vi "电池状态显示.vi"(0 "can卡类型":u8, 1 "设备索引号":u8, 2 "CAN端口":u8, 3 "VIC_Receive":refnum<vi>, 5 "主界面选项 3":enum32{"单选选项1", "单选选项2 2", "单选选项2 3", "单选选项2 4"}(ring)) -> ()   [LabVIEW 2013]
panel:
  out "辅助继电器B(heat)":u16(ring) items=["未闭合", "闭合", "故障", "保留"]
  out "辅助继电器A(fan)":u16(ring) items=["未闭合", "闭合", "故障", "保留"]
  out "标准CAN总线状态":u16(ring) caption="标定CAN模块状态"
  out "Life:":dbl
  out "从板个数":u8
  out "功率":dbl
  out "负绝缘":dbl
  out "正绝缘":dbl
  out "DO":string[](array[string])
  out "DI":string[](array[string])
  out "AI2":dbl
  out "AI1":dbl
  out "放电总安时":dbl
  out "充电总安时":dbl
  out "实际容量":dbl
  out "最大放电电流":dbl
  out "最大充电电流":dbl
  out "平均电流":dbl
  in  "板号":u8
  out "其它故障":string[](array[string])
  out "硬件故障":string[](array[string])
  out "电池系统故障":string[](array[string])
  out "电池故障":string[](array[string])
  out "电池信息":T1
  out "电池应用车型":string
  out "电池包产权标识 3":string
  out "电池包组号 3":string
  out "电池类型 3":string
  out "电池厂商":string
  out "电池生产日期":string
  out "电池充电次数":dbl
  out "电池放空次数 3":dbl
  out "电池充满次数":dbl
  out "电池包累计充电总安时 3":dbl
  out "电池包额定总电压":dbl
  out "电池包额定能量":dbl
  out "电池包额定容量":dbl
  out "电池包累计放电总安时 3":dbl
  out "电池并联 3":dbl
  out "电池串联 3":dbl
  in  "电池信息读取":bool
  out "时间":string
  out "07":dbl
  out "10":string[](array[string])
  out "F":dbl[](array[numeric])
  in  "充电均衡":u32(colorbox)=6618880
  in  "放电均衡":u32(colorbox)=16711680
  out "均衡信息":string[][](table)=[["第1串", "1", "单体检测其它故障", "第25串", "1", "单体检测其它故障", "第49串", "1", "单体检测其它故障", "第73串", "1", "单体检测其它故障", "第97串", "1", "单体检测其它故障", "第121串", "1", "单体检测其它故障", "第145串", "1", "单体检测其它故障", "第169串", "1", "单体检测其它故障", "第193串", "1", "单体检测其它故障", "第217串", "1", "单体检测其它故障", "第241串", "1", "单体检测其它故障", "第265串", "1", "单体检测其它故障", "第289串", "1", "单体检测其它故障", ""], ["第2串", "", "", "第26串", "", "", "第50串", "", "", "第74串", "", "", "第98串", "", "", "第122串", "", "", "第146串", "", "", "第170串", "", "", "第194串", "", "", "第218串", "", "", "第242串", "", "", "第266串", "", "", "第290串", "", "", ""], ["第3串", "", "", "第27串", "", "", "第51串", "", "", "第75串", "", "", "第99串", "", "", "第123串", "", "", "第147串", "", "", "第171串", "", "", "第195串", "", "", "第219串", "", "", "第243串", "", "", "第267串", "", "", "第291串", "", "", ""], ["第4串", "", "", "第28串", "", "", "第52串", "", "", "第76串", "", "", "第100串", "", "", "第124串", "", "", "第148串", "", "", "第172串", "", "", "第196串", "", "", "第220串", "", "", "第244串", "", "", "第268串", "", "", "第292串", "", "", ""], ["第5串", "", "", "第29串", "", "", "第53串", "", "", "第77串", "", "", "第101串", "", "", "第125串", "", "", "第149串", "", "", "第173串", "", "", "第197串", "", "", "第221串", "", "", "第245串", "", "", "第269串", "", "", "第293串", "", "", ""], ["第6串", "", "", "第30串", "", "", "第54串", "", "", "第78串", "", "", "第102串", "", "", "第126串", "", "", "第150串", "", "", "第174串", "", "", "第198串", "", "", "第222串", "", "", "第246串", "", "", "第270串", "", "", "第294串", "", "", ""], ["第7串", "", "", "第31串", "", "", "第55串", "", "", "第79串", "", "", "第103串", "", "", "第127串", "", "", "第151串", "", "", "第175串", "", "", "第199串", "", "", "第223串", "", "", "第247串", "", "", "第271串", "", "", "第295串", "", "", ""], ["第8串", "", "", "第32串", "", "", "第56串", "", "", "第80串", "", "", "第104串", "", "", "第128串", "", "", "第152串", "", "", "第176串", "", "", "第200串", "", "", "第224串", "", "", "第248串", "", "", "第272串", "", "", "第296串", "", "", ""], ["第9串", "", "", "第33串", "", "", "第57串", "", "", "第81串", "", "", "第105串", "", "", "第129串", "", "", "第153串", "", "", "第177串", "", "", "第201串", "", "", "第225串", "", "", "第249串", "", "", "第273串", "", "", "第297串", "", "", ""], ["第10串", "", "", "第34串", "", "", "第58串", "", "", "第82串", "", "", "第106串", "", "", "第130串", "", "", "第154串", "", "", "第178串", "", "", "第202串", "", "", "第226串", "", "", "第250串", "", "", "第274串", "", "", "第298串", "", "", ""], ["第11串", "", "", "第35串", "", "", "第59串", "", "", "第83串", "", "", "第107串", "", "", "第131串", "", "", "第155串", "", "", "第179串", "", "", "第203串", "", "", "第227串", "", "", "第251串", "", "", "第275串", "", "", "第299串", "", "", ""], ["第12串", "", "", "第36串", "", "", "第60串", "", "", "第84串", "", "", "第108串", "", "", "第132串", "", "", "第156串", "", "", "第180串", "", "", "第204串", "", "", "第228串", "", "", "第252串", "", "", "第276串", "", "", "第300串", "", "", ""], ["第13串", "", "", "第37串", "", "", "第61串", "", "", "第85串", "", "", "第109串", "", "", "第133串", "", "", "第157串", "", "", "第181串", "", "", "第205串", "", "", "第229串", "", "", "第253串", "", "", "第277串", "", "", "", "", "", ""], ["第14串", "", "", "第38串", "", "", "第62串", "", "", "第86串", "", "", "第110串", "", "", "第134串", "", "", "第158串", "", "", "第182串", "", "", "第206串", "", "", "第230串", "", "", "第254串", "", "", "第278串", "", "", "", "", "", ""], ["第15串", "", "", "第39串", "", "", "第63串", "", "", "第87串", "", "", "第111串", "", "", "第135串", "", "", "第159串", "", "", "第183串", "", "", "第207串", "", "", "第231串", "", "", "第255串", "", "", "第279串", "", "", "", "", "", ""], ["第16串", "", "", "第40串", "", "", "第64串", "", "", "第88串", "", "", "第112串", "", "", "第136串", "", "", "第160串", "", "", "第184串", "", "", "第208串", "", "", "第232串", "", "", "第256串", "", "", "第280串", "", "", "", "", "", ""], ["第17串", "", "", "第41串", "", "", "第65串", "", "", "第89串", "", "", "第113串", "", "", "第137串", "", "", "第161串", "", "", "第185串", "", "", "第209串", "", "", "第233串", "", "", "第257串", "", "", "第281串", "", "", "", "", "", ""], ["第18串", "", "", "第42串", "", "", "第66串", "", "", "第90串", "", "", "第114串", "", "", "第138串", "", "", "第162串", "", "", "第186串", "", "", "第210串", "", "", "第234串", "", "", "第258串", "", "", "第282串", "", "", "", "", "", ""], ["第19串", "", "", "第43串", "", "", "第67串", "", "", "第91串", "", "", "第115串", "", "", "第139串", "", "", "第163串", "", "", "第187串", "", "", "第211串", "", "", "第235串", "", "", "第259串", "", "", "第283串", "", "", "", "", "", ""], ["第20串", "", "", "第44串", "", "", "第68串", "", "", "第92串", "", "", "第116串", "", "", "第140串", "", "", "第164串", "", "", "第188串", "", "", "第212串", "", "", "第236串", "", "", "第260串", "", "", "第284串", "", "", "", "", "", ""], ["第21串", "", "", "第45串", "", "", "第69串", "", "", "第93串", "", "", "第117串", "", "", "第141串", "", "", "第165串", "", "", "第189串", "", "", "第213串", "", "", "第237串", "", "", "第261串", "", "", "第285串", "", "", "", "", "", ""], ["第22串", "", "", "第46串", "", "", "第70串", "", "", "第94串", "", "", "第118串", "", "", "第142串", "", "", "第166串", "", "", "第190串", "", "", "第214串", "", "", "第238串", "", "", "第262串", "", "", "第286串", "", "", "", "", "", ""], ["第23串", "", "", "第47串", "", "", "第71串", "", "", "第95串", "", "", "第119串", "", "", "第143串", "", "", "第167串", "", "", "第191串", "", "", "第215串", "", "", "第239串", "", "", "第263串", "", "", "第287串", "", "", "", "", "", ""], ["第24串", "", "", "第48串", "", "", "第72串", "", "", "第96串", "", "", "第120串", "", "", "第144串", "", "", "第168串", "", "", "第192串", "", "", "第216串", "", "", "第240串", "", "", "第264串", "", "", "第288串", "", "", "", "", "", ""]]
  out "SOC":string[][](table)=[["第1串", "", "", "第25串", "", "", "第49串", "", "", "第73串", "", "", "第97串", "", "", "第121串", "", "", "第145串", "", "", "第169串", "", "", "第193串", "", "", "第217串", "", "", "第241串", "", "", "第265串", "", "", "第289串", "", "", ""], ["第2串", "", "", "第26串", "", "", "第50串", "", "", "第74串", "", "", "第98串", "", "", "第122串", "", "", "第146串", "", "", "第170串", "", "", "第194串", "", "", "第218串", "", "", "第242串", "", "", "第266串", "", "", "第290串", "", "", ""], ["第3串", "", "", "第27串", "", "", "第51串", "", "", "第75串", "", "", "第99串", "", "", "第123串", "", "", "第147串", "", "", "第171串", "", "", "第195串", "", "", "第219串", "", "", "第243串", "", "", "第267串", "", "", "第291串", "", "", ""], ["第4串", "", "", "第28串", "", "", "第52串", "", "", "第76串", "", "", "第100串", "", "", "第124串", "", "", "第148串", "", "", "第172串", "", "", "第196串", "", "", "第220串", "", "", "第244串", "", "", "第268串", "", "", "第292串", "", "", ""], ["第5串", "", "", "第29串", "", "", "第53串", "", "", "第77串", "", "", "第101串", "", "", "第125串", "", "", "第149串", "", "", "第173串", "", "", "第197串", "", "", "第221串", "", "", "第245串", "", "", "第269串", "", "", "第293串", "", "", ""], ["第6串", "", "", "第30串", "", "", "第54串", "", "", "第78串", "", "", "第102串", "", "", "第126串", "", "", "第150串", "", "", "第174串", "", "", "第198串", "", "", "第222串", "", "", "第246串", "", "", "第270串", "", "", "第294串", "", "", ""], ["第7串", "", "", "第31串", "", "", "第55串", "", "", "第79串", "", "", "第103串", "", "", "第127串", "", "", "第151串", "", "", "第175串", "", "", "第199串", "", "", "第223串", "", "", "第247串", "", "", "第271串", "", "", "第295串", "", "", ""], ["第8串", "", "", "第32串", "", "", "第56串", "", "", "第80串", "", "", "第104串", "", "", "第128串", "", "", "第152串", "", "", "第176串", "", "", "第200串", "", "", "第224串", "", "", "第248串", "", "", "第272串", "", "", "第296串", "", "", ""], ["第9串", "", "", "第33串", "", "", "第57串", "", "", "第81串", "", "", "第105串", "", "", "第129串", "", "", "第153串", "", "", "第177串", "", "", "第201串", "", "", "第225串", "", "", "第249串", "", "", "第273串", "", "", "第297串", "", "", ""], ["第10串", "", "", "第34串", "", "", "第58串", "", "", "第82串", "", "", "第106串", "", "", "第130串", "", "", "第154串", "", "", "第178串", "", "", "第202串", "", "", "第226串", "", "", "第250串", "", "", "第274串", "", "", "第298串", "", "", ""], ["第11串", "", "", "第35串", "", "", "第59串", "", "", "第83串", "", "", "第107串", "", "", "第131串", "", "", "第155串", "", "", "第179串", "", "", "第203串", "", "", "第227串", "", "", "第251串", "", "", "第275串", "", "", "第299串", "", "", ""], ["第12串", "", "", "第36串", "", "", "第60串", "", "", "第84串", "", "", "第108串", "", "", "第132串", "", "", "第156串", "", "", "第180串", "", "", "第204串", "", "", "第228串", "", "", "第252串", "", "", "第276串", "", "", "第300串", "", "", ""], ["第13串", "", "", "第37串", "", "", "第61串", "", "", "第85串", "", "", "第109串", "", "", "第133串", "", "", "第157串", "", "", "第181串", "", "", "第205串", "", "", "第229串", "", "", "第253串", "", "", "第277串", "", "", "", "", "", ""], ["第14串", "", "", "第38串", "", "", "第62串", "", "", "第86串", "", "", "第110串", "", "", "第134串", "", "", "第158串", "", "", "第182串", "", "", "第206串", "", "", "第230串", "", "", "第254串", "", "", "第278串", "", "", "", "", "", ""], ["第15串", "", "", "第39串", "", "", "第63串", "", "", "第87串", "", "", "第111串", "", "", "第135串", "", "", "第159串", "", "", "第183串", "", "", "第207串", "", "", "第231串", "", "", "第255串", "", "", "第279串", "", "", "", "", "", ""], ["第16串", "", "", "第40串", "", "", "第64串", "", "", "第88串", "", "", "第112串", "", "", "第136串", "", "", "第160串", "", "", "第184串", "", "", "第208串", "", "", "第232串", "", "", "第256串", "", "", "第280串", "", "", "", "", "", ""], ["第17串", "", "", "第41串", "", "", "第65串", "", "", "第89串", "", "", "第113串", "", "", "第137串", "", "", "第161串", "", "", "第185串", "", "", "第209串", "", "", "第233串", "", "", "第257串", "", "", "第281串", "", "", "", "", "", ""], ["第18串", "", "", "第42串", "", "", "第66串", "", "", "第90串", "", "", "第114串", "", "", "第138串", "", "", "第162串", "", "", "第186串", "", "", "第210串", "", "", "第234串", "", "", "第258串", "", "", "第282串", "", "", "", "", "", ""], ["第19串", "", "", "第43串", "", "", "第67串", "", "", "第91串", "", "", "第115串", "", "", "第139串", "", "", "第163串", "", "", "第187串", "", "", "第211串", "", "", "第235串", "", "", "第259串", "", "", "第283串", "", "", "", "", "", ""], ["第20串", "", "", "第44串", "", "", "第68串", "", "", "第92串", "", "", "第116串", "", "", "第140串", "", "", "第164串", "", "", "第188串", "", "", "第212串", "", "", "第236串", "", "", "第260串", "", "", "第284串", "", "", "", "", "", ""], ["第21串", "", "", "第45串", "", "", "第69串", "", "", "第93串", "", "", "第117串", "", "", "第141串", "", "", "第165串", "", "", "第189串", "", "", "第213串", "", "", "第237串", "", "", "第261串", "", "", "第285串", "", "", "", "", "", ""], ["第22串", "", "", "第46串", "", "", "第70串", "", "", "第94串", "", "", "第118串", "", "", "第142串", "", "", "第166串", "", "", "第190串", "", "", "第214串", "", "", "第238串", "", "", "第262串", "", "", "第286串", "", "", "", "", "", ""], ["第23串", "", "", "第47串", "", "", "第71串", "", "", "第95串", "", "", "第119串", "", "", "第143串", "", "", "第167串", "", "", "第191串", "", "", "第215串", "", "", "第239串", "", "", "第263串", "", "", "第287串", "", "", "", "", "", ""], ["第24串", "", "", "第48串", "", "", "第72串", "", "", "第96串", "", "", "第120串", "", "", "第144串", "", "", "第168串", "", "", "第192串", "", "", "第216串", "", "", "第240串", "", "", "第264串", "", "", "第288串", "", "", "", "", "", ""]]
  out "内阻":string[][](table)=[["第1串", "", "", "第25串", "", "", "第49串", "", "", "第73串", "", "", "第97串", "", "", "第121串", "", "", "第145串", "", "", "第169串", "", "", "第193串", "", "", "第217串", "", "", "第241串", "", "", "第265串", "", "", "第289串", "", "", ""], ["第2串", "", "", "第26串", "", "", "第50串", "", "", "第74串", "", "", "第98串", "", "", "第122串", "", "", "第146串", "", "", "第170串", "", "", "第194串", "", "", "第218串", "", "", "第242串", "", "", "第266串", "", "", "第290串", "", "", ""], ["第3串", "", "", "第27串", "", "", "第51串", "", "", "第75串", "", "", "第99串", "", "", "第123串", "", "", "第147串", "", "", "第171串", "", "", "第195串", "", "", "第219串", "", "", "第243串", "", "", "第267串", "", "", "第291串", "", "", ""], ["第4串", "", "", "第28串", "", "", "第52串", "", "", "第76串", "", "", "第100串", "", "", "第124串", "", "", "第148串", "", "", "第172串", "", "", "第196串", "", "", "第220串", "", "", "第244串", "", "", "第268串", "", "", "第292串", "", "", ""], ["第5串", "", "", "第29串", "", "", "第53串", "", "", "第77串", "", "", "第101串", "", "", "第125串", "", "", "第149串", "", "", "第173串", "", "", "第197串", "", "", "第221串", "", "", "第245串", "", "", "第269串", "", "", "第293串", "", "", ""], ["第6串", "", "", "第30串", "", "", "第54串", "", "", "第78串", "", "", "第102串", "", "", "第126串", "", "", "第150串", "", "", "第174串", "", "", "第198串", "", "", "第222串", "", "", "第246串", "", "", "第270串", "", "", "第294串", "", "", ""], ["第7串", "", "", "第31串", "", "", "第55串", "", "", "第79串", "", "", "第103串", "", "", "第127串", "", "", "第151串", "", "", "第175串", "", "", "第199串", "", "", "第223串", "", "", "第247串", "", "", "第271串", "", "", "第295串", "", "", ""], ["第8串", "", "", "第32串", "", "", "第56串", "", "", "第80串", "", "", "第104串", "", "", "第128串", "", "", "第152串", "", "", "第176串", "", "", "第200串", "", "", "第224串", "", "", "第248串", "", "", "第272串", "", "", "第296串", "", "", ""], ["第9串", "", "", "第33串", "", "", "第57串", "", "", "第81串", "", "", "第105串", "", "", "第129串", "", "", "第153串", "", "", "第177串", "", "", "第201串", "", "", "第225串", "", "", "第249串", "", "", "第273串", "", "", "第297串", "", "", ""], ["第10串", "", "", "第34串", "", "", "第58串", "", "", "第82串", "", "", "第106串", "", "", "第130串", "", "", "第154串", "", "", "第178串", "", "", "第202串", "", "", "第226串", "", "", "第250串", "", "", "第274串", "", "", "第298串", "", "", ""], ["第11串", "", "", "第35串", "", "", "第59串", "", "", "第83串", "", "", "第107串", "", "", "第131串", "", "", "第155串", "", "", "第179串", "", "", "第203串", "", "", "第227串", "", "", "第251串", "", "", "第275串", "", "", "第299串", "", "", ""], ["第12串", "", "", "第36串", "", "", "第60串", "", "", "第84串", "", "", "第108串", "", "", "第132串", "", "", "第156串", "", "", "第180串", "", "", "第204串", "", "", "第228串", "", "", "第252串", "", "", "第276串", "", "", "第300串", "", "", ""], ["第13串", "", "", "第37串", "", "", "第61串", "", "", "第85串", "", "", "第109串", "", "", "第133串", "", "", "第157串", "", "", "第181串", "", "", "第205串", "", "", "第229串", "", "", "第253串", "", "", "第277串", "", "", "", "", "", ""], ["第14串", "", "", "第38串", "", "", "第62串", "", "", "第86串", "", "", "第110串", "", "", "第134串", "", "", "第158串", "", "", "第182串", "", "", "第206串", "", "", "第230串", "", "", "第254串", "", "", "第278串", "", "", "", "", "", ""], ["第15串", "", "", "第39串", "", "", "第63串", "", "", "第87串", "", "", "第111串", "", "", "第135串", "", "", "第159串", "", "", "第183串", "", "", "第207串", "", "", "第231串", "", "", "第255串", "", "", "第279串", "", "", "", "", "", ""], ["第16串", "", "", "第40串", "", "", "第64串", "", "", "第88串", "", "", "第112串", "", "", "第136串", "", "", "第160串", "", "", "第184串", "", "", "第208串", "", "", "第232串", "", "", "第256串", "", "", "第280串", "", "", "", "", "", ""], ["第17串", "", "", "第41串", "", "", "第65串", "", "", "第89串", "", "", "第113串", "", "", "第137串", "", "", "第161串", "", "", "第185串", "", "", "第209串", "", "", "第233串", "", "", "第257串", "", "", "第281串", "", "", "", "", "", ""], ["第18串", "", "", "第42串", "", "", "第66串", "", "", "第90串", "", "", "第114串", "", "", "第138串", "", "", "第162串", "", "", "第186串", "", "", "第210串", "", "", "第234串", "", "", "第258串", "", "", "第282串", "", "", "", "", "", ""], ["第19串", "", "", "第43串", "", "", "第67串", "", "", "第91串", "", "", "第115串", "", "", "第139串", "", "", "第163串", "", "", "第187串", "", "", "第211串", "", "", "第235串", "", "", "第259串", "", "", "第283串", "", "", "", "", "", ""], ["第20串", "", "", "第44串", "", "", "第68串", "", "", "第92串", "", "", "第116串", "", "", "第140串", "", "", "第164串", "", "", "第188串", "", "", "第212串", "", "", "第236串", "", "", "第260串", "", "", "第284串", "", "", "", "", "", ""], ["第21串", "", "", "第45串", "", "", "第69串", "", "", "第93串", "", "", "第117串", "", "", "第141串", "", "", "第165串", "", "", "第189串", "", "", "第213串", "", "", "第237串", "", "", "第261串", "", "", "第285串", "", "", "", "", "", ""], ["第22串", "", "", "第46串", "", "", "第70串", "", "", "第94串", "", "", "第118串", "", "", "第142串", "", "", "第166串", "", "", "第190串", "", "", "第214串", "", "", "第238串", "", "", "第262串", "", "", "第286串", "", "", "", "", "", ""], ["第23串", "", "", "第47串", "", "", "第71串", "", "", "第95串", "", "", "第119串", "", "", "第143串", "", "", "第167串", "", "", "第191串", "", "", "第215串", "", "", "第239串", "", "", "第263串", "", "", "第287串", "", "", "", "", "", ""], ["第24串", "", "", "第48串", "", "", "第72串", "", "", "第96串", "", "", "第120串", "", "", "第144串", "", "", "第168串", "", "", "第192串", "", "", "第216串", "", "", "第240串", "", "", "第264串", "", "", "第288串", "", "", "", "", "", ""]]
  out "温度表格":string[][](table)=[["第1串", "", "", "第25串", "", "", "第49串", "", "", "第73串", "", "", "第97串", "", "", "第121串", "", "", "第145串", "", "", "第169串", "", "", "第193串", "", "", "第217串", "", "", "第241串", "", "", "第265串", "", "", "第289串", "", "", ""], ["第2串", "", "", "第26串", "", "", "第50串", "", "", "第74串", "", "", "第98串", "", "", "第122串", "", "", "第146串", "", "", "第170串", "", "", "第194串", "", "", "第218串", "", "", "第242串", "", "", "第266串", "", "", "第290串", "", "", ""], ["第3串", "", "", "第27串", "", "", "第51串", "", "", "第75串", "", "", "第99串", "", "", "第123串", "", "", "第147串", "", "", "第171串", "", "", "第195串", "", "", "第219串", "", "", "第243串", "", "", "第267串", "", "", "第291串", "", "", ""], ["第4串", "", "", "第28串", "", "", "第52串", "", "", "第76串", "", "", "第100串", "", "", "第124串", "", "", "第148串", "", "", "第172串", "", "", "第196串", "", "", "第220串", "", "", "第244串", "", "", "第268串", "", "", "第292串", "", "", ""], ["第5串", "", "", "第29串", "", "", "第53串", "", "", "第77串", "", "", "第101串", "", "", "第125串", "", "", "第149串", "", "", "第173串", "", "", "第197串", "", "", "第221串", "", "", "第245串", "", "", "第269串", "", "", "第293串", "", "", ""], ["第6串", "", "", "第30串", "", "", "第54串", "", "", "第78串", "", "", "第102串", "", "", "第126串", "", "", "第150串", "", "", "第174串", "", "", "第198串", "", "", "第222串", "", "", "第246串", "", "", "第270串", "", "", "第294串", "", "", ""], ["第7串", "", "", "第31串", "", "", "第55串", "", "", "第79串", "", "", "第103串", "", "", "第127串", "", "", "第151串", "", "", "第175串", "", "", "第199串", "", "", "第223串", "", "", "第247串", "", "", "第271串", "", "", "第295串", "", "", ""], ["第8串", "", "", "第32串", "", "", "第56串", "", "", "第80串", "", "", "第104串", "", "", "第128串", "", "", "第152串", "", "", "第176串", "", "", "第200串", "", "", "第224串", "", "", "第248串", "", "", "第272串", "", "", "第296串", "", "", ""], ["第9串", "", "", "第33串", "", "", "第57串", "", "", "第81串", "", "", "第105串", "", "", "第129串", "", "", "第153串", "", "", "第177串", "", "", "第201串", "", "", "第225串", "", "", "第249串", "", "", "第273串", "", "", "第297串", "", "", ""], ["第10串", "", "", "第34串", "", "", "第58串", "", "", "第82串", "", "", "第106串", "", "", "第130串", "", "", "第154串", "", "", "第178串", "", "", "第202串", "", "", "第226串", "", "", "第250串", "", "", "第274串", "", "", "第298串", "", "", ""], ["第11串", "", "", "第35串", "", "", "第59串", "", "", "第83串", "", "", "第107串", "", "", "第131串", "", "", "第155串", "", "", "第179串", "", "", "第203串", "", "", "第227串", "", "", "第251串", "", "", "第275串", "", "", "第299串", "", "", ""], ["第12串", "", "", "第36串", "", "", "第60串", "", "", "第84串", "", "", "第108串", "", "", "第132串", "", "", "第156串", "", "", "第180串", "", "", "第204串", "", "", "第228串", "", "", "第252串", "", "", "第276串", "", "", "第300串", "", "", ""], ["第13串", "", "", "第37串", "", "", "第61串", "", "", "第85串", "", "", "第109串", "", "", "第133串", "", "", "第157串", "", "", "第181串", "", "", "第205串", "", "", "第229串", "", "", "第253串", "", "", "第277串", "", "", "", "", "", ""], ["第14串", "", "", "第38串", "", "", "第62串", "", "", "第86串", "", "", "第110串", "", "", "第134串", "", "", "第158串", "", "", "第182串", "", "", "第206串", "", "", "第230串", "", "", "第254串", "", "", "第278串", "", "", "", "", "", ""], ["第15串", "", "", "第39串", "", "", "第63串", "", "", "第87串", "", "", "第111串", "", "", "第135串", "", "", "第159串", "", "", "第183串", "", "", "第207串", "", "", "第231串", "", "", "第255串", "", "", "第279串", "", "", "", "", "", ""], ["第16串", "", "", "第40串", "", "", "第64串", "", "", "第88串", "", "", "第112串", "", "", "第136串", "", "", "第160串", "", "", "第184串", "", "", "第208串", "", "", "第232串", "", "", "第256串", "", "", "第280串", "", "", "", "", "", ""], ["第17串", "", "", "第41串", "", "", "第65串", "", "", "第89串", "", "", "第113串", "", "", "第137串", "", "", "第161串", "", "", "第185串", "", "", "第209串", "", "", "第233串", "", "", "第257串", "", "", "第281串", "", "", "", "", "", ""], ["第18串", "", "", "第42串", "", "", "第66串", "", "", "第90串", "", "", "第114串", "", "", "第138串", "", "", "第162串", "", "", "第186串", "", "", "第210串", "", "", "第234串", "", "", "第258串", "", "", "第282串", "", "", "", "", "", ""], ["第19串", "", "", "第43串", "", "", "第67串", "", "", "第91串", "", "", "第115串", "", "", "第139串", "", "", "第163串", "", "", "第187串", "", "", "第211串", "", "", "第235串", "", "", "第259串", "", "", "第283串", "", "", "", "", "", ""], ["第20串", "", "", "第44串", "", "", "第68串", "", "", "第92串", "", "", "第116串", "", "", "第140串", "", "", "第164串", "", "", "第188串", "", "", "第212串", "", "", "第236串", "", "", "第260串", "", "", "第284串", "", "", "", "", "", ""], ["第21串", "", "", "第45串", "", "", "第69串", "", "", "第93串", "", "", "第117串", "", "", "第141串", "", "", "第165串", "", "", "第189串", "", "", "第213串", "", "", "第237串", "", "", "第261串", "", "", "第285串", "", "", "", "", "", ""], ["第22串", "", "", "第46串", "", "", "第70串", "", "", "第94串", "", "", "第118串", "", "", "第142串", "", "", "第166串", "", "", "第190串", "", "", "第214串", "", "", "第238串", "", "", "第262串", "", "", "第286串", "", "", "", "", "", ""], ["第23串", "", "", "第47串", "", "", "第71串", "", "", "第95串", "", "", "第119串", "", "", "第143串", "", "", "第167串", "", "", "第191串", "", "", "第215串", "", "", "第239串", "", "", "第263串", "", "", "第287串", "", "", "", "", "", ""], ["第24串", "", "", "第48串", "", "", "第72串", "", "", "第96串", "", "", "第120串", "", "", "第144串", "", "", "第168串", "", "", "第192串", "", "", "第216串", "", "", "第240串", "", "", "第264串", "", "", "第288串", "", "", "", "", "", ""]]
  out "电压表格控件":string[][](table)=[["第1串", "", "", "第25串", "", "", "第49串", "", "", "第73串", "", "", "第97串", "", "", "第121串", "", "", "第145串", "", "", "第169串", "", "", "第193串", "", "", "第217串", "", "", "第241串", "", "", "第265串", "", "", "第289串", "", "", ""], ["第2串", "", "", "第26串", "", "", "第50串", "", "", "第74串", "", "", "第98串", "", "", "第122串", "", "", "第146串", "", "", "第170串", "", "", "第194串", "", "", "第218串", "", "", "第242串", "", "", "第266串", "", "", "第290串", "", "", ""], ["第3串", "", "", "第27串", "", "", "第51串", "", "", "第75串", "", "", "第99串", "", "", "第123串", "", "", "第147串", "", "", "第171串", "", "", "第195串", "", "", "第219串", "", "", "第243串", "", "", "第267串", "", "", "第291串", "", "", ""], ["第4串", "", "", "第28串", "", "", "第52串", "", "", "第76串", "", "", "第100串", "", "", "第124串", "", "", "第148串", "", "", "第172串", "", "", "第196串", "", "", "第220串", "", "", "第244串", "", "", "第268串", "", "", "第292串", "", "", ""], ["第5串", "", "", "第29串", "", "", "第53串", "", "", "第77串", "", "", "第101串", "", "", "第125串", "", "", "第149串", "", "", "第173串", "", "", "第197串", "", "", "第221串", "", "", "第245串", "", "", "第269串", "", "", "第293串", "", "", ""], ["第6串", "", "", "第30串", "", "", "第54串", "", "", "第78串", "", "", "第102串", "", "", "第126串", "", "", "第150串", "", "", "第174串", "", "", "第198串", "", "", "第222串", "", "", "第246串", "", "", "第270串", "", "", "第294串", "", "", ""], ["第7串", "", "", "第31串", "", "", "第55串", "", "", "第79串", "", "", "第103串", "", "", "第127串", "", "", "第151串", "", "", "第175串", "", "", "第199串", "", "", "第223串", "", "", "第247串", "", "", "第271串", "", "", "第295串", "", "", ""], ["第8串", "", "", "第32串", "", "", "第56串", "", "", "第80串", "", "", "第104串", "", "", "第128串", "", "", "第152串", "", "", "第176串", "", "", "第200串", "", "", "第224串", "", "", "第248串", "", "", "第272串", "", "", "第296串", "", "", ""], ["第9串", "", "", "第33串", "", "", "第57串", "", "", "第81串", "", "", "第105串", "", "", "第129串", "", "", "第153串", "", "", "第177串", "", "", "第201串", "", "", "第225串", "", "", "第249串", "", "", "第273串", "", "", "第297串", "", "", ""], ["第10串", "", "", "第34串", "", "", "第58串", "", "", "第82串", "", "", "第106串", "", "", "第130串", "", "", "第154串", "", "", "第178串", "", "", "第202串", "", "", "第226串", "", "", "第250串", "", "", "第274串", "", "", "第298串", "", "", ""], ["第11串", "", "", "第35串", "", "", "第59串", "", "", "第83串", "", "", "第107串", "", "", "第131串", "", "", "第155串", "", "", "第179串", "", "", "第203串", "", "", "第227串", "", "", "第251串", "", "", "第275串", "", "", "第299串", "", "", ""], ["第12串", "", "", "第36串", "", "", "第60串", "", "", "第84串", "", "", "第108串", "", "", "第132串", "", "", "第156串", "", "", "第180串", "", "", "第204串", "", "", "第228串", "", "", "第252串", "", "", "第276串", "", "", "第300串", "", "", ""], ["第13串", "", "", "第37串", "", "", "第61串", "", "", "第85串", "", "", "第109串", "", "", "第133串", "", "", "第157串", "", "", "第181串", "", "", "第205串", "", "", "第229串", "", "", "第253串", "", "", "第277串", "", "", "", "", "", ""], ["第14串", "", "", "第38串", "", "", "第62串", "", "", "第86串", "", "", "第110串", "", "", "第134串", "", "", "第158串", "", "", "第182串", "", "", "第206串", "", "", "第230串", "", "", "第254串", "", "", "第278串", "", "", "", "", "", ""], ["第15串", "", "", "第39串", "", "", "第63串", "", "", "第87串", "", "", "第111串", "", "", "第135串", "", "", "第159串", "", "", "第183串", "", "", "第207串", "", "", "第231串", "", "", "第255串", "", "", "第279串", "", "", "", "", "", ""], ["第16串", "", "", "第40串", "", "", "第64串", "", "", "第88串", "", "", "第112串", "", "", "第136串", "", "", "第160串", "", "", "第184串", "", "", "第208串", "", "", "第232串", "", "", "第256串", "", "", "第280串", "", "", "", "", "", ""], ["第17串", "", "", "第41串", "", "", "第65串", "", "", "第89串", "", "", "第113串", "", "", "第137串", "", "", "第161串", "", "", "第185串", "", "", "第209串", "", "", "第233串", "", "", "第257串", "", "", "第281串", "", "", "", "", "", ""], ["第18串", "", "", "第42串", "", "", "第66串", "", "", "第90串", "", "", "第114串", "", "", "第138串", "", "", "第162串", "", "", "第186串", "", "", "第210串", "", "", "第234串", "", "", "第258串", "", "", "第282串", "", "", "", "", "", ""], ["第19串", "", "", "第43串", "", "", "第67串", "", "", "第91串", "", "", "第115串", "", "", "第139串", "", "", "第163串", "", "", "第187串", "", "", "第211串", "", "", "第235串", "", "", "第259串", "", "", "第283串", "", "", "", "", "", ""], ["第20串", "", "", "第44串", "", "", "第68串", "", "", "第92串", "", "", "第116串", "", "", "第140串", "", "", "第164串", "", "", "第188串", "", "", "第212串", "", "", "第236串", "", "", "第260串", "", "", "第284串", "", "", "", "", "", ""], ["第21串", "", "", "第45串", "", "", "第69串", "", "", "第93串", "", "", "第117串", "", "", "第141串", "", "", "第165串", "", "", "第189串", "", "", "第213串", "", "", "第237串", "", "", "第261串", "", "", "第285串", "", "", "", "", "", ""], ["第22串", "", "", "第46串", "", "", "第70串", "", "", "第94串", "", "", "第118串", "", "", "第142串", "", "", "第166串", "", "", "第190串", "", "", "第214串", "", "", "第238串", "", "", "第262串", "", "", "第286串", "", "", "", "", "", ""], ["第23串", "", "", "第47串", "", "", "第71串", "", "", "第95串", "", "", "第119串", "", "", "第143串", "", "", "第167串", "", "", "第191串", "", "", "第215串", "", "", "第239串", "", "", "第263串", "", "", "第287串", "", "", "", "", "", ""], ["第24串", "", "", "第48串", "", "", "第72串", "", "", "第96串", "", "", "第120串", "", "", "第144串", "", "", "第168串", "", "", "第192串", "", "", "第216串", "", "", "第240串", "", "", "第264串", "", "", "第288串", "", "", "", "", "", ""]]
  out "故障定义":string[][](table)=[["电池故障定义", "状态", "BMS故障定义", "状态", "电池系统故障定义", "状态", "其他故障定义", "状态"], ["总电压过压", "失效", "电压检测模块故障", "保留", "正接触器粘连", "保留", "下电故障", "二级故障"], ["总电压欠压", "失效", "温度检测模块故障", "保留", "正接触器不能吸合", "保留", "供电电源过压", "二级故障"], ["单体电压过压", "失效", "电池检测模块故障", "保留", "带电流切断总正继电器故障", "保留", "供电电源欠压", "二级故障"], ["单体电压欠压", "失效", "绝缘检测模块故障", "正常", "带电流切断总负继电器故障", "保留", "风机继电器粘连", "二级故障"], ["单箱压差过大", "失效", "内总电压检测模块故障", "保留", "负接触器粘连", "保留", "风机继电器不能吸合", "失效"], ["整组压差过大", "失效", "外总电压检测模块故障", "保留", "负接触器不能吸合", "保留", "液位传感器", "失效"], ["单箱温差过大", "失效", "系统外扩时钟模块故障", "正常", "预充电接触器粘连", "保留", "压力传感器报警", "失效"], ["整组温差过大", "失效", "CPU内部EE故障", "保留", "预充电接触器不能吸合", "保留", "碰撞传感器报警", "失效"], ["温度过高", "失效", "EE存储器故障", "保留", "DC/DC继电器粘连", "保留", "湿度传感器报警", ""], ["温度过低", "失效", "45db041存储器故障", "保留", "DC/DC继电器不能吸合", "保留", "烟雾报警器故障", ""], ["充电电流过高", "失效", "CPU内部flash存储器故障", "保留", "高压互锁失效", "保留", "保险丝温度高于上限值", ""], ["放电电流过高", "失效", "CPU故障", "保留", "高压互锁异常", "保留", "保险丝损坏", ""], ["回馈过电流", "失效", "CAN4通信模块故障", "保留", "充电接触器粘连", "保留", "绝缘故障偏正极", "失效"], ["SOC过高", "正常", "CAN0通信模块故障", "保留", "充电接触器不能吸合", "保留", "绝缘故障偏负极", "失效"], ["SOC过低", "失效", "CAN1通信模块故障", "正常", "带电流切断充电继电器故障", "保留", "绝缘故障中间侧", "失效"], ["单体SOC过高", "失效", "CAN2通信模块故障", "正常", "极注温度高于上限值", "保留", "绝缘故障(未分位置", "失效"], ["单体SOC过低", "失效", "CAN3通信模块故障", "保留", "预充电故障", "保留", "", ""], ["单体SOC不一致", "失效", "以太网通信模块故障", "保留", "风机堵路", "正常", "", ""], ["箱间平均电压不一致", "失效", "RS232通信模块故障", "保留", "风机开路", "正常", "", ""], ["电池组号不一致", "失效", "RS485通信模块故障", "保留", "加热不能开启", "正常", "", ""], ["单体电池内阻大", "失效", "充电均衡模块故障", "正常", "加热不能关闭", "保留", "", ""], ["单体电池内阻不一致", "失效", "放电均衡模块故障", "正常", "加热器温度高于上限值", "保留", "", ""], ["电池组内阻大", "失效", "WH计量模块故障", "正常", "进风口温度过高", "保留", "", ""], ["箱间SOC不一致", "失效", "软件故障", "正常", "进风口,出风口温差故障", "保留", "", ""], ["电池厂家不一致", "失效", "AI自检异常", "正常", "出风口温度过高", "保留", "", ""], ["电池类型不一致", "失效", "AO自检异常", "正常", "出风口过低", "保留", "", ""], ["电池内短路", "失效", "DI模块故障", "正常", "", "", "", ""], ["整体电池容量低", "失效", "DO模块故障", "正常", "", "", "", ""], ["单体电池容量低", "失效", "", "", "", "", "", ""], ["单体电池容量不一致", "", "", "", "", "", "", ""], ["", "", "", "", "", "", "", ""], ["", "", "", "", "", "", "", ""]] caption="故障信息"
  out "BMS信息":string[][](table)=[["参数名称", "周期刷新", "参数名称", "周期刷新", "参数名称", "单次刷新"], ["温度检测模块状态", "", "BMS唤醒模式", "", "软件版本号", ""], ["电池充电均衡模块状态", "", "Key_on", "", "平台版本号", ""], ["电池放电均衡模块状态", "", "慢充", "", "各功能模块版本号", ""], ["电压检测模式状态", "", "快充", "", "内部CAN通讯协议版本", ""], ["绝缘检测模块状态", "", "自唤醒", "", "硬件版本号", ""], ["电池检测模块状态", "", "CAN唤醒", "", "温度传感器类型", ""], ["内部总电压检测模块状态", "", "自保持输出状态", "", "电流传感器类型", ""], ["外部总电压检测模块状态", "", "内部CAN总线状态", "", "历史记录起始页", ""], ["系统时钟状态", "", "充电CAN总线状态", "", "历史记录终止页", ""], ["Flash存储器状态", "", "整车CAN总线状态", "", "故障记录起始页", ""], ["外部EE存储器状态", "", "BMS上次停机时间", "", "故障记录终止页", ""], ["内部EE存储器状态", "", "BMS当前系统时间", "", "", ""], ["BMS供电电源状态", "", "", "", "", ""], ["BMS钥匙信号状态", "", "", "", "", ""], ["BMS供电电源电压", "", "", "", "", ""], ["内网总线负载率", "", "", "", "", ""], ["", "", "", "", "", ""], ["", "", "", "", "", ""], ["", "", "", "", "", ""], ["", "", "", "", "", ""], ["", "", "", "", "", ""]] caption="BMS信息界面"
  in  "主界面选项":enum32{"单选选项1", "单选选项2 2", "单选选项2 3", "单选选项2 4"}(radio)
  out "充电信息":string[][](table)=[["参数名称", "周期刷新", "参数名称", "周期刷新", "参数名称", ""], ["充电允许控制状态", "禁止充电", "BMS停止充电原因", "2345", "累计充电时间", ""], ["快/慢充电信号状态", "消失", "达到所需单体电压设定值", "0", "剩余充电时间", ""], ["交流充电接口容量", "32A", "达到总电压设定值", "300", "最大允许充电总电压", ""], ["充电接口连接状态", "不连接", "达到所需SOC目标值", "3.7", "最大允许充电单体电压", ""], ["充电状态", "空闲", "BMS有硬件故障", "670", "最大允许充电电流", ""], ["充电阶段", "", "系统存在绝缘故障", "3500", "最小允许充电电流", ""], ["充电机状态", "", "单体电压超过上限", "0", "充电电流步长", ""], ["充电机停止充电原因", "", "单体电压过低", "23000", "最大允许充电温度", ""], ["达到充电机设定条件中止", "", "总电压超过上限", "300", "充电机输出电压", ""], ["人工中止", "", "总电压过低", "30000", "充电机输出电流", ""], ["故障中止", "", "电池温度过高", "4560", "充电机累计输出能量", ""], ["充电机故障代码", "", "电池温度过低", "", "", ""], ["充电机过温", "", "充电电流超限", "", "", ""], ["充电连接器故障", "", "电池不匹配", "", "", ""], ["充电机内部过温", "", "电池己充满", "", "", ""], ["所需电量不能传送", "", "充电继电器故障", "", "", ""], ["充电机急停故障", "", "输出连接器故障", "", "", ""], ["电压异常", "", "充电连接器故障", "", "", ""], ["电流不匹配", "", "充电通信超时", "", "", ""], ["其他故障", "", "辅助电源故障", "", "", ""], ["", "", "烟雾报警", "", "", ""], ["", "", "其他故障", "", "", ""], ["", "", "", "", "", ""]] caption="BMS信息界面"
  in  "电池信息选项":enum16{"电池信息", "历史信息"}(ring)
  out "电池系统信息":string[][](table)=[["参数名称", "周期刷新", "参数名称", "单次刷新", "参数名称", "单次刷新", "参数名称", "单次刷新"], ["严重故障干接点", "", "电池串联数", "", "历史最高电压", "", "历史最大充电功率", ""], ["加热器状态", "", "电池并联数", "", "历史最低电压", "", "历史最大放电功率", ""], ["风机状态", "", "电池生产厂商", "", "历史电池电压极差", "", "历史最大充电电流", ""], ["液位传感器状态", "", "电池类型", "", "历史最高平均电压", "", "历史最大放电电流", ""], ["电池箱锁止机构状态", "", "电池包生产日期", "", "历史最低平均电压", "", "电池组工作电流分布", ""], ["烟雾报警器状态", "", "电池包额定能量", "", "历史最高端电压", "", "电池组SOC分布", ""], ["维护开关状态", "", "电池包额定容量", "", "历史最低端电压", "", "电池总充电安时", ""], ["高压互锁状态", "", "电池包额定总电压", "", "历史最高温度", "", "电池总放电安时", ""], ["碰撞开关状态", "", "电池包产权标识", "", "历史最低温度", "", "电池剩余容量", ""], ["手动维护状态", "", "", "", "历史电池温度极差", "", "", ""], ["温度传感器状态", "", "电池包应用车型", "", "历史最高平均温度", "", "", ""], ["压力传感器状态", "", "正极接触器寿命", "", "历史最低平均温度", "", "", ""], ["风机转速", "", "负极接触器寿命", "", "平均温度分布", "", "", ""], ["预充电时间", "", "预充电接触器寿命", "", "最低温度分布", "", "", ""], ["", "", "充电接触器寿命", "", "最高温度分布", "", "", ""], ["", "", "车辆VIN号", "", "最大极差温度分布", "", "", ""], ["", "", "电池放空次数", "", "", "", "", ""], ["", "", "充满次数", "", "", "", "", ""], ["", "", "充电次数", "", "", "", "", ""], ["", "", "", "", "", "", "", ""], ["", "", "", "", "", "", "", ""], ["", "", "", "", "", "", "", ""], ["", "", "", "", "", "", "", ""]] caption="BMS信息界面"
  out "主界面详细信息":string[][](table)=[["平均电流", "", "辅助继电器A"], ["最大充电电流", "", "辅助继电器B"], ["最大放电电流", "", "DO1"], ["实际容量", "", "DO2"], ["充电总安时", "", "DI1"], ["放电总安时", "", "DI2"], ["正绝缘电阻", "", "DI3"], ["负绝缘电阻", "", "DI4"], ["功率", "", "协议版本号"], ["从板个数", "", "应用类型"], ["AI1", "", "波特率"], ["AI2", "", "协议是否公开"], ["", "", ""], ["", "", ""]]
  out "位置":dbl[](array[numeric])
  out "输出数据":dbl[](array[numeric])
  out "详细信息":T2
  out "继电器颜色":u32[](array[colorbox])
  out "命令序号":u8
  in  "命令":u32=133
  out "列1颜色 2":u32[](array[colorbox])
  out "电池信息解析":dbl[](array[numeric])
  out "列1":dbl[](array[numeric])
  out "列3":T3
  out "结束信号":bool
  out "输出数组":u8[](array[numeric])
  out "错误代码":i32
  in  "VCI_Receive":T4 {"Rsv3" max=0 format="%x"; "Rsv2" min=101 format="%x"; "Rsv1" format="%x"; "Data8" format="%x"; "Data7" format="%x"; "Data6" format="%x"; "Data5" format="%x"; "Data4" format="%x"; "Data3" format="%x"; "Data2" format="%x"; "Data1" format="%x"; "DataLen" format="%x"; "ExternFlag" format="%x"; "RemoteFlag" format="%x"; "SendType" format="%x"; "TimeFlag" format="%x"; "TimeStamp" format="%x"; "ID" format="%x"}
  out "状态":bool=TRUE
  in  "停止":bool=TRUE
  in  "选项卡控件":enum32{"电池系统信息", "BMS信息", "充电信息", "故障信息"}(tab)
  out "外总压(V)":dbl(knob) scale=0.0..800.0
  out "风机转速":dbl
  out "预充电时间":dbl
  out "碰撞开关状态":u16(ring) items=["正常", "异常", "保留", "无效"]
  out "手动维护开关":u16(ring) items=["正常", "异常", "保留", "无效"]
  out "湿度传感器状态":u16(ring) items=["正常", "异常", "保留", "无效"]
  out "压力传感器状态":u16(ring) items=["正常", "异常", "保留", "无效"]
  out "电池箱锁止机构状态":u16(ring) items=["正常", "异常", "保留", "无效"]
  out "烟雾报警器状态":u16(ring) items=["正常", "异常", "保留", "无效"]
  out "维护开关状态":u16(ring) items=["正常", "异常", "保留", "无效"]
  out "高压互锁状态":u16(ring) items=["正常", "异常", "保留", "无效"]
  out "液位传感器状态":u16(ring) items=["正常", "异常", "保留", "无效"]
  out "风机状态":u16(ring) items=["闭合", "断开", "故障", "无效"]
  out "加热器状态":u16(ring) items=["闭合", "断开", "故障", "无效"]
  out "严重故障干接点":u16(ring) items=["闭合", "断开", "故障", "无效"]
  out "主界面其他信息":T5 {"放电总安时(Ah)" format="%#_12f"; "负绝缘电阻(kΩ)" format="%#_12f"; "实际容量(Ah)" format="%#.3f"; "充电总安时(Ah)" format="%#_12f"; "正绝缘电阻(kΩ)" format="%#_12f"}
  out "慢充":string="未唤醒"
  out "快充":string="未唤醒"
  out "自唤醒":string="未唤醒"
  out "CAN唤醒":string="未唤醒"
  out "Key_on":string="未唤醒"
  out "当前系统时间":string
  out "BMS当前系统时间2":string
  out "BMS当前系统时间2 2":string
  out "上次停机时间":string
  out "供电电源电压(V)":string="0"
  in  "保留":u16(ring)
  in  "故障":u16(ring)
  in  "闭合":u16(ring)
  in  "未闭合":u16(ring)
  in  "欠压":u16(ring)
  in  "过压":u16(ring)
  in  "无效":u16(ring)
  in  "故障":u16(ring)
  in  "正常":u16(ring)
  out "内网总线负载率":string="0"
  out "供电电源状态":u16(ring)
  out "充电CAN总线状态":u16(ring) caption="充电CAN模块状态"
  out "整车CAN总线状态":u16(ring) caption="整车CAN模块状态"
  out "内部CAN总线状态":u16(ring) caption="内部CAN模块状态"
  out "Flash存储器状态":u16(ring)
  out "外部EE存储器状态":u16(ring)
  out "内部EE存储器状态":u16(ring)
  out "系统时钟状态":u16(ring)
  out "内部总电压检测模块状态":u16(ring)
  out "外部总电压检测模块状态":u16(ring)
  out "绝缘检测模块状态":u16(ring)
  out "电流模块模块状态":u16(ring) caption="电流检测模块状态"
  out "电池充电均衡模块状态":u16(ring)
  out "电池放电均衡模块状态":u16(ring)
  out "温度模块检测状态":u16(ring) caption="温度检测模块状态"
  out "电压模块检测状态":u16(ring) caption="电压检测模块状态"
  out "下拉列表":u16(ring) caption="充电状态2"
  out "充电状态":u16(ring) items=["空闲", "充电", "充满", "故障"]
  out "检测点2 CC2(V)":dbl
  out "检测点4 CC(V)":dbl
  out "PWM检测点3 CP(%)":dbl caption="PWM3 CP(%)"
  out "充电电流步长":dbl
  out "最小允许充电电流(A)":dbl
  out "最大允许充电电流(A)":dbl
  out "最高允许充电单体电压(A)":dbl
  out "最高允许充电总电压(A)":dbl
  out "最高允许充电温度(℃)":dbl
  out "剩余充电时间(min)":dbl
  out "BMS中止\n充电原因":string
  out "累计充电时间(min)":dbl
  out "充电机累计输出能量(kW)":string="0"
  out "充电机输出电流(A)":T6="0"
  out "充电机输出电压(V)":string="0"
  out "充电机中止充电原因":string
  out "充电机 故障代码":string="充电机 故障代码"
  out "慢充电信号状态":string="消失"
  out "交流充电接口容量":string="无效"
  out "充电允许控制状态":string="禁止充电"
  out "充电接口连接状态":string="不连接"
  out "充电阶段":string="无效"
  out "充电机状态":string="正常"
  out "三级故障":bool=TRUE
  out "二级故障":bool
  out "一级故障":bool=TRUE
  in  "故障信息选择按键":T7(radio)
  out "二级故障 4":bool
  out "二级故障 3":bool
  out "二级故障 2":bool
  in  "故障信息":T8(tab)=enum."BMS故障"
  out "电池故障":string[][](array[string])
  out "硬件故障 2":string[][](array[string])
  out "硬件故障 2":string[][](array[string])
  out "其他故障":string[][](array[string])
  in  "其他故障":string[][](array[string])
  in  "状态选择":T9(ring)
  in  "读取其它状态":bool
  out "电池故障显示":bool
  out "电池系统故障显示":bool
  out "BMS故障显示":bool
  out "二级故障 5":bool
  out "其他故障显示":bool
  out "单选选项2":bool
  # "主板详细信息"
  # "主板详细信息"
  # "监控上位机"
  # "图例"
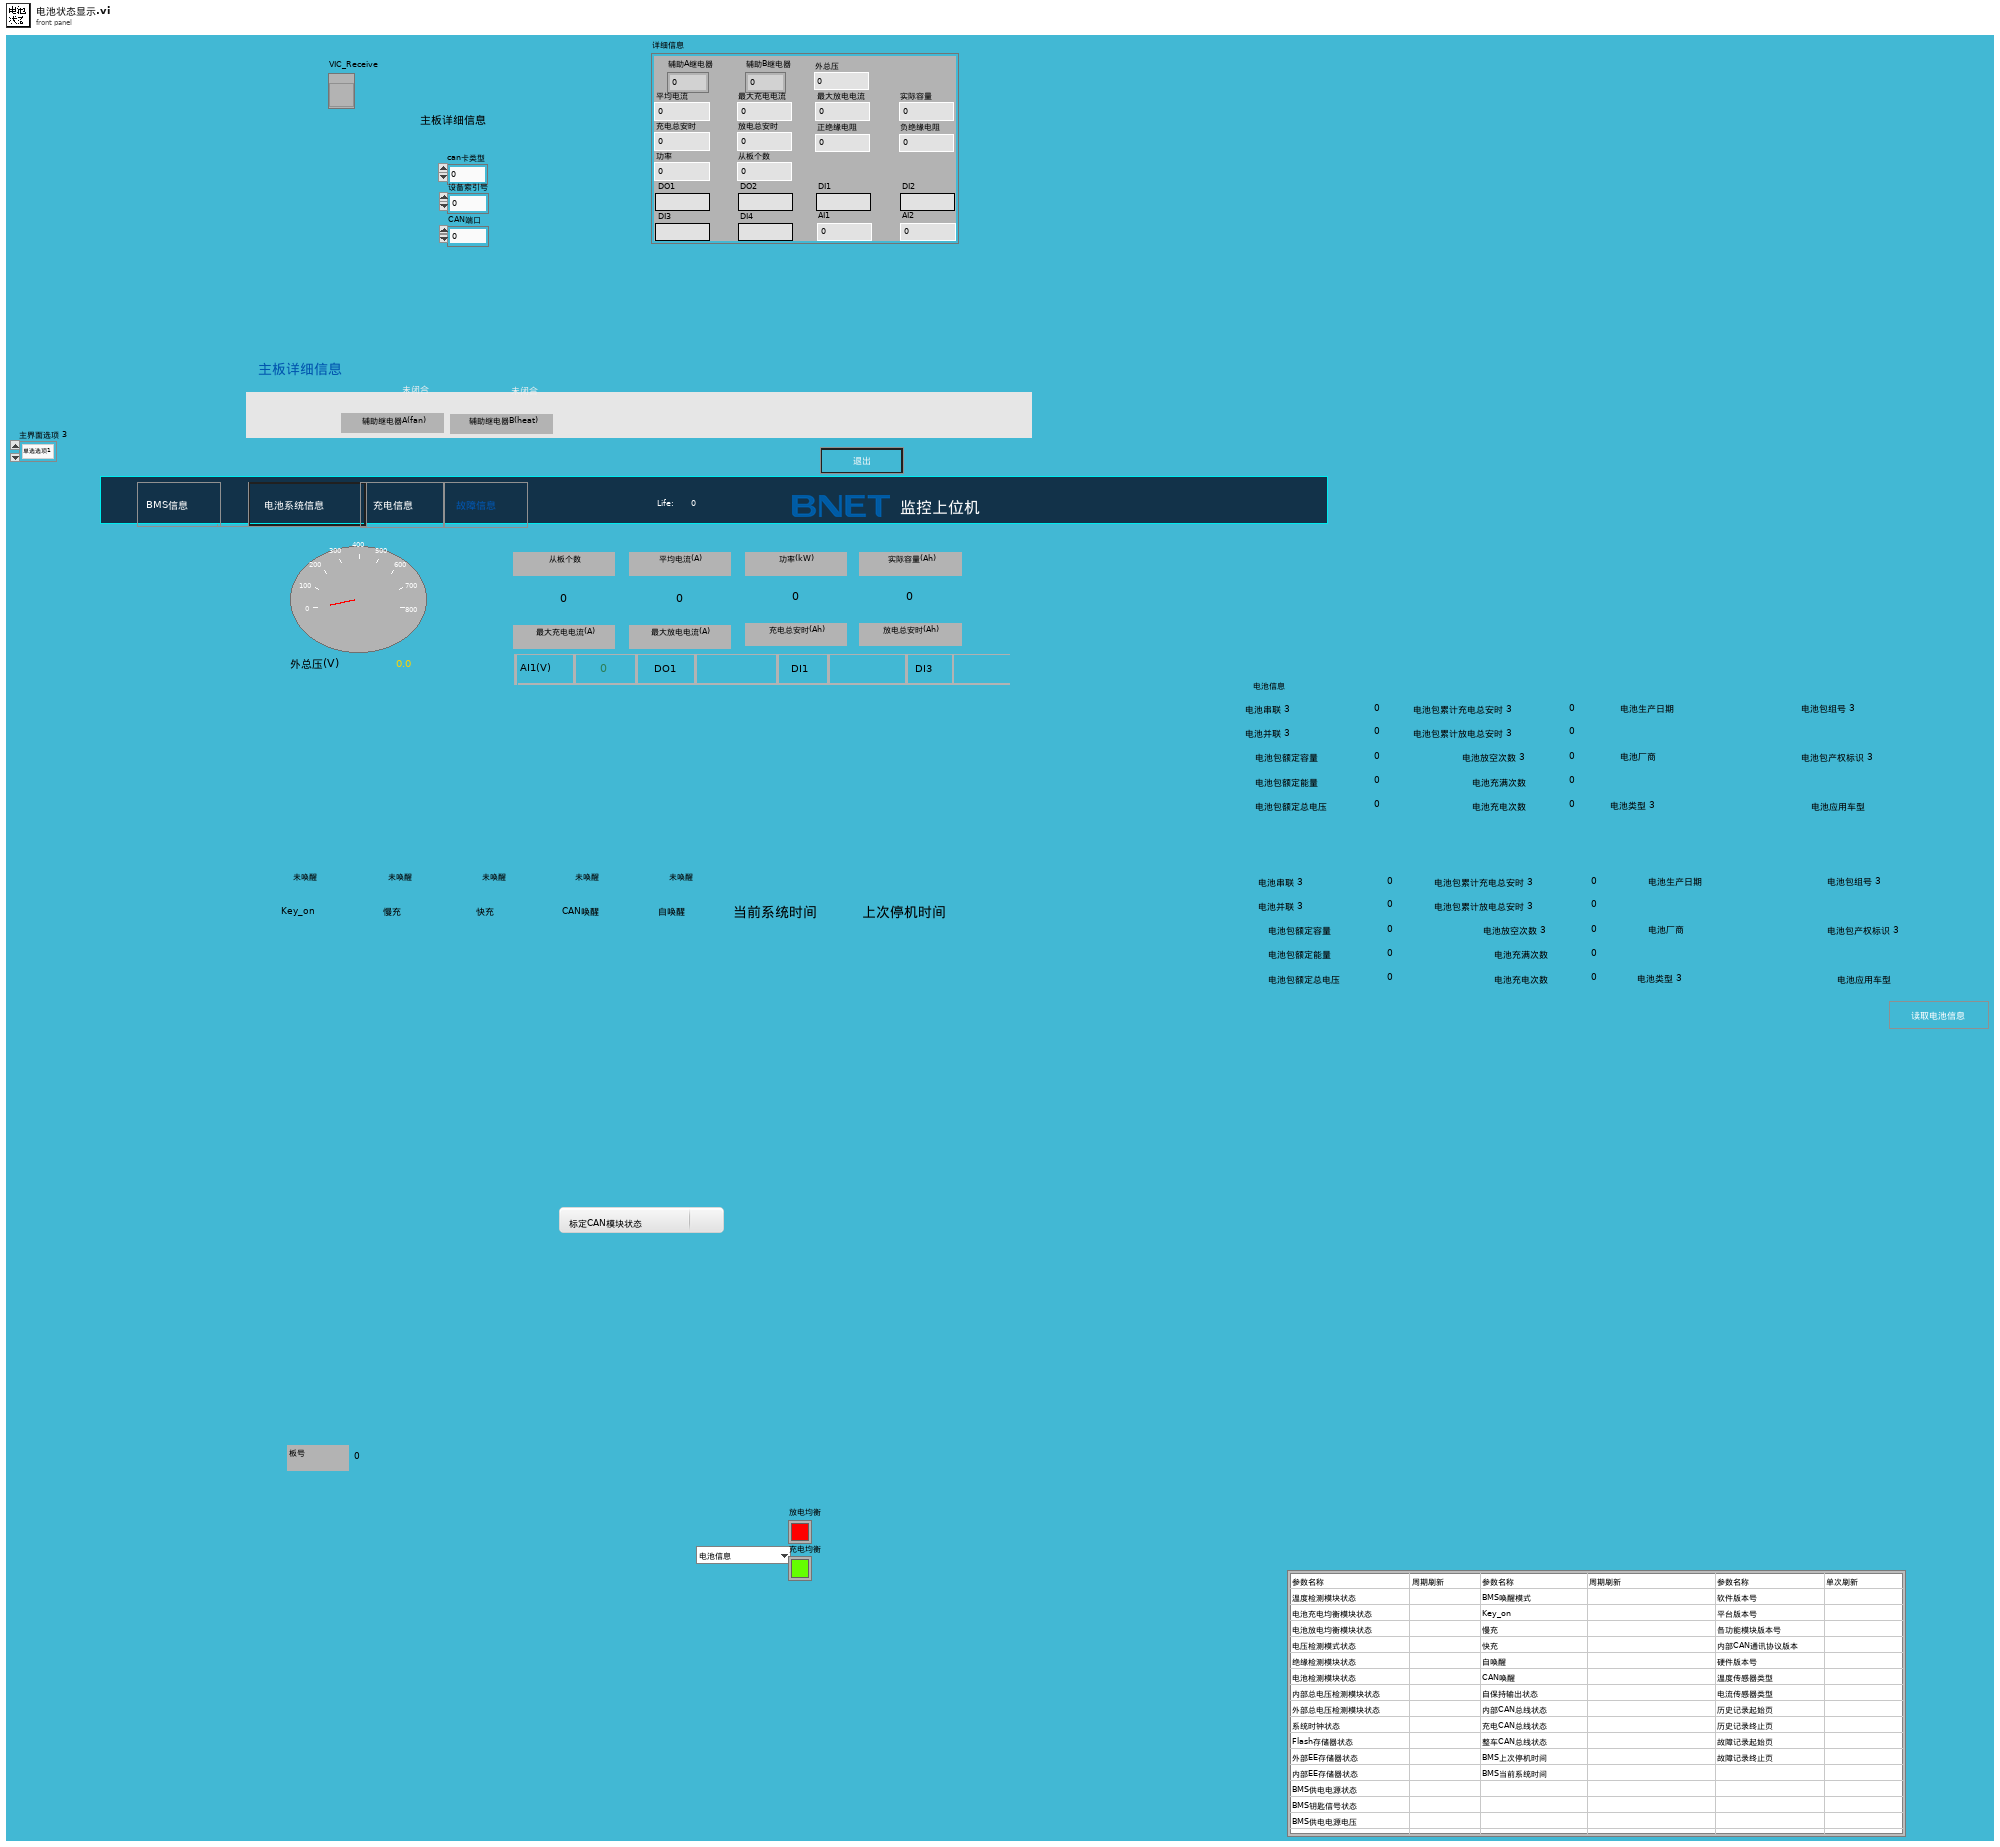
[diagram p1: front panel]
types:
  T1 = cluster{"电池串联 3":dbl, "电池并联 3":dbl, "电池包累计放电总安时 3":dbl, "电池包额定容量":dbl, "电池包额定能量":dbl, "电池包额定总电压":dbl, "电池包累计充电总安时 3":dbl, "电池充满次数":dbl, "电池放空次数 3":dbl, "电池充电次数":dbl, "电池生产日期":string, "电池厂商":string, "电池类型 3":string, "电池包组号 3":string, "电池包产权标识 3":string, "电池应用车型":string}
  T2 = cluster{"平均电流":dbl, "最大充电电流":dbl, "最大放电电流":dbl, "实际容量":dbl, "充电总安时":dbl, "放电总安时":dbl, "正绝缘电阻":dbl, "负绝缘电阻":dbl, "功率":dbl, "从板个数":dbl, "辅助A继电器":dbl, "辅助B继电器":dbl, "DO1":string, "DO2":string, "DI1":string, "DI2":string, "DI3":string, "DI4":string, "AI1":dbl, "AI2":dbl, "外总压":dbl}
  T3 = cluster{"累计充电时间":dbl, "剩余充电时间":dbl, "最大允许充电总电压":dbl, "最大允许充电单体电压":dbl, "最大允许充电电流":dbl, "最小允许充电电流":dbl, "充电电流步长":dbl, "最大允许充电温度":dbl, "充电机输出电压":dbl, "充电机输出电流":dbl, "充电机累计输出能量":dbl}
  T4 = cluster{"ID":u32, "TimeStamp":u32, "TimeFlag":u8, "SendType":u8, "RemoteFlag":u8, "ExternFlag":u8, "DataLen":u8, "Data1":u8, "Data2":u8, "Data3":u8, "Data4":u8, "Data5":u8, "Data6":u8, "Data7":u8, "Data8":u8, "Rsv1":u8, "Rsv2":u8, "Rsv3":u8}
  T5 = cluster{"平均电流(A)":dbl, "最大充电电流(A)":dbl, "最大放电电流(A)":dbl, "实际容量(Ah)":dbl, "充电总安时(Ah)":dbl, "放电总安时(Ah)":dbl, "正绝缘电阻(kΩ)":dbl, "负绝缘电阻(kΩ)":dbl, "功率(kW)":dbl, "从板个数":dbl, "DO1":string, "DO2":string, "DI1":string, "DI2":string, "DI3":string, "DI4":string, "AI1(V)":dbl, "AI2(V)":dbl}
  T6 = typedef "控件 1.ctl" = string
  T7 = enum32{"单选选项2", "单选选项2 2", "单选选项2 3", "单选选项1", "单选选项2 4"}
  T8 = enum32{"电池故障", "BMS故障", "电池系统故障", "其他故障", "其他状态"}
  T9 = enum16{"电压检测,内总电压检测,外总电压检测,温度检测,电流检测,绝缘检测", "内部EE存储器,外部EE存储器,外部FLASH存储器", "CAN检测", "CPU,软件", "RS485,RS232检测", "DI,DO,AI,AO检测", "预充电故障,电池不匹配,充电异常故障"}
  T10 = enum16{"电压检测", "外总电压检测", "内总电压检测", "温度检测", "电流检测", "绝缘检测", "CAN0检测", "CAN1检测", "CAN4检测", "CAN2检测", "CAN3检测", "RS485检测", "RS232检测", "内部EE存储器", "外部EE存储器", "外部Flash存储器", "CPU", "软件", "DI", "DO", "AI", "AO", "预充电故障", "电池不匹配", "充电异常"}
  T11 = enum32{"Invalid", "Standard", "Closed", "Hidden", "Minimized", "Maximized"}
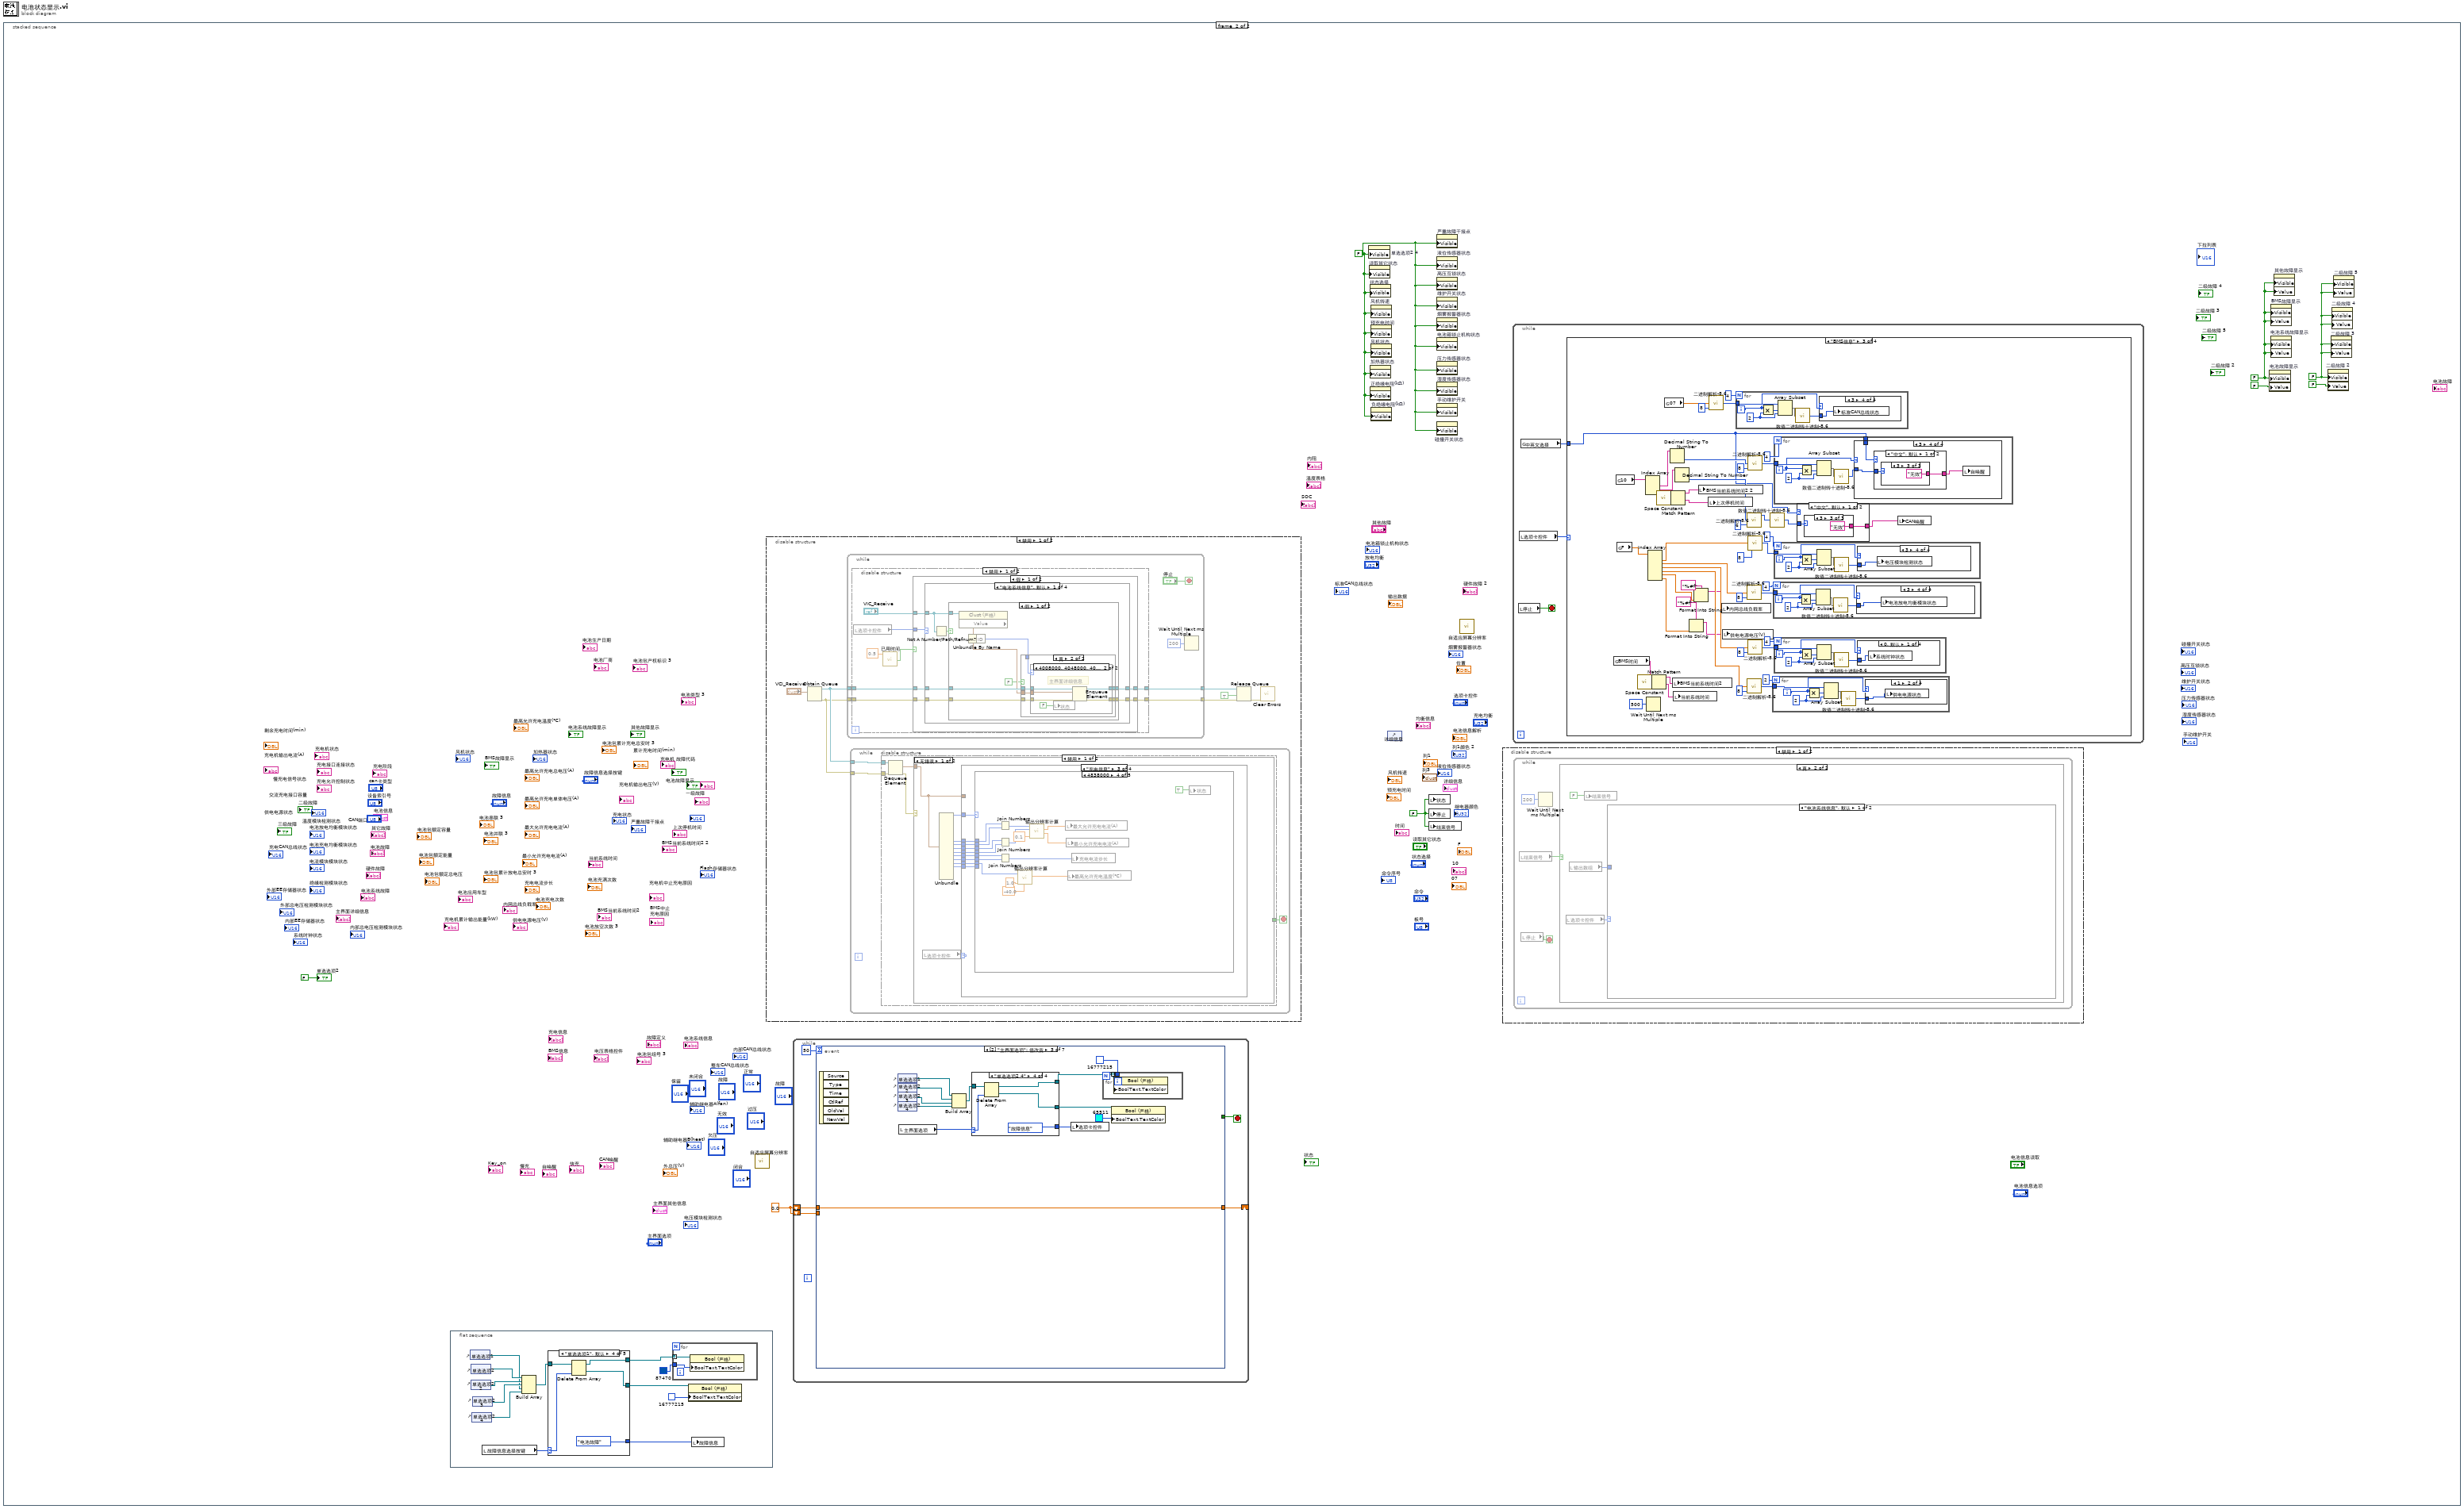
[diagram p0: block diagram]
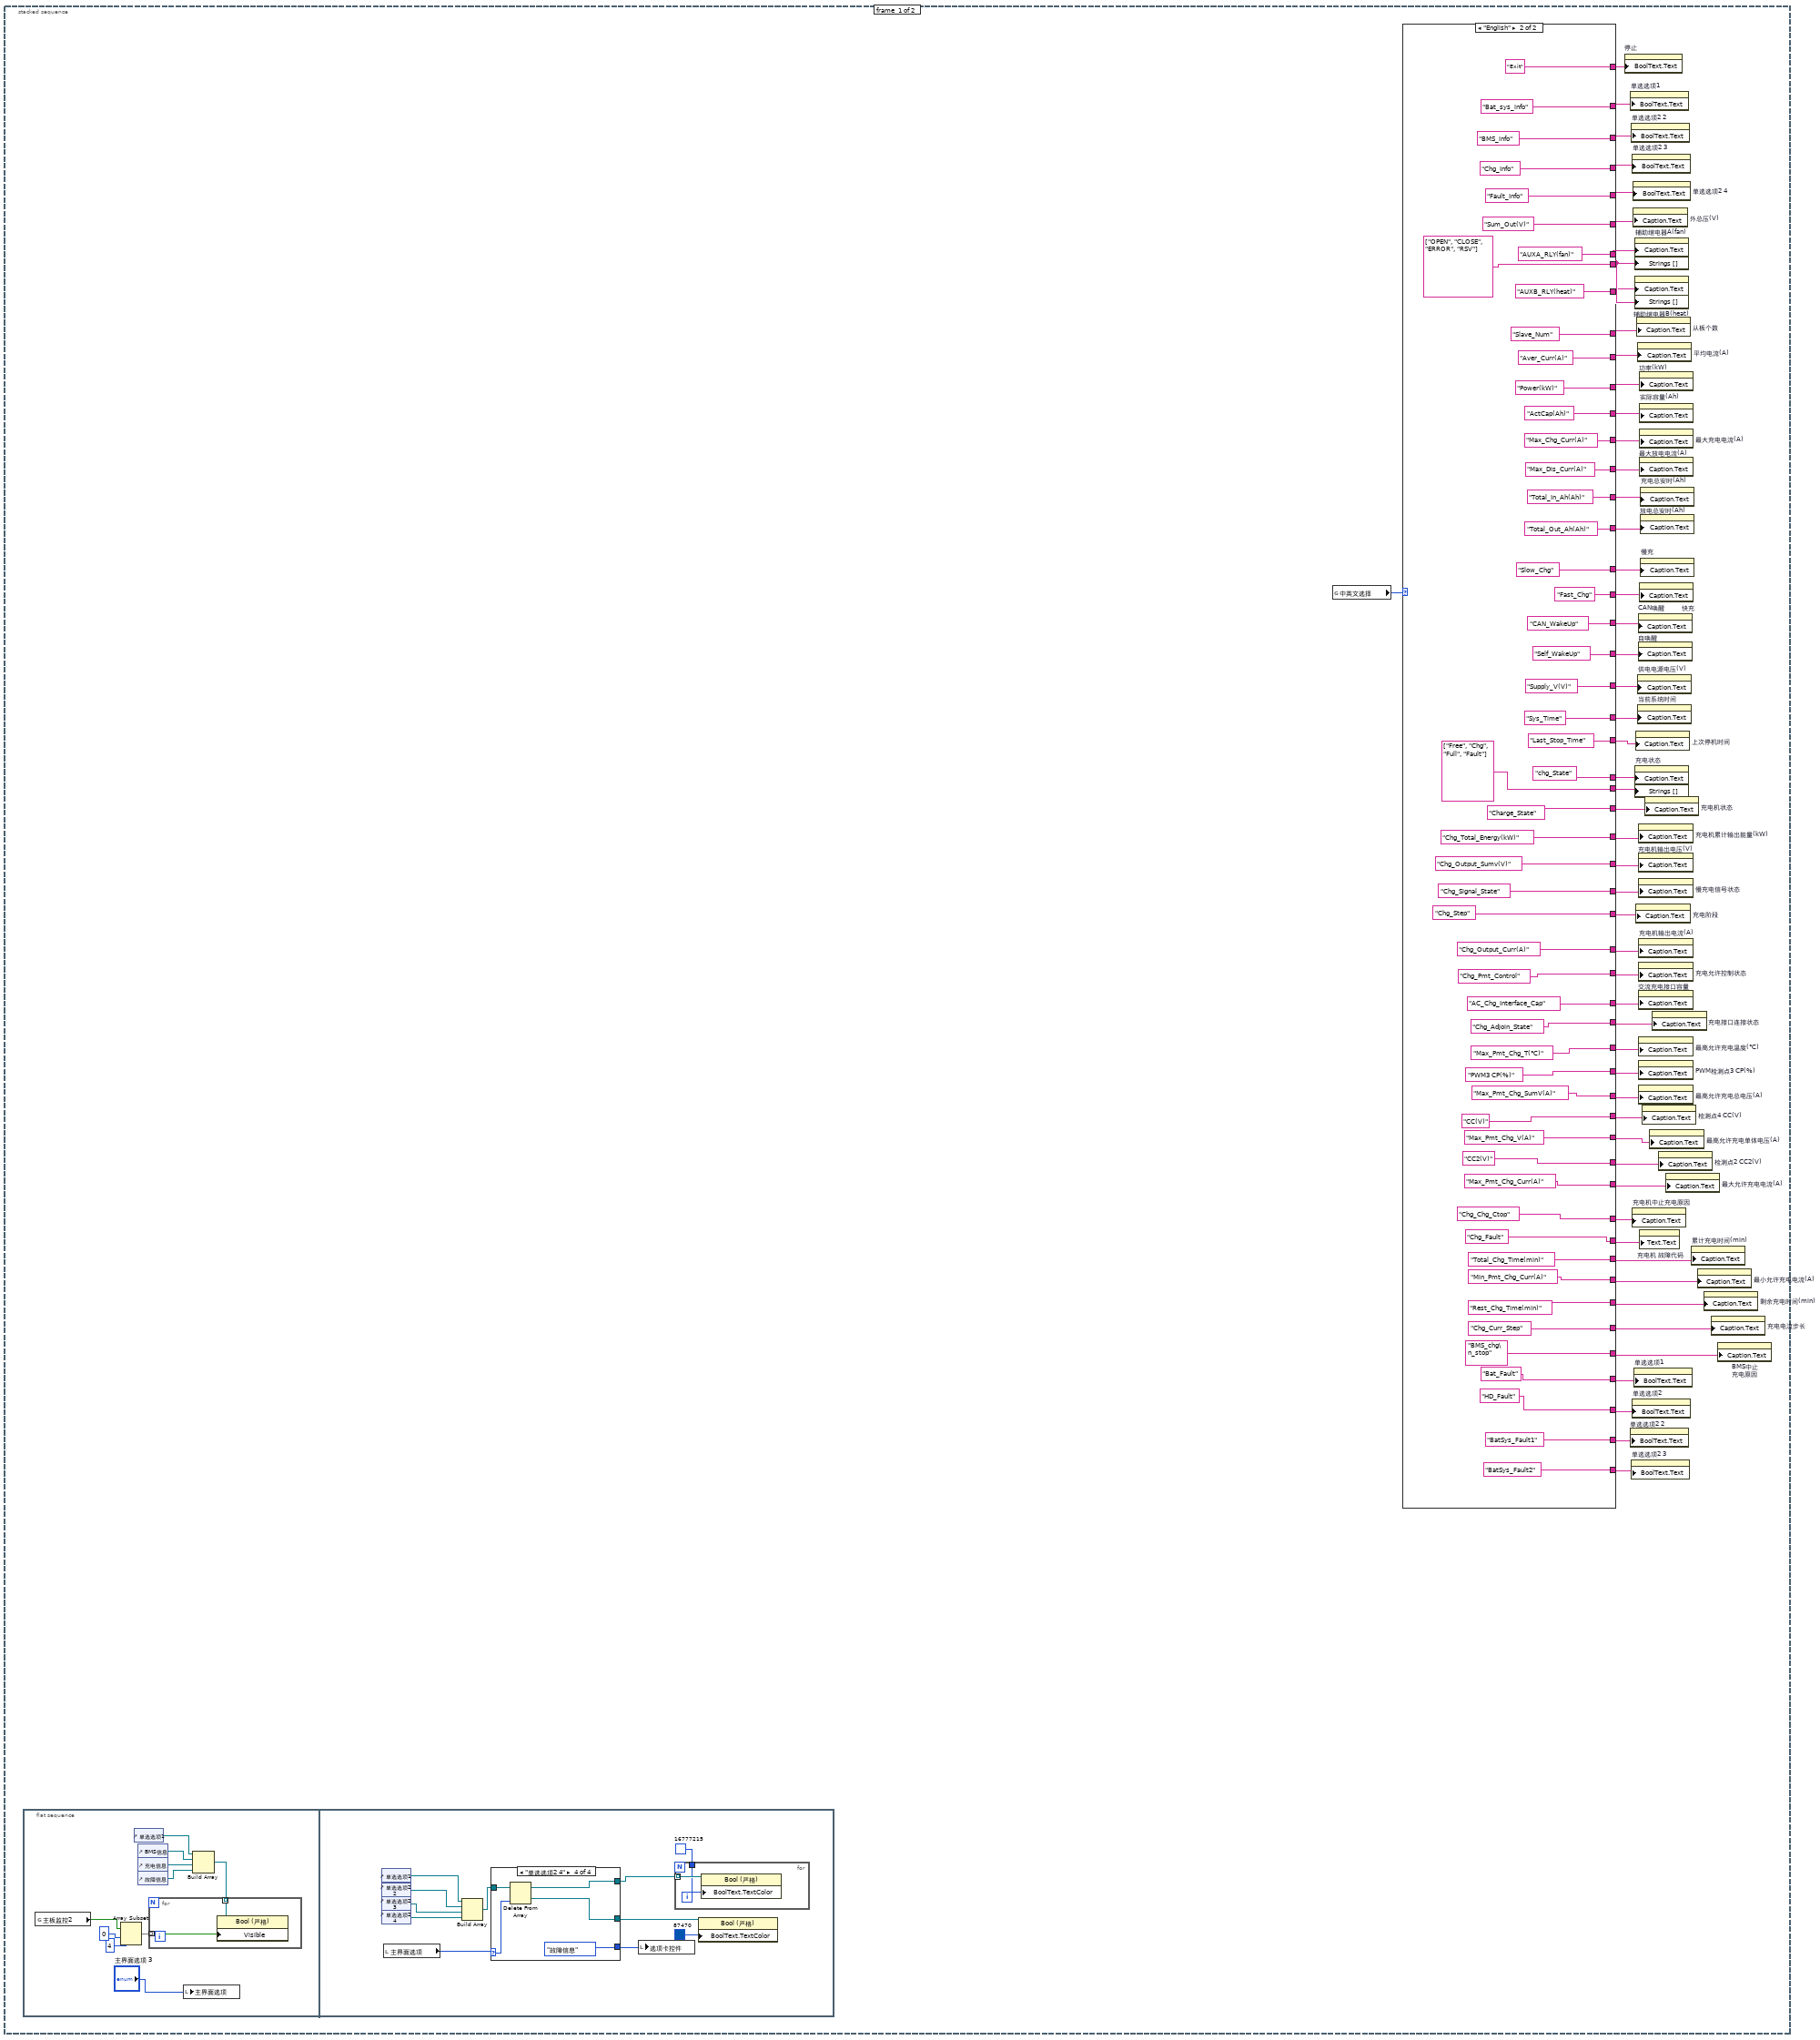
[diagram p2: hidden frame]
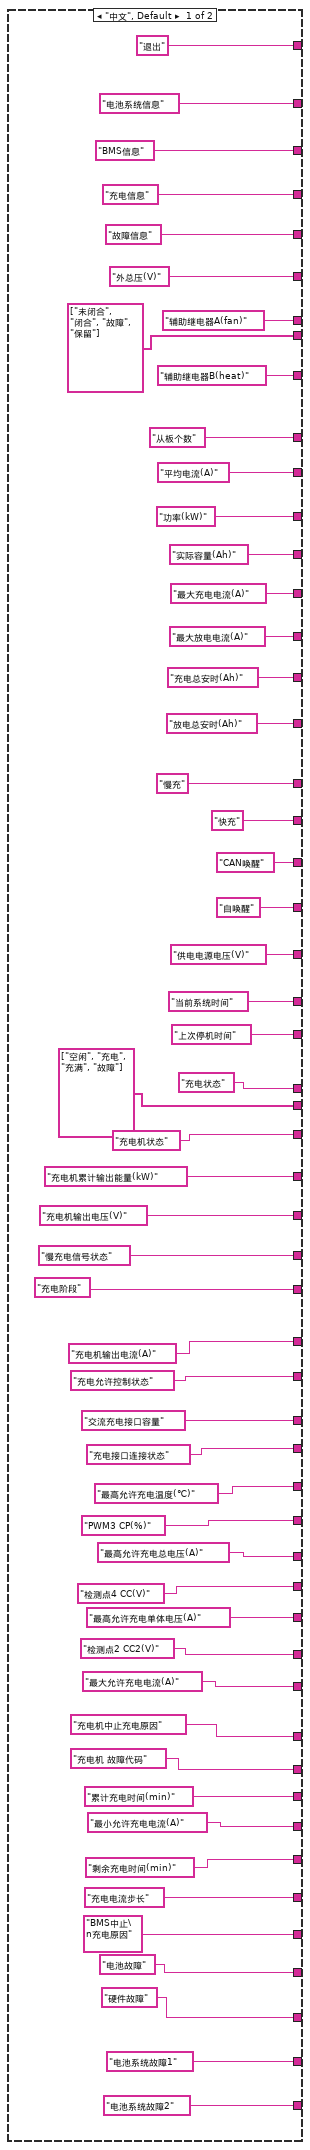
[diagram p3: hidden frame]
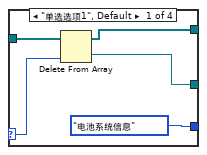
[diagram p4: hidden frame]
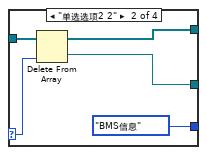
[diagram p5: hidden frame]
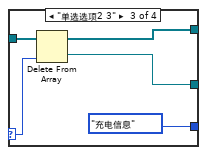
[diagram p6: hidden frame]
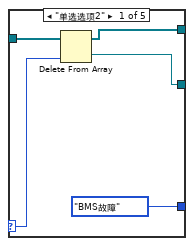
[diagram p7: hidden frame]
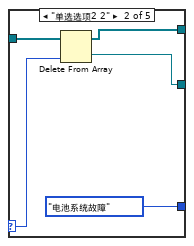
[diagram p8: hidden frame]
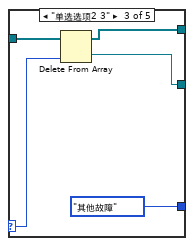
[diagram p9: hidden frame]
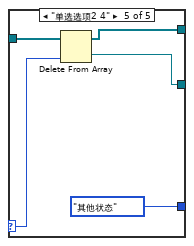
[diagram p10: hidden frame]
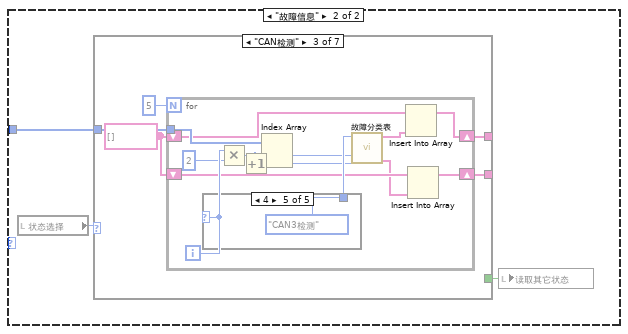
[diagram p12: hidden frame]
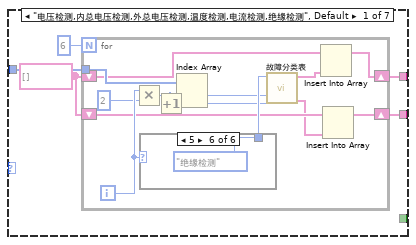
[diagram p13: hidden frame]
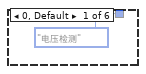
[diagram p14: hidden frame]
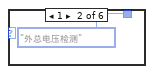
[diagram p15: hidden frame]
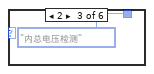
[diagram p16: hidden frame]
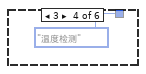
[diagram p17: hidden frame]
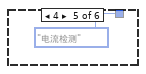
[diagram p18: hidden frame]
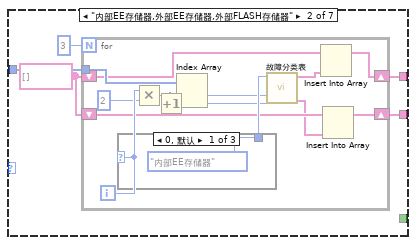
[diagram p19: hidden frame]
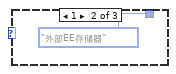
[diagram p20: hidden frame]
diagram:
  n1 = stacked-sequence {
    frame #0 {
      n2 = flat-sequence {
        frame #0 {
          n3 = global read "功能码全局.vi" "主板监控2"() -> (w170:bool[])
          n4 = Array Subset(array=w170, index=0 ("索引"), length=4 ("长度")) -> (w167:bool[])
          n5 = control-ref of="单选选项1"() -> (w162:refnum<vi>)
          n6 = control-ref of="BMS信息"() -> (w166:refnum<vi>)
          n7 = control-ref of="充电信息"() -> (w165:refnum<vi>)
          n8 = control-ref of="故障信息"() -> (w164:refnum<vi>)
          n9 = local write "主界面选项"("主界面选项 3") -> ()
          n10 = Build Array(w162, w166, w165, w164) -> (w163:refnum<vi>[])
          n11 = for {
            tunnel: w167 -> [w171] mode=indexing
            tunnel: w163 -> [w172] mode=indexing
            n12 = property class="Bool (严格)"(reference=w172, "Visible"=w171) -> ()  [unwired: 1 in, 2 out]
          }
        }
        frame #1 {
          n13 = control-ref of="单选选项1"() -> (w178:refnum<vi>)
          n14 = control-ref of="单选选项2 2"() -> (w180:refnum<vi>)
          n15 = control-ref of="单选选项2 3"() -> (w181:refnum<vi>)
          n16 = control-ref of="单选选项2 4"() -> (w182:refnum<vi>)
          n17 = local read "主界面选项"() -> (w175:enum32{"单选选项1", "单选选项2 2", "单选选项2 3", "单选选项2 4"})
          n18 = Build Array(w178, w180, w181, w182) -> (w179:refnum<vi>[])
          n19 = case shown="\"单选选项2 4\"" w175 {
            selector: w175 -> [w189 w195 w200 w205]
            tunnel: [w188 w194 w199 w204] -> w174
            tunnel: [w187 w193 w198 w203] -> w177
            tunnel: w179 -> [w190 w192 w197 w202]
            tunnel: [enum32{"电池系统信息", "BMS信息", "充电信息", "故障信息"}."电池系统信息" ("值") enum32{"电池系统信息", "BMS信息", "充电信息", "故障信息"}."BMS信息" ("值") enum32{"电池系统信息", "BMS信息", "充电信息", "故障信息"}."充电信息" ("值") enum32{"电池系统信息", "BMS信息", "充电信息", "故障信息"}."故障信息" ("值")] -> w183
            frame "单选选项1", Default {
              n20 = Delete From Array(array=w190, index=w189) -> (deleted portion=w187:refnum<vi>, array with subset deleted=w188:refnum<vi>[])  [unwired: 1 in]
            }
            frame "单选选项2 2" {
              n21 = Delete From Array(array=w192, index=w195) -> (deleted portion=w193:refnum<vi>, array with subset deleted=w194:refnum<vi>[])  [unwired: 1 in]
            }
            frame "单选选项2 3" {
              n22 = Delete From Array(array=w197, index=w200) -> (deleted portion=w198:refnum<vi>, array with subset deleted=w199:refnum<vi>[])  [unwired: 1 in]
            }
            frame "单选选项2 4" {
              n23 = Delete From Array(array=w202, index=w205) -> (deleted portion=w203:refnum<vi>, array with subset deleted=w204:refnum<vi>[])  [unwired: 1 in]
            }
          }
          n24 = local write "选项卡控件"(w183) -> ()
          n25 = for {
            tunnel: w174 -> [w185] mode=indexing
            tunnel: u32 16777215 -> [w184]
            n26 = property class="Bool (严格)"(reference=w185, "BoolText.TextColor"=w184) -> ()  [unwired: 1 in, 2 out]
          }
          n27 = property class="Bool (严格)"(reference=w177, "BoolText.TextColor"=u32 87470) -> ()  [unwired: 1 in, 2 out]
        }
      }
      n28 = global read "中英文全局.vi" "中英文选择"() -> (w54:enum32{"中文", "English"})
      n29 = case shown="\"English\"" w54 {
        tunnel: ["电池系统信息" "Bat_sys_info"] -> w53
        tunnel: ["BMS信息" "BMS_info"] -> w52
        tunnel: ["充电信息" "Chg_Info"] -> w51
        tunnel: ["故障信息" "Fault_Info"] -> w50
        tunnel: ["外总压(V)" "Sum_Out(V)"] -> w49
        tunnel: [string[] ["未闭合", "闭合", "故障", "保留"] ("字符串[]") string[] ["OPEN", "CLOSE", "ERROR", "RSV"] ("字符串[]")] -> w48
        tunnel: ["辅助继电器A(fan)" "AUXA_RLY(fan)"] -> w47
        tunnel: ["辅助继电器B(heat)" "AUXB_RLY(heat)"] -> w46
        tunnel: ["从板个数" "Slave_Num"] -> w45
        tunnel: ["平均电流(A)" "Aver_Curr(A)"] -> w44
        tunnel: ["功率(kW)" "Power(kW)"] -> w43
        tunnel: ["实际容量(Ah)" "ActCap(Ah)"] -> w42
        tunnel: ["最大充电电流(A)" "Max_Chg_Curr(A)"] -> w41
        tunnel: ["最大放电电流(A)" "Max_Dis_Curr(A)"] -> w40
        tunnel: ["充电总安时(Ah)" "Total_In_Ah(Ah)"] -> w39
        tunnel: ["放电总安时(Ah)" "Total_Out_Ah(Ah)"] -> w38
        tunnel: ["慢充" "Slow_Chg"] -> w37
        tunnel: ["快充" "Fast_Chg"] -> w36
        tunnel: ["CAN唤醒" "CAN_WakeUp"] -> w35
        tunnel: ["自唤醒" "Self_WakeUp"] -> w34
        tunnel: ["供电电源电压(V)" "Supply_V(V)"] -> w33
        tunnel: ["当前系统时间" "Sys_Time"] -> w32
        tunnel: ["上次停机时间" "Last_Stop_Time"] -> w31
        tunnel: ["退出" "Exit"] -> w30
        tunnel: [string[] ["空闲", "充电", "充满", "故障"] ("字符串[]") string[] ["Free", "Chg", "Full", "Fault"] ("字符串[]")] -> w29
        tunnel: ["充电状态" "chg_State"] -> w28
        tunnel: ["充电机累计输出能量(kW)" "Chg_Total_Energy(kW)"] -> w27
        tunnel: ["充电机输出电压(V)" "Chg_Output_Sumv(V)"] -> w26
        tunnel: ["慢充电信号状态" "Chg_Signal_State"] -> w25
        tunnel: ["充电阶段" "Chg_Step"] -> w24
        tunnel: ["充电机状态" "Charge_State"] -> w23
        tunnel: ["充电机输出电流(A)" "Chg_Output_Curr(A)"] -> w22
        tunnel: ["充电允许控制状态" "Chg_Pmt_Control"] -> w21
        tunnel: ["交流充电接口容量" "AC_Chg_Interface_Cap"] -> w20
        tunnel: ["充电接口连接状态" "Chg_Adjoin_State"] -> w19
        tunnel: ["最高允许充电温度(℃)" "Max_Pmt_Chg_T(℃)"] -> w18
        tunnel: ["PWM3 CP(%)" "PWM3 CP(%)"] -> w17
        tunnel: ["最高允许充电总电压(A)" "Max_Pmt_Chg_SumV(A)"] -> w16
        tunnel: ["检测点4 CC(V)" "CC(V)"] -> w15
        tunnel: ["最高允许充电单体电压(A)" "Max_Pmt_Chg_V(A)"] -> w14
        tunnel: ["检测点2 CC2(V)" "CC2(V)"] -> w13
        tunnel: ["最大允许充电电流(A)" "Max_Pmt_Chg_Curr(A)"] -> w12
        tunnel: ["累计充电时间(min)" "Total_Chg_Time(min)"] -> w11
        tunnel: ["最小允许充电电流(A)" "Min_Pmt_Chg_Curr(A)"] -> w10
        tunnel: ["剩余充电时间(min)" "Rest_Chg_Time(min)"] -> w9
        tunnel: ["充电电流步长" "Chg_Curr_Step"] -> w8
        tunnel: ["BMS中止\n充电原因" "BMS_chg\n_stop"] -> w7
        tunnel: ["电池故障" "Bat_Fault"] -> w6
        tunnel: ["硬件故障" "HD_Fault"] -> w5
        tunnel: ["电池系统故障1" "BatSys_Fault1"] -> w4
        tunnel: ["电池系统故障2" "BatSys_Fault2"] -> w3
        tunnel: ["充电机中止充电原因" "Chg_Chg_Ctop"] -> w2
        tunnel: ["充电机 故障代码" "Chg_Fault"] -> w1
        frame "中文", Default {
        }
        frame "English" {
        }
      }
      n30 = property on="停止" class="Bool (严格)"("BoolText.Text"=w30) -> ()  [unwired: 2 in, 2 out]
      n31 = property on="单选选项1" class="Bool (严格)"("BoolText.Text"=w53) -> ()  [unwired: 2 in, 2 out]
      n32 = property on="单选选项2 2" class="Bool (严格)"("BoolText.Text"=w4) -> ()  [unwired: 2 in, 2 out]
      n33 = property on="单选选项2 2" class="Bool (严格)"("BoolText.Text"=w52) -> ()  [unwired: 2 in, 2 out]
      n34 = property on="单选选项2 3" class="Bool (严格)"("BoolText.Text"=w3) -> ()  [unwired: 2 in, 2 out]
      n35 = property on="单选选项2 3" class="Bool (严格)"("BoolText.Text"=w51) -> ()  [unwired: 2 in, 2 out]
      n36 = property on="充电机中止充电原因" class="Str"("Caption.Text"=w2) -> ()  [unwired: 2 in, 2 out]
      n37 = property on="单选选项2" class="Bool (严格)"("BoolText.Text"=w5) -> ()  [unwired: 2 in, 2 out]
      n38 = property on="单选选项2 4" class="Bool (严格)"("BoolText.Text"=w50) -> ()  [unwired: 2 in, 2 out]
      n39 = property on="外总压(V)" class="Knob (严格)"("Caption.Text"=w49) -> ()  [unwired: 2 in, 2 out]
      n40 = property on="单选选项1" class="Bool (严格)"("BoolText.Text"=w6) -> ()  [unwired: 2 in, 2 out]
      n41 = property on="辅助继电器A(fan)" class="Ring (严格)"("Caption.Text"=w47, "Strings []"=w48) -> ()  [unwired: 2 in, 2 out]
      n42 = property on="辅助继电器B(heat)" class="Ring (严格)"("Caption.Text"=w46, "Strings []"=w48) -> ()  [unwired: 2 in, 2 out]
      n43 = property on="充电状态" class="Ring (严格)"("Caption.Text"=w28, "Strings []"=w29) -> ()  [unwired: 2 in, 2 out]
      n44 = property on="上次停机时间" class="Str"("Caption.Text"=w31) -> ()  [unwired: 2 in, 2 out]
      n45 = property on="充电阶段" class="Str"("Caption.Text"=w24) -> ()  [unwired: 2 in, 2 out]
      n46 = property on="从板个数" class="DigNum (严格)"("Caption.Text"=w45) -> ()  [unwired: 2 in, 2 out]
      n47 = property on="平均电流(A)" class="DigNum (严格)"("Caption.Text"=w44) -> ()  [unwired: 2 in, 2 out]
      n48 = property on="供电电源电压(V)" class="Str"("Caption.Text"=w33) -> ()  [unwired: 2 in, 2 out]
      n49 = property on="当前系统时间" class="Str"("Caption.Text"=w32) -> ()  [unwired: 2 in, 2 out]
      n50 = property on="CAN唤醒" class="Str"("Caption.Text"=w35) -> ()  [unwired: 2 in, 2 out]
      n51 = property on="自唤醒" class="Str"("Caption.Text"=w34) -> ()  [unwired: 2 in, 2 out]
      n52 = property on="充电机累计输出能量(kW)" class="Str"("Caption.Text"=w27) -> ()  [unwired: 2 in, 2 out]
      n53 = property on="充电机输出电压(V)" class="Str"("Caption.Text"=w26) -> ()  [unwired: 2 in, 2 out]
      n54 = property on="慢充电信号状态" class="Str"("Caption.Text"=w25) -> ()  [unwired: 2 in, 2 out]
      n55 = property on="充电机输出电流(A)" class="Str (严格)"("Caption.Text"=w22) -> ()  [unwired: 2 in, 2 out]
      n56 = property on="充电允许控制状态" class="Str"("Caption.Text"=w21) -> ()  [unwired: 2 in, 2 out]
      n57 = property on="交流充电接口容量" class="Str"("Caption.Text"=w20) -> ()  [unwired: 2 in, 2 out]
      n58 = property on="最高允许充电温度(℃)" class="DigNum (严格)"("Caption.Text"=w18) -> ()  [unwired: 2 in, 2 out]
      n59 = property on="PWM检测点3 CP(%)" class="DigNum (严格)"("Caption.Text"=w17) -> ()  [unwired: 2 in, 2 out]
      n60 = property on="最高允许充电总电压(A)" class="DigNum (严格)"("Caption.Text"=w16) -> ()  [unwired: 2 in, 2 out]
      n61 = property on="功率(kW)" class="DigNum (严格)"("Caption.Text"=w43) -> ()  [unwired: 2 in, 2 out]
      n62 = property on="实际容量(Ah)" class="DigNum (严格)"("Caption.Text"=w42) -> ()  [unwired: 2 in, 2 out]
      n63 = property on="最大充电电流(A)" class="DigNum (严格)"("Caption.Text"=w41) -> ()  [unwired: 2 in, 2 out]
      n64 = property on="最大放电电流(A)" class="DigNum (严格)"("Caption.Text"=w40) -> ()  [unwired: 2 in, 2 out]
      n65 = property on="快充" class="Str"("Caption.Text"=w36) -> ()  [unwired: 2 in, 2 out]
      n66 = property on="充电机 故障代码" class="Str"("Text.Text"=w1) -> ()  [unwired: 2 in, 2 out]
      n67 = property on="充电总安时(Ah)" class="DigNum (严格)"("Caption.Text"=w39) -> ()  [unwired: 2 in, 2 out]
      n68 = property on="放电总安时(Ah)" class="DigNum (严格)"("Caption.Text"=w38) -> ()  [unwired: 2 in, 2 out]
      n69 = property on="慢充" class="Str"("Caption.Text"=w37) -> ()  [unwired: 2 in, 2 out]
      n70 = property on="检测点4 CC(V)" class="DigNum (严格)"("Caption.Text"=w15) -> ()  [unwired: 2 in, 2 out]
      n71 = property on="充电机状态" class="Str"("Caption.Text"=w23) -> ()  [unwired: 2 in, 2 out]
      n72 = property on="最高允许充电单体电压(A)" class="DigNum (严格)"("Caption.Text"=w14) -> ()  [unwired: 2 in, 2 out]
      n73 = property on="充电接口连接状态" class="Str"("Caption.Text"=w19) -> ()  [unwired: 2 in, 2 out]
      n74 = property on="检测点2 CC2(V)" class="DigNum (严格)"("Caption.Text"=w13) -> ()  [unwired: 2 in, 2 out]
      n75 = property on="最大允许充电电流(A)" class="DigNum (严格)"("Caption.Text"=w12) -> ()  [unwired: 2 in, 2 out]
      n76 = property on="累计充电时间(min)" class="DigNum (严格)"("Caption.Text"=w11) -> ()  [unwired: 2 in, 2 out]
      n77 = property on="最小允许充电电流(A)" class="DigNum (严格)"("Caption.Text"=w10) -> ()  [unwired: 2 in, 2 out]
      n78 = property on="剩余充电时间(min)" class="DigNum (严格)"("Caption.Text"=w9) -> ()  [unwired: 2 in, 2 out]
      n79 = property on="充电电流步长" class="DigNum (严格)"("Caption.Text"=w8) -> ()  [unwired: 2 in, 2 out]
      n80 = property on="BMS中止\n充电原因" class="Str"("Caption.Text"=w7) -> ()  [unwired: 2 in, 2 out]
    }
    frame #1 {
      w206 = FALSE ("可见")
      w207 = 0.0 ("life")
      w210 = FALSE ("可见")
      w209 = FALSE ("可见")
      w213 = FALSE ("停止")
      n81 = flat-sequence {
        frame #0 {
          n82 = control-ref of="单选选项1"() -> (w214:refnum<vi>)
          n83 = control-ref of="单选选项2"() -> (w221:refnum<vi>)
          n84 = control-ref of="单选选项2 2"() -> (w220:refnum<vi>)
          n85 = control-ref of="单选选项2 4"() -> (w218:refnum<vi>)
          n86 = control-ref of="单选选项2 3"() -> (w219:refnum<vi>)
          n87 = local read "故障信息选择按键"() -> (w215:T7)
          n88 = Build Array(w221, w220, w219, w214, w218) -> (w217:refnum<vi>[])
          n89 = case shown="\"单选选项1\", 默认" w215 {
            selector: w215 -> [w231 w236 w241 w246 w251]
            tunnel: [w230 w235 w240 w245 w250] -> w225
            tunnel: [w229 w234 w239 w244 w249] -> w223
            tunnel: w217 -> [w232 w237 w242 w247 w252]
            tunnel: [T8."BMS故障" ("故障信息") T8."电池系统故障" ("故障信息") T8."其他故障" ("故障信息") T8."电池故障" ("故障信息") T8."其他状态" ("故障信息")] -> w222
            frame "单选选项2" {
              n90 = Delete From Array(array=w232, index=w231) -> (deleted portion=w229:refnum<vi>, array with subset deleted=w230:refnum<vi>[])  [unwired: 1 in]
            }
            frame "单选选项2 2" {
              n91 = Delete From Array(array=w237, index=w236) -> (deleted portion=w234:refnum<vi>, array with subset deleted=w235:refnum<vi>[])  [unwired: 1 in]
            }
            frame "单选选项2 3" {
              n92 = Delete From Array(array=w242, index=w241) -> (deleted portion=w239:refnum<vi>, array with subset deleted=w240:refnum<vi>[])  [unwired: 1 in]
            }
            frame "单选选项1", Default {
              n93 = Delete From Array(array=w247, index=w246) -> (deleted portion=w244:refnum<vi>, array with subset deleted=w245:refnum<vi>[])  [unwired: 1 in]
            }
            frame "单选选项2 4" {
              n94 = Delete From Array(array=w252, index=w251) -> (deleted portion=w249:refnum<vi>, array with subset deleted=w250:refnum<vi>[])  [unwired: 1 in]
            }
          }
          n95 = for {
            tunnel: u32 87470 -> [w227]
            tunnel: w225 -> [w226] mode=indexing
            n96 = property class="Bool (严格)"(reference=w226, "BoolText.TextColor"=w227) -> ()  [unwired: 1 in, 2 out]
          }
          n97 = property class="Bool (严格)"(reference=w223, "BoolText.TextColor"=u32 16777215) -> ()  [unwired: 1 in, 2 out]
          n98 = local write "故障信息"(w222) -> ()
        }
      }
      n99 = call "自适应屏幕分辨率.vi"() -> ()  [unwired: 16 in]
      n100 = disable-structure shown="禁用" {
        frame Disabled {
          n101 = Obtain Queue(element data type="VCI_Receive") -> (queue out=w1590:refnum<queue>, error out=w1589:errorcluster)  [unwired: 4 in, 1 out]
          n102 = while {
            tunnel: w1590 -> [w1951]
            tunnel: w1589 -> [w1950]
            tunnel: [w1949] -> w1588
            tunnel: [w1948] -> w1587
            stop <- "停止" stop-if-true
            n103 = disable-structure shown="禁用" {
              disable-tunnel: w1951 -> [w1958 _]
              disable-tunnel: w1950 -> [w1957 _]
              disable-tunnel: [w1956 _] -> w1949
              disable-tunnel: [w1955 _] -> w1948
              frame Disabled {
                n104 = local read "选项卡控件"() -> (w1959:enum32{"电池系统信息", "BMS信息", "充电信息", "故障信息"})
                n105 = call "已用时间"("Time Target (s)"=0.5) -> ("Time has Elapsed"=w1953:bool)  [unwired: 4 in, 14 out]
                n106 = case shown="假" w1953 {
                  tunnel: "VIC_Receive" -> [w1966 _]
                  tunnel: w1959 -> [w1965 _]
                  tunnel: w1958 -> [w1964 w2072]
                  tunnel: w1957 -> [w1963 w2071]
                  tunnel: [w1962 w2070] -> w1956
                  tunnel: [w1961 w2068] -> w1955
                  frame False {
                    n107 = case shown="\"电池系统信息\", 默认" w1965 {
                      tunnel: w1966 -> [w1968 w2000 w2023 w2046]
                      tunnel: w1964 -> [w1972 w2004 w2027 w2050]
                      tunnel: w1963 -> [w1971 w2003 w2026 w2049]
                      tunnel: [w1970 w2002 w2025 w2048] -> w1962
                      tunnel: [w1969 w2001 w2024 w2047] -> w1961
                      frame "电池系统信息", Default {
                        n108 = Not A Number/Path/Refnum?(number/path/refnum=w1968) -> (NaN/Path/Refnum?=w1967:bool)
                        n109 = case shown="假" w1967 {
                          tunnel: w1972 -> [w1980 w1998]
                          tunnel: w1971 -> [w1979 w1997]
                          tunnel: [w1977 w1998] -> w1970
                          tunnel: [w1976 w1997] -> w1969
                          tunnel: w1968 -> [w1975 _]
                          frame False {
                            n110 = property class="Clust (严格)"(reference=w1975) -> ("Value"=w1978:T4)  [unwired: 1 in, 2 out]
                            n111 = Unbundle By Name(w1978) -> ("ID"=w1974:u32)
                            n112 = case shown="真" FALSE {
                              tunnel: w1980 -> [w1982 w1988]
                              tunnel: w1979 -> [w1981 w1987]
                              tunnel: w1978 -> [_ w1986]
                              tunnel: [w1982 w1985] -> w1977
                              tunnel: [w1981 w1984] -> w1976
                              tunnel: w1974 -> [_ w1983]
                              frame False {
                              }
                              frame True {
                                n113 = case shown="4008000, 4048000, 4058000, 4068000, 4088000, 40E8000, 4FF3F00" w1983 {
                                tunnel: w1988 -> [w1990 w1996]
                                tunnel: w1987 -> [w1989 w1995]
                                tunnel: w1986 -> [_ w1994]
                                tunnel: [w1990 w1993] -> w1985
                                tunnel: [w1989 w1992] -> w1984
                                frame 153, Default {
                                }
                                frame 67141632, 67403776, 67469312, 67534848, 67665920, 68059136, 83836672 {
                                # "主界面详细信息"
                                n114 = local write "状态"(FALSE ("状态")) -> ()
                                n115 = Enqueue Element(queue=w1996, element=w1994, error in (no error)=w1995) -> (queue out=w1993:refnum<queue>, error out=w1992:errorcluster)  [unwired: 2 out]
                                }
                                }
                              }
                            }
                          }
                          frame True {
                          }
                        }
                      }
                      frame "BMS信息" {
                        n116 = Not A Number/Path/Refnum?(number/path/refnum=w2000) -> (NaN/Path/Refnum?=w1999:bool)
                        n117 = case shown="假" w1999 {
                          tunnel: w2004 -> [w2011 w2021]
                          tunnel: w2003 -> [w2010 w2020]
                          tunnel: [w2008 w2021] -> w2002
                          tunnel: [w2007 w2020] -> w2001
                          tunnel: w2000 -> [w2006 _]
                          frame False {
                            n118 = property class="Clust (严格)"(reference=w2006) -> ("Value"=w2009:T4)  [unwired: 1 in, 2 out]
                            n119 = Unbundle By Name(w2009) -> ("ID"=w2005:u32)
                            n120 = case shown="4078000, 40F8000, 4108000, 18898000, 188A8000" w2005 {
                              tunnel: w2011 -> [w2013 w2019]
                              tunnel: w2010 -> [w2012 w2018]
                              tunnel: w2009 -> [_ w2017]
                              tunnel: [w2013 w2016] -> w2008
                              tunnel: [w2012 w2015] -> w2007
                              frame 0, Default {
                              }
                              frame 67600384, 68124672, 68190208, 411664384, 411729920 {
                                # "BMS信息"
                                n121 = Enqueue Element(queue=w2019, element=w2017, error in (no error)=w2018) -> (queue out=w2016:refnum<queue>, error out=w2015:errorcluster)  [unwired: 2 out]
                                n122 = local write "状态"(FALSE ("状态")) -> ()
                              }
                            }
                          }
                          frame True {
                          }
                        }
                      }
                      frame "充电信息" {
                        n123 = Not A Number/Path/Refnum?(number/path/refnum=w2023) -> (NaN/Path/Refnum?=w2022:bool)
                        n124 = case shown="假" w2022 {
                          tunnel: w2027 -> [w2034 w2044]
                          tunnel: w2026 -> [w2033 w2043]
                          tunnel: [w2031 w2044] -> w2025
                          tunnel: [w2030 w2043] -> w2024
                          tunnel: w2023 -> [w2029 _]
                          frame False {
                            n125 = property class="Clust (严格)"(reference=w2029) -> ("Value"=w2032:T4)  [unwired: 1 in, 2 out]
                            n126 = Unbundle By Name(w2032) -> ("ID"=w2028:u32)
                            n127 = case shown="4818000, 4828000, 4838000, 4848000" w2028 {
                              tunnel: w2034 -> [w2036 w2042]
                              tunnel: w2033 -> [w2035 w2041]
                              tunnel: w2032 -> [_ w2040]
                              tunnel: [w2036 w2039] -> w2031
                              tunnel: [w2035 w2038] -> w2030
                              frame 0, Default {
                              }
                              frame 75595776, 75661312, 75726848, 75792384 {
                                # "充电信息"
                                n128 = Enqueue Element(queue=w2042, element=w2040, error in (no error)=w2041) -> (queue out=w2039:refnum<queue>, error out=w2038:errorcluster)  [unwired: 2 out]
                                n129 = local write "状态"(FALSE ("状态")) -> ()
                              }
                            }
                          }
                          frame True {
                          }
                        }
                      }
                      frame "故障信息" {
                        n130 = Not A Number/Path/Refnum?(number/path/refnum=w2046) -> (NaN/Path/Refnum?=w2045:bool)
                        n131 = case shown="假" w2045 {
                          tunnel: w2050 -> [w2057 w2067]
                          tunnel: w2049 -> [w2056 w2066]
                          tunnel: [w2054 w2067] -> w2048
                          tunnel: [w2053 w2066] -> w2047
                          tunnel: w2046 -> [w2052 _]
                          frame False {
                            n132 = property class="Clust (严格)"(reference=w2052) -> ("Value"=w2055:T4)  [unwired: 1 in, 2 out]
                            n133 = Unbundle By Name(w2055) -> ("ID"=w2051:u32)
                            n134 = case shown="4098000, 40A8000, 40B8000, 40C8000, 18858000" w2051 {
                              tunnel: w2057 -> [w2059 w2065]
                              tunnel: w2056 -> [w2058 w2064]
                              tunnel: w2055 -> [_ w2063]
                              tunnel: [w2059 w2062] -> w2054
                              tunnel: [w2058 w2061] -> w2053
                              frame 0, Default {
                              }
                              frame 67731456, 67796992, 67862528, 67928064, 411402240 {
                                # "故障信息"
                                n135 = Enqueue Element(queue=w2065, element=w2063, error in (no error)=w2064) -> (queue out=w2062:refnum<queue>, error out=w2061:errorcluster)  [unwired: 2 out]
                                n136 = local write "状态"(FALSE ("状态")) -> ()
                              }
                            }
                          }
                          frame True {
                          }
                        }
                      }
                    }
                  }
                  frame True {
                    n137 = Flush Queue(queue=w2072, error in (no error)=w2071) -> (queue out=w2070:refnum<queue>, error out=w2069:errorcluster)  [unwired: 1 out]
                    n138 = call <vilib>:"Clear Errors.vi"("error in (no error)"=w2069) -> ("error out"=w2068:errorcluster)  [unwired: 6 out]
                  }
                }
              }
              frame Enabled {
              }
            }
            n139 = Wait Until Next ms Multiple(millisecond multiple=u32 200 ("毫秒倍数")) -> ()  [unwired: 1 out]
          }
          n140 = while {
            tunnel: w1590 -> [w1594]
            tunnel: w1589 -> [w1593]
            stop <- w1592 stop-if-true
            n141 = disable-structure shown="禁用" {
              disable-tunnel: [w1598 _] -> _
              disable-tunnel: w1594 -> [w1597 _]
              disable-tunnel: w1593 -> [w1596 _]
              disable-tunnel: [_ TRUE] -> w1592
              frame Disabled {
                n142 = Dequeue Element(queue=w1597, error in (no error)=w1596) -> (element=w1595:T4, error out=w1598:errorcluster)  [unwired: 3 out]
                n143 = case shown="无错误" w1598 {
                  tunnel: w1595 -> [w1608 _]
                  frame No Error {
                    n144 = local read "选项卡控件"() -> (w1609:enum32{"电池系统信息", "BMS信息", "充电信息", "故障信息"})
                    n145 = Unbundle(w1608) -> ("ID"=w1607:u32, "Data1"=w1606:u8, "Data2"=w1605:u8, "Data3"=w1604:u8, "Data4"=w1603:u8, "Data5"=w1602:u8, "Data6"=w1601:u8, "Data7"=w1600:u8, "Data8"=w1599:u8)  [unwired: 9 out]
                    n146 = case shown="\"充电信息\"" w1609 {
                      tunnel: w1608 -> [_ w1728 _ w1856]
                      tunnel: w1607 -> [w1618 w1727 w1787 w1846]
                      tunnel: w1606 -> [w1613 w1726 w1786 w1854]
                      tunnel: w1605 -> [w1612 w1725 w1785 w1853]
                      tunnel: w1604 -> [w1611 w1724 w1784 w1852]
                      tunnel: w1603 -> [w1610 w1723 w1783 w1851]
                      tunnel: w1602 -> [w1617 w1722 w1782 w1850]
                      tunnel: w1601 -> [w1616 w1721 w1781 w1849]
                      tunnel: w1600 -> [w1615 w1720 w1780 w1848]
                      tunnel: w1599 -> [w1614 w1719 w1779 w1847]
                      frame "电池系统信息", Default {
                        n147 = case shown="4068000" w1618 {
                          tunnel: w1617 -> [_ w1625 w1636 w1652 _ w1695 w1711 _]
                          tunnel: w1616 -> [_ w1624 w1635 w1651 w1674 w1694 w1710 _]
                          tunnel: w1615 -> [_ w1623 _ w1650 w1673 _ w1709 w1718]
                          tunnel: w1614 -> [_ w1622 _ w1649 _ _ w1708 _]
                          tunnel: w1613 -> [_ _ w1640 w1656 _ w1699 w1714 _]
                          tunnel: w1612 -> [_ _ w1639 w1655 w1676 w1698 w1713 _]
                          tunnel: w1611 -> [_ _ w1638 w1654 _ w1697 w1712 _]
                          tunnel: w1610 -> [_ _ w1637 w1653 w1675 w1696 _ _]
                          frame 0, Default {
                          }
                          frame 67141632 {
                            n148 = Join Numbers(hi=w1623, lo=w1622) -> ((hi.lo)=w1626:u16)
                            n149 = Join Numbers(hi=w1625, lo=w1624) -> ((hi.lo)=w1629:u16)
                            n150 = call "输出分辨率计算.vi"("偏移量"=sgl -3000.0, "分辨率"=0.1, "数值 2"=w1626) -> ("输出2"=→"平均电流":dbl)  [unwired: 3 in, 5 out]
                            n151 = call "输出分辨率计算.vi"("分辨率"=0.1, "数值 2"=w1629) -> ("输出2"=w1620:dbl)  [unwired: 4 in, 5 out]
                            n152 = local write "外总压(V)"(w1620) -> ()
                            n153 = local write "状态"(TRUE ("状态")) -> ()
                          }
                          frame 67403776 {
                            n154 = Join Numbers(hi=w1640, lo=w1639) -> ((hi.lo)=w1641:u16)
                            n155 = Join Numbers(hi=w1638, lo=w1637) -> ((hi.lo)=w1642:u16)
                            n156 = Join Numbers(hi=w1636, lo=w1635) -> ((hi.lo)=w1643:u16)
                            n157 = call "输出分辨率计算.vi"("分辨率"=0.1, "数值 2"=w1643) -> ("输出2"=→"实际容量":dbl)  [unwired: 4 in, 5 out]
                            n158 = call "输出分辨率计算.vi"("分辨率"=0.1, "数值 3"=w1642, "数值 2"=w1641) -> ("输出3"=→"最大放电电流":dbl, "输出2"=→"最大充电电流":dbl)  [unwired: 3 in, 4 out]
                            n159 = local write "状态"(TRUE ("状态")) -> ()
                          }
                          frame 67469312 {
                            n160 = Join Numbers(hi=w1652, lo=w1651) -> ((hi.lo)=w1661:u16)
                            n161 = Join Numbers(hi=w1650, lo=w1649) -> ((hi.lo)=w1662:u16)
                            n162 = Join Numbers(hi=w1656, lo=w1655) -> ((hi.lo)=w1659:u16)
                            n163 = Join Numbers(hi=w1654, lo=w1653) -> ((hi.lo)=w1658:u16)
                            n164 = Join Numbers(hi=w1661, lo=w1662) -> ((hi.lo)=w1663:u32)
                            n165 = Join Numbers(hi=w1659, lo=w1658) -> ((hi.lo)=w1660:u32)
                            n166 = To Double Precision Float(number=w1660) -> (double precision float=w1664:dbl)
                            n167 = To Double Precision Float(number=w1663) -> (double precision float=w1665:dbl)
                            n168 = call "输出分辨率计算.vi"("分辨率"=0.001, "数值 3"=w1665, "数值 2"=w1664) -> ("输出3"=→"放电总安时":dbl, "输出2"=→"充电总安时":dbl)  [unwired: 3 in, 4 out]
                            n169 = local write "状态"(TRUE ("状态")) -> ()
                          }
                          frame 67534848 {
                            n170 = call "二进制解析-8.6.vi"("索引"=4, "数值"=w1676) -> ("高位子数组"=w1689:i32[])  [unwired: 3 out]
                            n171 = Delete From Array(array=w1689, length=2 ("长度"), index=0 ("索引")) -> (deleted portion=w1687:i32[], array with subset deleted=w1688:i32[])
                            n172 = call "输出分辨率计算.vi"("分辨率"=0.2, "数值 3"=w1673, "数值 2"=w1674) -> ("输出3"=→"AI2":dbl, "输出2"=→"AI1":dbl)  [unwired: 3 in, 4 out]
                            n173 = call "数值二进制转十进制-8.6.vi"("子数组"=w1688) -> ("十进制数值"=w1668:i32)  [unwired: 4 out]
                            n174 = call "数值二进制转十进制-8.6.vi"("子数组"=w1687) -> ("十进制数值"=w1667:i32)  [unwired: 4 out]
                            n175 = local write "辅助继电器A(fan)"(w1668) -> ()
                            n176 = local write "辅助继电器B(heat)"(w1667) -> ()
                            n177 = call "各种状态子VI.vi"("颜色输入"=u32[] [16448250, 6618880, 16711680, 16860], "状态输入"=string[][] [["未闭合", "闭合", "故障", "保留"], ["未闭合", "闭合", "故障", "保留"], ["输出为低", "输出为高", "保留", "保留"], ["输出为低", "输出为高", "保留", "保留"]], "几种类型"=4, "数值"=w1676) -> ("状态"=→"DO":string[])  [unwired: 1 out]
                            n178 = call "各种状态子VI.vi"("颜色输入"=u32[] [16773465, 6618880, 16860, 16860], "状态输入"=string[][] [["输入为低", "输入为高", "保留", "保留"], ["输入为低", "输入为高", "保留", "保留"], ["输入为低", "输入为高", "保留", "保留"], ["输入为低", "输入为高", "保留", "保留"]], "几种类型"=4, "数值"=w1675) -> ("状态"=→"DI":string[])  [unwired: 1 out]
                            n179 = local write "状态"(TRUE ("状态")) -> ()
                          }
                          frame 67665920 {
                            n180 = Join Numbers(hi=w1699, lo=w1698) -> ((hi.lo)=w1701:u16)
                            n181 = Join Numbers(hi=w1697, lo=w1696) -> ((hi.lo)=w1702:u16)
                            n182 = Join Numbers(hi=w1695, lo=w1694) -> ((hi.lo)=w1703:u16)
                            n183 = call "输出分辨率计算.vi"("偏移量"=sgl -3000.0, "分辨率"=0.1, "数值 2"=w1703) -> ("输出2"=→"功率":dbl)  [unwired: 3 in, 5 out]
                            n184 = call "输出分辨率计算.vi"("分辨率"=0.5, "数值 3"=w1702, "数值 2"=w1701) -> ("输出3"=→"负绝缘":dbl, "输出2"=→"正绝缘":dbl)  [unwired: 3 in, 4 out]
                            n185 = local write "状态"(TRUE ("状态")) -> ()
                          }
                          frame 68059136 {
                            n186 = Join Numbers(hi=w1711, lo=w1710) -> ((hi.lo)=w1716:u16)
                            n187 = Join Numbers(hi=w1709, lo=w1708) -> ((hi.lo)=w1715:u16)
                            n188 = Build Array(w1714, w1713, w1712, w1716, w1715) -> (w1707:u16[])
                            n189 = local write "电池信息解析"(w1707) -> ()
                            n190 = local write "状态"(TRUE ("状态")) -> ()
                          }
                          frame 83836672 {
                            n191 = local write "状态"(TRUE ("状态")) -> ()
                            "从板个数" <- w1718
                          }
                        }
                      }
                      frame "BMS信息" {
                        n192 = disable-structure shown="禁用" {
                          disable-tunnel: w1728 -> [w1729 _]
                          frame Disabled {
                            n193 = local read "设备索引号"() -> (w1738:u8)
                            n194 = local read "can卡类型"() -> (w1739:u8)
                            n195 = local read "CAN端口"() -> (w1737:u8)
                            n196 = local read "命令"() -> (w1732:u32)
                            n197 = call "标定授权读取.vi"("VCI_Receive"=w1729) -> ()  [unwired: 1 out]
                            n198 = call "多帧接收机制(EV05).vi"("can卡类型"=w1739, "设备索引号"=w1738, "CAN端口"=w1737, "VCI_Receive"=w1729, "命令"=w1732, "板号"=u32 0, "写?"=FALSE) -> ("错误代码"=w1735:i32, "命令序号"=w1730:u8, "输出数组"=w1734:u8[], "结束信号"=w1733:bool)  [unwired: 1 in, 8 out]
                            n199 = local write "错误代码"(w1735) -> ()
                            n200 = local write "输出数组"(w1734) -> ()
                            n201 = local write "结束信号"(w1733) -> ()
                            n202 = local write "命令序号"(w1730) -> ()
                          }
                          frame Enabled {
                          }
                        }
                        n203 = case shown="40F8000" w1727 {
                          tunnel: w1726 -> [_ w1754 w1765 w1778]
                          tunnel: w1725 -> [_ w1753 w1764 _]
                          tunnel: w1724 -> [_ w1752 w1763 w1777]
                          tunnel: w1723 -> [_ w1751 w1762 w1776]
                          tunnel: w1722 -> [_ w1750 w1761 w1775]
                          tunnel: w1721 -> [_ w1749 w1760 w1774]
                          tunnel: w1720 -> [_ w1748 w1759 w1773]
                          tunnel: w1719 -> [_ w1747 w1758 w1772]
                          frame 0, Default {
                          }
                          frame 68124672 {
                            n204 = Join Numbers(hi=w1750, lo=w1749) -> ((hi.lo)=w1745:u16)
                            n205 = Join Numbers(hi=w1748, lo=w1747) -> ((hi.lo)=w1742:u16)
                            n206 = call "输出分辨率计算.vi"("分辨率"=0.2, "数值 2"=w1742) -> ("输出2"=w1741:dbl)  [unwired: 4 in, 5 out]
                            n207 = call "输出分辨率计算.vi"("分辨率"=0.1, "数值 2"=w1745) -> ("输出2"=w1744:dbl)  [unwired: 4 in, 5 out]
                            n208 = Build Array(w1754, w1753, w1752, w1751, w1744, w1741) -> (w1746:dbl[])
                            n209 = local write "F"(w1746) -> ()
                            n210 = local write "状态"(TRUE ("状态")) -> ()
                          }
                          frame 68190208 {
                            w1767 = "%#f" ("格式字符串")
                            n211 = call "时间合并-8.6.vi"("年"=w1763, "月"=w1762, "日"=w1761, "时"=w1760, "分"=w1759, "秒"=w1758) -> ("时间"=w1766:string)  [unwired: 13 out]
                            n212 = Format Into String(format string=w1767, w1765) -> (resulting string=w1768:string)  [unwired: 2 in, 1 out]
                            n213 = Format Into String(format string=w1767, w1764) -> (resulting string=w1769:string)  [unwired: 2 in, 1 out]
                            n214 = Build Array(w1768, w1769, w1766) -> (w1757:string[])
                            n215 = local write "10"(w1757) -> ()
                            n216 = local write "状态"(TRUE ("状态")) -> ()
                          }
                          frame 67600384 {
                            n217 = local write "07"(w1778) -> ()
                            n218 = call "时间合并-8.6.vi"("年"=w1777, "月"=w1776, "日"=w1775, "时"=w1774, "分"=w1773, "秒"=w1772) -> ("时间"=w1771:string)  [unwired: 13 out]
                            n219 = local write "时间"(w1771) -> ()
                            n220 = local write "状态"(TRUE ("状态")) -> ()
                          }
                        }
                      }
                      frame "充电信息" {
                        n221 = case shown="4838000" w1787 {
                          tunnel: w1786 -> [_ w1797 w1810 w1829 w1845]
                          tunnel: w1785 -> [_ w1796 w1809 w1828 w1844]
                          tunnel: w1784 -> [_ w1795 w1808 w1827 w1843]
                          tunnel: w1783 -> [_ w1794 w1807 w1826 w1842]
                          tunnel: w1782 -> [_ w1793 w1806 w1825 w1841]
                          tunnel: w1781 -> [_ w1792 w1805 w1824 w1840]
                          tunnel: w1780 -> [_ w1791 w1804 w1821 _]
                          tunnel: w1779 -> [_ w1790 w1803 _ _]
                          frame 0, Default {
                          }
                          frame 75595776 {
                            n222 = Build Array(w1797, w1796, w1795, w1794, w1793, w1792, w1791, w1790) -> (w1789:u8[])
                            n223 = local write "列1"(w1789) -> ()
                            n224 = local write "状态"(TRUE ("状态")) -> ()
                          }
                          frame 75661312 {
                            n225 = Join Numbers(hi=w1806, lo=w1805) -> ((hi.lo)=w1811:u16)
                            n226 = Join Numbers(hi=w1804, lo=w1803) -> ((hi.lo)=w1814:u16)
                            n227 = Join Numbers(hi=w1808, lo=w1807) -> ((hi.lo)=w1800:u16)
                            n228 = Join Numbers(hi=w1810, lo=w1809) -> ((hi.lo)=w1799:u16)
                            n229 = call "输出分辨率计算.vi"("分辨率"=0.1, "数值 2"=w1811) -> ("输出2"=w1802:dbl)  [unwired: 4 in, 5 out]
                            n230 = call "输出分辨率计算.vi"("分辨率"=0.001, "数值 2"=w1814) -> ("输出2"=w1801:dbl)  [unwired: 4 in, 5 out]
                            n231 = local write "最高允许充电单体电压(A)"(w1801) -> ()
                            n232 = local write "最高允许充电总电压(A)"(w1802) -> ()
                            n233 = local write "累计充电时间(min)"(w1799) -> ()
                            n234 = local write "剩余充电时间(min)"(w1800) -> ()
                            n235 = local write "状态"(TRUE ("状态")) -> ()
                          }
                          frame 75726848 {
                            n236 = Join Numbers(hi=w1829, lo=w1828) -> ((hi.lo)=w1820:u16)
                            n237 = Join Numbers(hi=w1827, lo=w1826) -> ((hi.lo)=w1819:u16)
                            n238 = Join Numbers(hi=w1825, lo=w1824) -> ((hi.lo)=w1822:u16)
                            n239 = call "输出分辨率计算.vi"("偏移量"=sgl -40.0, "分辨率"=1.0, "数值 2"=w1821) -> ("输出2"=w1823:dbl)  [unwired: 3 in, 5 out]
                            n240 = call "输出分辨率计算.vi"("分辨率"=0.1, "数值 3"=w1819, "数值 2"=w1820) -> ("输出3"=w1816:dbl, "输出2"=w1817:dbl)  [unwired: 3 in, 4 out]
                            n241 = local write "最大允许充电电流(A)"(w1817) -> ()
                            n242 = local write "最小允许充电电流(A)"(w1816) -> ()
                            n243 = local write "最高允许充电温度(℃)"(w1823) -> ()
                            n244 = local write "充电电流步长"(w1822) -> ()
                            n245 = local write "状态"(TRUE ("状态")) -> ()
                          }
                          frame 75792384 {
                            n246 = Join Numbers(hi=w1845, lo=w1844) -> ((hi.lo)=w1838:u16)
                            n247 = Join Numbers(hi=w1843, lo=w1842) -> ((hi.lo)=w1837:u16)
                            n248 = Join Numbers(hi=w1841, lo=w1840) -> ((hi.lo)=w1836:u16)
                            n249 = call "输出分辨率计算.vi"("分辨率"=0.1, "数值 4"=w1836, "数值 3"=w1837, "数值 2"=w1838) -> ("输出4"=w1835:dbl, "输出3"=w1834:dbl, "输出2"=w1833:dbl)  [unwired: 2 in, 3 out]
                            n250 = local write "充电机累计输出能量(kW)"(w1835) -> ()
                            n251 = local write "充电机输出电压(V)"(w1833) -> ()
                            n252 = local write "充电机输出电流(A)"(w1834) -> ()
                            n253 = local write "状态"(TRUE ("状态")) -> ()
                          }
                        }
                      }
                      frame "故障信息" {
                        n254 = local read "设备索引号"() -> (w1863:u8)
                        n255 = local read "can卡类型"() -> (w1864:u8)
                        n256 = local read "CAN端口"() -> (w1862:u8)
                        n257 = case shown="4098000" w1846 {
                          tunnel: w1854 -> [_ w1885 w1905 w1925 w1945]
                          tunnel: w1853 -> [_ w1884 w1904 w1924 w1944]
                          tunnel: w1852 -> [_ w1883 w1903 w1923 w1943]
                          tunnel: w1851 -> [_ w1882 w1902 w1922 w1942]
                          tunnel: w1850 -> [_ w1881 w1901 w1921 w1941]
                          tunnel: w1849 -> [_ w1880 w1900 w1920 w1940]
                          tunnel: w1848 -> [_ w1879 w1899 w1919 w1939]
                          tunnel: w1847 -> [_ w1878 w1898 w1918 w1938]
                          frame 0, Default {
                          }
                          frame 67731456 {
                            n258 = call "故障数值解析.vi"("输入"=w1885) -> ("结果"=w1868:string[])  [unwired: 2 out]
                            n259 = call "故障数值解析.vi"("输入"=w1884) -> ("结果"=w1869:string[])  [unwired: 2 out]
                            n260 = call "故障数值解析.vi"("输入"=w1883) -> ("结果"=w1870:string[])  [unwired: 2 out]
                            n261 = call "故障数值解析.vi"("输入"=w1882) -> ("结果"=w1874:string[])  [unwired: 2 out]
                            n262 = call "故障数值解析.vi"("输入"=w1881) -> ("结果"=w1871:string[])  [unwired: 2 out]
                            n263 = call "故障数值解析.vi"("输入"=w1880) -> ("结果"=w1872:string[])  [unwired: 2 out]
                            n264 = call "故障数值解析.vi"("输入"=w1879) -> ("结果"=w1873:string[])  [unwired: 2 out]
                            n265 = call "故障数值解析.vi"("输入"=w1878) -> ("结果"=w1875:string[])  [unwired: 2 out]
                            n266 = Build Array(w1868, w1869, w1870, w1874, w1871, w1872, w1873, w1875) -> (w1877:string[][])
                            n267 = Reshape Array(w1877, 32 ("维数大小")) -> (w1867:string[])
                            n268 = local write "电池故障"(w1867) -> ()
                            n269 = local write "状态"(TRUE ("状态")) -> ()
                          }
                          frame 67796992 {
                            n270 = call "故障数值解析.vi"("输入"=w1905) -> ("结果"=w1888:string[])  [unwired: 2 out]
                            n271 = call "故障数值解析.vi"("输入"=w1904) -> ("结果"=w1889:string[])  [unwired: 2 out]
                            n272 = call "故障数值解析.vi"("输入"=w1903) -> ("结果"=w1890:string[])  [unwired: 2 out]
                            n273 = call "故障数值解析.vi"("输入"=w1902) -> ("结果"=w1894:string[])  [unwired: 2 out]
                            n274 = call "故障数值解析.vi"("输入"=w1901) -> ("结果"=w1891:string[])  [unwired: 2 out]
                            n275 = call "故障数值解析.vi"("输入"=w1900) -> ("结果"=w1892:string[])  [unwired: 2 out]
                            n276 = call "故障数值解析.vi"("输入"=w1899) -> ("结果"=w1893:string[])  [unwired: 2 out]
                            n277 = call "故障数值解析.vi"("输入"=w1898) -> ("结果"=w1895:string[])  [unwired: 2 out]
                            n278 = Build Array(w1888, w1889, w1890, w1894, w1891, w1892, w1893, w1895) -> (w1897:string[][])
                            n279 = Reshape Array(w1897, 32 ("维数大小")) -> (w1887:string[])
                            n280 = local write "电池系统故障"(w1887) -> ()
                            n281 = local write "状态"(TRUE ("状态")) -> ()
                          }
                          frame 67862528 {
                            n282 = call "故障数值解析.vi"("输入"=w1925) -> ("结果"=w1908:string[])  [unwired: 2 out]
                            n283 = call "故障数值解析.vi"("输入"=w1924) -> ("结果"=w1909:string[])  [unwired: 2 out]
                            n284 = call "故障数值解析.vi"("输入"=w1923) -> ("结果"=w1910:string[])  [unwired: 2 out]
                            n285 = call "故障数值解析.vi"("输入"=w1922) -> ("结果"=w1914:string[])  [unwired: 2 out]
                            n286 = call "故障数值解析.vi"("输入"=w1921) -> ("结果"=w1911:string[])  [unwired: 2 out]
                            n287 = call "故障数值解析.vi"("输入"=w1920) -> ("结果"=w1912:string[])  [unwired: 2 out]
                            n288 = call "故障数值解析.vi"("输入"=w1919) -> ("结果"=w1913:string[])  [unwired: 2 out]
                            n289 = call "故障数值解析.vi"("输入"=w1918) -> ("结果"=w1915:string[])  [unwired: 2 out]
                            n290 = Build Array(w1908, w1909, w1910, w1914, w1911, w1912, w1913, w1915) -> (w1917:string[][])
                            n291 = Reshape Array(w1917, 32 ("维数大小")) -> (w1907:string[])
                            n292 = local write "其它故障"(w1907) -> ()
                            n293 = local write "状态"(TRUE ("状态")) -> ()
                          }
                          frame 67928064 {
                            n294 = call "故障数值解析.vi"("输入"=w1945) -> ("结果"=w1928:string[])  [unwired: 2 out]
                            n295 = call "故障数值解析.vi"("输入"=w1944) -> ("结果"=w1929:string[])  [unwired: 2 out]
                            n296 = call "故障数值解析.vi"("输入"=w1943) -> ("结果"=w1930:string[])  [unwired: 2 out]
                            n297 = call "故障数值解析.vi"("输入"=w1942) -> ("结果"=w1934:string[])  [unwired: 2 out]
                            n298 = call "故障数值解析.vi"("输入"=w1941) -> ("结果"=w1931:string[])  [unwired: 2 out]
                            n299 = call "故障数值解析.vi"("输入"=w1940) -> ("结果"=w1932:string[])  [unwired: 2 out]
                            n300 = call "故障数值解析.vi"("输入"=w1939) -> ("结果"=w1933:string[])  [unwired: 2 out]
                            n301 = call "故障数值解析.vi"("输入"=w1938) -> ("结果"=w1935:string[])  [unwired: 2 out]
                            n302 = Build Array(w1928, w1929, w1930, w1934, w1931, w1932, w1933, w1935) -> (w1937:string[][])
                            n303 = Reshape Array(w1937, 32 ("维数大小")) -> (w1927:string[])
                            n304 = local write "硬件故障"(w1927) -> ()
                            n305 = local write "状态"(TRUE ("状态")) -> ()
                          }
                        }
                        n306 = disable-structure shown="禁用" {
                          disable-tunnel: w1856 -> [w1865 _]
                          frame Disabled {
                            n307 = call "标定授权读取.vi"("VCI_Receive"=w1865) -> ()  [unwired: 1 out]
                          }
                          frame Enabled {
                          }
                        }
                        n308 = call "多帧接收机制(EV05).vi"("can卡类型"=w1864, "设备索引号"=w1863, "CAN端口"=w1862, "VCI_Receive"=w1856, "命令"=u32 133, "板号"=u32 0, "写?"=FALSE) -> ("错误代码"=→"错误代码":i32, "输出数组"=→"输出数组":u8[], "结束信号"=→"结束信号":bool)  [unwired: 1 in, 9 out]
                      }
                    }
                  }
                  frame Error {
                  }
                }
              }
              frame Enabled {
              }
            }
          }
          n309 = Release Queue(queue=w1588, force destroy? (F)=TRUE ("强制销毁？(F)"), error in (no error)=w1587) -> (error out=w1586:errorcluster)  [unwired: 2 out]
          n310 = call <vilib>:"Clear Errors.vi"("error in (no error)"=w1586) -> ()  [unwired: 7 out]
        }
        frame Enabled {
        }
      }
      n311 = while {
        shift-right: [w2075] -> _
        shift-left: w207 -> [w2074]
        shift-left: w207 -> [w2073]
        stop <- w2076 stop-if-true
        n312 = event shown="[2] \"主界面选项\": 值改变" {
          selector: _ -> [_ _ _ _ _ _ _]
          dyn-events: _ -> [_ _ _ _ _ _ _]
          timeout: 50 -> [_ _ _ _ _ _ _]
          tunnel: [_ _ _ _ _ w2255 w2261] -> w2076
          tunnel: [w2081 w2122 w2162 w2196 w2232 w2253 w2260] -> w2075
          tunnel: w2074 -> [w2079 w2122 w2162 w2196 w2232 w2253 w2260]
          tunnel: w2073 -> [w2080 _ _ _ _ _ _]
          event Timeout {
            n313 = event-data() -> ()  [unwired: 3 out]
            n314 = flat-sequence {
              tunnel: w2080 -> [w2084]
              tunnel: w2079 -> [w2082]
              tunnel: [w2082] -> w2078
              tunnel: w2078 -> [w2085]
              frame #0 {
                n315 = Not Equal?(x=w2082, y=w2084) -> (x != y?=w2083:bool)
                n316 = local write "状态"(w2083) -> ()
              }
              frame #1 {
                n317 = Quotient & Remainder(x=w2085, y=2.0) -> (x-y*floor(x/y)=w2087:dbl)  [unwired: 1 out]
                n318 = Equal To 0?(x=w2087) -> (x = 0?=w2088:bool)
                n319 = local write "状态"(w2088) -> ()
              }
            }
            n320 = disable-structure shown="禁用" {
              frame Disabled {
                n321 = control-ref of="单选选项1"() -> (w2094:refnum<vi>)
                n322 = control-ref of="单选选项2 2"() -> (w2092:refnum<vi>)
                n323 = control-ref of="单选选项2 3"() -> (w2091:refnum<vi>)
                n324 = control-ref of="单选选项2 4"() -> (w2090:refnum<vi>)
                n325 = local read "主界面选项"() -> (w2099:enum32{"单选选项1", "单选选项2 2", "单选选项2 3", "单选选项2 4"})
                n326 = Build Array(w2094, w2092, w2091, w2090) -> (w2093:refnum<vi>[])
                n327 = case shown="\"单选选项2 4\"" w2099 {
                  selector: w2099 -> [w2105 w2111 w2116 w2121]
                  tunnel: [w2104 w2110 w2115 w2120] -> w2096
                  tunnel: [w2103 w2109 w2114 w2119] -> w2095
                  tunnel: w2093 -> [w2106 w2108 w2113 w2118]
                  tunnel: [enum32{"电池系统信息", "BMS信息", "充电信息", "故障信息"}."电池系统信息" ("值") enum32{"电池系统信息", "BMS信息", "充电信息", "故障信息"}."BMS信息" ("值") enum32{"电池系统信息", "BMS信息", "充电信息", "故障信息"}."充电信息" ("值") enum32{"电池系统信息", "BMS信息", "充电信息", "故障信息"}."故障信息" ("值")] -> w2089
                  frame "单选选项1", Default {
                    n328 = Delete From Array(array=w2106, index=w2105) -> (deleted portion=w2103:refnum<vi>, array with subset deleted=w2104:refnum<vi>[])  [unwired: 1 in]
                  }
                  frame "单选选项2 2" {
                    n329 = Delete From Array(array=w2108, index=w2111) -> (deleted portion=w2109:refnum<vi>, array with subset deleted=w2110:refnum<vi>[])  [unwired: 1 in]
                  }
                  frame "单选选项2 3" {
                    n330 = Delete From Array(array=w2113, index=w2116) -> (deleted portion=w2114:refnum<vi>, array with subset deleted=w2115:refnum<vi>[])  [unwired: 1 in]
                  }
                  frame "单选选项2 4" {
                    n331 = Delete From Array(array=w2118, index=w2121) -> (deleted portion=w2119:refnum<vi>, array with subset deleted=w2120:refnum<vi>[])  [unwired: 1 in]
                  }
                }
                n332 = local write "选项卡控件"(w2089) -> ()
                n333 = for {
                  tunnel: w2096 -> [w2101] mode=indexing
                  tunnel: u32 16777215 -> [w2100]
                  n334 = property class="Bool (严格)"(reference=w2101, "BoolText.TextColor"=w2100) -> ()  [unwired: 1 in, 2 out]
                }
                n335 = property class="Bool (严格)"(reference=w2095, "BoolText.TextColor"=u32 87470) -> ()  [unwired: 1 in, 2 out]
              }
              frame Enabled {
              }
            }
            n336 = global read "EV05全局变量1.vi" "life"() -> (w2081:dbl)
            "Life:" <- w2081
          }
          event "故障信息选择按键": Value Change {
            n337 = event-data() -> ()  [unwired: 7 out]
            n338 = control-ref of="单选选项1"() -> (w2134:refnum<vi>)
            n339 = control-ref of="单选选项2"() -> (w2127:refnum<vi>)
            n340 = control-ref of="单选选项2 2"() -> (w2128:refnum<vi>)
            n341 = control-ref of="单选选项2 4"() -> (w2130:refnum<vi>)
            n342 = control-ref of="单选选项2 3"() -> (w2129:refnum<vi>)
            n343 = local read "故障信息选择按键"() -> (w2133:T7)
            n344 = Build Array(w2127, w2128, w2129, w2134, w2130) -> (w2131:refnum<vi>[])
            n345 = case shown="\"单选选项1\", 默认" w2133 {
              selector: w2133 -> [w2140 w2145 w2150 w2155 w2160]
              tunnel: [w2139 w2144 w2149 w2154 w2159] -> w2123
              tunnel: [w2138 w2143 w2148 w2153 w2158] -> w2125
              tunnel: w2131 -> [w2141 w2146 w2151 w2156 w2161]
              tunnel: [T8."BMS故障" ("故障信息") T8."电池系统故障" ("故障信息") T8."其他故障" ("故障信息") T8."电池故障" ("故障信息") T8."其他状态" ("故障信息")] -> w2126
              frame "单选选项2" {
                n346 = Delete From Array(array=w2141, index=w2140) -> (deleted portion=w2138:refnum<vi>, array with subset deleted=w2139:refnum<vi>[])  [unwired: 1 in]
              }
              frame "单选选项2 2" {
                n347 = Delete From Array(array=w2146, index=w2145) -> (deleted portion=w2143:refnum<vi>, array with subset deleted=w2144:refnum<vi>[])  [unwired: 1 in]
              }
              frame "单选选项2 3" {
                n348 = Delete From Array(array=w2151, index=w2150) -> (deleted portion=w2148:refnum<vi>, array with subset deleted=w2149:refnum<vi>[])  [unwired: 1 in]
              }
              frame "单选选项1", Default {
                n349 = Delete From Array(array=w2156, index=w2155) -> (deleted portion=w2153:refnum<vi>, array with subset deleted=w2154:refnum<vi>[])  [unwired: 1 in]
              }
              frame "单选选项2 4" {
                n350 = Delete From Array(array=w2161, index=w2160) -> (deleted portion=w2158:refnum<vi>, array with subset deleted=w2159:refnum<vi>[])  [unwired: 1 in]
              }
            }
            n351 = for {
              tunnel: u32 87470 -> [w2136]
              tunnel: w2123 -> [w2135] mode=indexing
              n352 = property class="Bool (严格)"(reference=w2135, "BoolText.TextColor"=w2136) -> ()  [unwired: 1 in, 2 out]
            }
            n353 = property class="Bool (严格)"(reference=w2125, "BoolText.TextColor"=u32 16777215) -> ()  [unwired: 1 in, 2 out]
            n354 = local write "故障信息"(w2126) -> ()
          }
          event "主界面选项": Value Change {
            n355 = event-data() -> ()  [unwired: 7 out]
            n356 = control-ref of="单选选项1"() -> (w2168:refnum<vi>)
            n357 = control-ref of="单选选项2 2"() -> (w2166:refnum<vi>)
            n358 = control-ref of="单选选项2 3"() -> (w2165:refnum<vi>)
            n359 = control-ref of="单选选项2 4"() -> (w2164:refnum<vi>)
            n360 = local read "主界面选项"() -> (w2173:enum32{"单选选项1", "单选选项2 2", "单选选项2 3", "单选选项2 4"})
            n361 = Build Array(w2168, w2166, w2165, w2164) -> (w2167:refnum<vi>[])
            n362 = case shown="\"单选选项2 4\"" w2173 {
              selector: w2173 -> [w2179 w2185 w2190 w2195]
              tunnel: [w2178 w2184 w2189 w2194] -> w2170
              tunnel: [w2177 w2183 w2188 w2193] -> w2169
              tunnel: w2167 -> [w2180 w2182 w2187 w2192]
              tunnel: [enum32{"电池系统信息", "BMS信息", "充电信息", "故障信息"}."电池系统信息" ("值") enum32{"电池系统信息", "BMS信息", "充电信息", "故障信息"}."BMS信息" ("值") enum32{"电池系统信息", "BMS信息", "充电信息", "故障信息"}."充电信息" ("值") enum32{"电池系统信息", "BMS信息", "充电信息", "故障信息"}."故障信息" ("值")] -> w2163
              frame "单选选项1", Default {
                n363 = Delete From Array(array=w2180, index=w2179) -> (deleted portion=w2177:refnum<vi>, array with subset deleted=w2178:refnum<vi>[])  [unwired: 1 in]
              }
              frame "单选选项2 2" {
                n364 = Delete From Array(array=w2182, index=w2185) -> (deleted portion=w2183:refnum<vi>, array with subset deleted=w2184:refnum<vi>[])  [unwired: 1 in]
              }
              frame "单选选项2 3" {
                n365 = Delete From Array(array=w2187, index=w2190) -> (deleted portion=w2188:refnum<vi>, array with subset deleted=w2189:refnum<vi>[])  [unwired: 1 in]
              }
              frame "单选选项2 4" {
                n366 = Delete From Array(array=w2192, index=w2195) -> (deleted portion=w2193:refnum<vi>, array with subset deleted=w2194:refnum<vi>[])  [unwired: 1 in]
              }
            }
            n367 = local write "选项卡控件"(w2163) -> ()
            n368 = for {
              tunnel: w2170 -> [w2175] mode=indexing
              tunnel: u32 16777215 -> [w2174]
              n369 = property class="Bool (严格)"(reference=w2175, "BoolText.TextColor"=w2174) -> ()  [unwired: 1 in, 2 out]
            }
            n370 = property class="Bool (严格)"(reference=w2169, "BoolText.TextColor"=u32 65511) -> ()  [unwired: 1 in, 2 out]
          }
          event "电池信息读取": Value Change {
            n371 = event-data() -> ("NewVal"=w2197:bool)  [unwired: 6 out]
            n372 = disable-structure shown="禁用" {
              disable-tunnel: w2197 -> [w2198 _]
              frame Disabled {
                n373 = case shown="真" w2198 {
                  frame False {
                  }
                  frame True {
                    n374 = local read "设备索引号"() -> (w2206:u8)
                    n375 = local read "can卡类型"() -> (w2207:u8)
                    n376 = local read "CAN端口"() -> (w2205:u8)
                    n377 = call "标定授权发送.vi"("CAN卡类型"=w2207, "解锁类型"=enum16{"读取", "写", "下载"}."读取", "设备索引号"=w2206, "CAN端口"=w2205, "是否连接"=TRUE, "板选择"=0, "FUNC"=u32 1) -> ("发送成功"=w2200:bool)  [unwired: 8 out]
                    n378 = local read "电池信息选项"() -> (w2199:enum16{"电池信息", "历史信息"})
                    n379 = case shown="真" w2200 {
                      tunnel: w2207 -> [_ w2213]
                      tunnel: w2206 -> [_ w2212]
                      tunnel: w2205 -> [_ w2211]
                      tunnel: w2199 -> [_ w2210]
                      frame False {
                      }
                      frame True {
                        n380 = case shown="\"电池信息\", 默认" w2210 {
                          tunnel: [6 4] -> w2209
                          frame "电池信息", Default {
                          }
                          frame "历史信息" {
                          }
                        }
                        n381 = for {
                          N: w2209 -> [_]
                          tunnel: w2213 -> [w2227]
                          tunnel: w2212 -> [w2226]
                          tunnel: w2211 -> [w2225]
                          tunnel: w2210 -> [w2217]
                          i -> [w2219]
                          n382 = case shown="\"电池信息\"" w2217 {
                            tunnel: [u32 131 ("命令") u32 132 ("命令")] -> w2223
                            frame "历史信息" {
                            }
                            frame "电池信息" {
                            }
                          }
                          n383 = Increment(x=w2219) -> (x+1=w2218:i32)
                          n384 = Wait Until Next ms Multiple(millisecond multiple=u32 200 ("毫秒倍数")) -> ()  [unwired: 1 out]
                          n385 = local write "命令"(w2223) -> ()
                          n386 = call "ID组合.vi"("SA(4)"=u32 128 ("命令"), "PS(3)"=u32 0 ("命令"), "PF(2)"=w2223, "PDU(1)"=u32 24 ("命令")) -> ("ID"=w2220:i32)  [unwired: 7 out]
                          n387 = Build Array(1, w2218) -> (w2228:i32[])
                          n388 = call "transmit-8.6.vi"("can卡类型"=w2227, "设备索引号"=w2226, "CAN端口"=w2225, "ID"=w2220, "Data"=w2228) -> ()  [unwired: 4 in, 11 out]
                        }
                        n389 = global write "EV05全局变量1.vi" "超时"(TRUE ("超时")) -> ()
                      }
                    }
                  }
                }
              }
              frame Enabled {
              }
            }
          }
          event "读取其它状态": Value Change {
            n390 = event-data() -> ("NewVal"=w2233:bool)  [unwired: 6 out]
            n391 = case shown="真" w2233 {
              frame False {
              }
              frame True {
                n392 = disable-structure shown="启用" {
                  frame Disabled {
                    n393 = local read "设备索引号"() -> (w2240:u8)
                    n394 = local read "can卡类型"() -> (w2241:u8)
                    n395 = local read "CAN端口"() -> (w2239:u8)
                    n396 = call "标定授权发送.vi"("CAN卡类型"=w2241, "解锁类型"=enum16{"读取", "写", "下载"}."读取", "设备索引号"=w2240, "CAN端口"=w2239, "是否连接"=TRUE, "板选择"=0, "FUNC"=u32 1) -> ("发送成功"=w2234:bool)  [unwired: 8 out]
                    n397 = case shown="真" w2234 {
                      tunnel: w2241 -> [_ w2245]
                      tunnel: w2240 -> [_ w2244]
                      tunnel: w2239 -> [_ w2243]
                      frame False {
                      }
                      frame True {
                        n398 = local read "状态选择"() -> (w2250:T9)
                        n399 = Increment(x=w2250) -> (x+1=w2248:T9)
                        n400 = Build Array(1, w2248) -> (w2247:i32[])
                        n401 = global write "EV05全局变量1.vi" "超时"(TRUE ("超时")) -> ()
                        n402 = call "transmit-8.6.vi"("can卡类型"=w2245, "设备索引号"=w2244, "CAN端口"=w2243, "ID"=u32 411369600 ("命令"), "Data"=w2247) -> ()  [unwired: 4 in, 11 out]
                      }
                    }
                  }
                  frame Enabled {
                    n403 = One Button Dialog(message="请功能暂未开放,请联系技术人员" ("消息"), button name ("OK")="确定" ("按钮名称（“确定”）")) -> ()  [unwired: 1 out]
                  }
                }
              }
            }
          }
          event "停止": Value Change {
            n404 = event-data() -> ("NewVal"=w2255:bool)  [unwired: 6 out]
            n405 = disable-structure shown="启用" {
              disable-tunnel: w2255 -> [_ _]
              frame Disabled {
                n406 = property class="VI"("FP.State"=T11."Hidden" ("前面板窗口:状态")) -> (reference out=w2257:refnum<vi>, error out=w2256:errorcluster)  [unwired: 2 in]
                n407 = property class="VI"(reference=w2257, error in=w2256, "Front Panel.Open"=FALSE ("前面板窗口:打开")) -> ()  [unwired: 2 out]
              }
              frame Enabled {
              }
            }
            n408 = local write "停止"(TRUE ("停止")) -> ()
          }
          event Panel Close? {
            w2261 = TRUE ("NewVal")
            n409 = event-data() -> ()  [unwired: 5 out]
            n410 = disable-structure shown="启用" {
              disable-tunnel: w2261 -> [_ _]
              frame Disabled {
                n411 = property class="VI"("FP.State"=T11."Hidden" ("前面板窗口:状态")) -> (reference out=w2264:refnum<vi>, error out=w2263:errorcluster)  [unwired: 2 in]
                n412 = property class="VI"(reference=w2264, error in=w2263, "Front Panel.Open"=FALSE ("前面板窗口:打开")) -> ()  [unwired: 2 out]
              }
              frame Enabled {
              }
            }
            n413 = local write "停止"(w2261) -> ()
            n414 = event-data("Discard?"=TRUE ("放弃？")) -> ()  [unwired: 1 in, 1 out]
          }
        }
      }
      n415 = property on="单选选项2 4" class="Bool (严格)"("Visible"=w206) -> ()  [unwired: 2 in, 2 out]
      n416 = property on="读取其它状态" class="Bool (严格)"("Visible"=w206) -> ()  [unwired: 2 in, 2 out]
      n417 = property on="状态选择" class="Enum (严格)"("Visible"=w206) -> ()  [unwired: 2 in, 2 out]
      n418 = property on="加热器状态" class="Ring (严格)"("Visible"=w206) -> ()  [unwired: 2 in, 2 out]
      n419 = property on="正绝缘电阻(kΩ)" class="DigNum (严格)"("Visible"=w206) -> ()  [unwired: 2 in, 2 out]
      n420 = property on="风机转速" class="DigNum (严格)"("Visible"=w206) -> ()  [unwired: 2 in, 2 out]
      n421 = property on="预充电时间" class="DigNum (严格)"("Visible"=w206) -> ()  [unwired: 2 in, 2 out]
      n422 = property on="风机状态" class="Ring (严格)"("Visible"=w206) -> ()  [unwired: 2 in, 2 out]
      n423 = property on="负绝缘电阻(kΩ)" class="DigNum (严格)"("Visible"=w206) -> ()  [unwired: 2 in, 2 out]
      n424 = control-ref of="详细信息"() -> ()  [unwired: 1 out]
      n425 = local write "状态"(w213) -> ()
      n426 = local write "停止"(w213) -> ()
      n427 = local write "结束信号"(w213) -> ()
      n428 = property on="严重故障干接点" class="Ring (严格)"("Visible"=w206) -> ()  [unwired: 2 in, 2 out]
      n429 = property on="液位传感器状态" class="Ring (严格)"("Visible"=w206) -> ()  [unwired: 2 in, 2 out]
      n430 = property on="高压互锁状态" class="Ring (严格)"("Visible"=w206) -> ()  [unwired: 2 in, 2 out]
      n431 = property on="维护开关状态" class="Ring (严格)"("Visible"=w206) -> ()  [unwired: 2 in, 2 out]
      n432 = property on="烟雾报警器状态" class="Ring (严格)"("Visible"=w206) -> ()  [unwired: 2 in, 2 out]
      n433 = property on="电池箱锁止机构状态" class="Ring (严格)"("Visible"=w206) -> ()  [unwired: 2 in, 2 out]
      n434 = property on="压力传感器状态" class="Ring (严格)"("Visible"=w206) -> ()  [unwired: 2 in, 2 out]
      n435 = property on="湿度传感器状态" class="Ring (严格)"("Visible"=w206) -> ()  [unwired: 2 in, 2 out]
      n436 = property on="手动维护开关" class="Ring (严格)"("Visible"=w206) -> ()  [unwired: 2 in, 2 out]
      n437 = property on="碰撞开关状态" class="Ring (严格)"("Visible"=w206) -> ()  [unwired: 2 in, 2 out]
      n438 = call "自适应屏幕分辨率.vi"() -> ()  [unwired: 16 in]
      n439 = disable-structure shown="禁用" {
        frame Disabled {
          n440 = while {
            stop <- w254 stop-if-true
            n441 = local read "结束信号"() -> (w255:bool)
            n442 = local read "停止"() -> (w254:bool)
            n443 = Wait Until Next ms Multiple(millisecond multiple=u32 200 ("毫秒倍数")) -> ()  [unwired: 1 out]
            n444 = case shown="真" w255 {
              frame False {
              }
              frame True {
                n445 = local read "选项卡控件"() -> (w257:enum32{"电池系统信息", "BMS信息", "充电信息", "故障信息"})
                n446 = local read "输出数组"() -> (w256:u8[])
                n447 = local write "结束信号"(FALSE ("结束信号")) -> ()
                n448 = case shown="\"电池系统信息\", 默认" w257 {
                  tunnel: w256 -> [_ w260]
                  frame "电池系统信息", Default {
                  }
                  frame "故障信息" {
                    n449 = local read "状态选择"() -> (w261:T9)
                    n450 = case shown="\"CAN检测\"" w261 {
                      tunnel: w260 -> [w265 w290 w312 w336 w357 w378 w402]
                      tunnel: [w263 w288 w310 w334 w355 w376 w400] -> _
                      tunnel: [w262 w287 w309 w333 w354 w375 w399] -> _
                      tunnel: [_ _ _ _ _ _ FALSE] -> w259
                      frame "电压检测,内总电压检测,外总电压检测,温度检测,电流检测,绝缘检测", Default {
                        w264 = string[] [] ("类型")
                        n451 = for {
                          N: 6 -> [_]
                          tunnel: w265 -> [w280]
                          shift-right: [w270] -> w263
                          shift-left: w264 -> [w272]
                          shift-right: [w267] -> w262
                          shift-left: w264 -> [w269]
                          i -> [w276]
                          n452 = Multiply(x=w276, y=2) -> (x*y=w274:i32)
                          n453 = case shown="5" w276 {
                            tunnel: [T10."电压检测" ("枚举") T10."外总电压检测" ("枚举") T10."内总电压检测" ("枚举") T10."温度检测" ("枚举") T10."电流检测" ("枚举") T10."绝缘检测" ("枚举")] -> w279
                            frame 0, Default {
                            }
                            frame 1 {
                            }
                            frame 2 {
                            }
                            frame 3 {
                            }
                            frame 4 {
                            }
                            frame 5 {
                            }
                          }
                          n454 = Increment(x=w274) -> (x+1=w273:i32)
                          n455 = Index Array(array=w280, index #1=w274, index #2=w273) -> (element #1=w278:u8, element #2=w277:u8)
                          n456 = call "故障分类表.vi"("低位"=w277, "高位"=w278, "枚举"=w279) -> ("状态"=w268:string[], "类型"=w271:string[])  [unwired: 7 out]
                          n457 = Insert Into Array(array=w272, new element=w271) -> (w270:string[])  [unwired: 1 in]
                          n458 = Insert Into Array(array=w269, new element=w268) -> (w267:string[])  [unwired: 1 in]
                        }
                      }
                      frame "内部EE存储器,外部EE存储器,外部FLASH存储器" {
                        w289 = string[] [] ("类型")
                        n459 = for {
                          N: 3 -> [_]
                          tunnel: w290 -> [w305]
                          shift-right: [w295] -> w288
                          shift-left: w289 -> [w297]
                          shift-right: [w292] -> w287
                          shift-left: w289 -> [w294]
                          i -> [w301]
                          n460 = case shown="0, 默认" w301 {
                            tunnel: [T10."内部EE存储器" ("枚举") T10."外部EE存储器" ("枚举") T10."外部Flash存储器" ("枚举")] -> w304
                            frame 0, Default {
                            }
                            frame 1 {
                            }
                            frame 2 {
                            }
                          }
                          n461 = Multiply(x=w301, y=2) -> (x*y=w299:i32)
                          n462 = Increment(x=w299) -> (x+1=w298:i32)
                          n463 = Index Array(array=w305, index #1=w299, index #2=w298) -> (element #1=w303:u8, element #2=w302:u8)
                          n464 = call "故障分类表.vi"("低位"=w302, "高位"=w303, "枚举"=w304) -> ("状态"=w293:string[], "类型"=w296:string[])  [unwired: 7 out]
                          n465 = Insert Into Array(array=w297, new element=w296) -> (w295:string[])  [unwired: 1 in]
                          n466 = Insert Into Array(array=w294, new element=w293) -> (w292:string[])  [unwired: 1 in]
                        }
                      }
                      frame "CAN检测" {
                        w311 = string[] [] ("类型")
                        n467 = for {
                          N: 5 -> [_]
                          tunnel: w312 -> [w327]
                          shift-right: [w317] -> w310
                          shift-left: w311 -> [w319]
                          shift-right: [w314] -> w309
                          shift-left: w311 -> [w316]
                          i -> [w323]
                          n468 = case shown="4" w323 {
                            tunnel: [T10."CAN0检测" ("枚举") T10."CAN1检测" ("枚举") T10."CAN4检测" ("枚举") T10."CAN2检测" ("枚举") T10."CAN3检测" ("枚举")] -> w326
                            frame 0, Default {
                            }
                            frame 1 {
                            }
                            frame 2 {
                            }
                            frame 3 {
                            }
                            frame 4 {
                            }
                          }
                          n469 = Multiply(x=w323, y=2) -> (x*y=w321:i32)
                          n470 = Increment(x=w321) -> (x+1=w320:i32)
                          n471 = Index Array(array=w327, index #1=w321, index #2=w320) -> (element #1=w325:u8, element #2=w324:u8)
                          n472 = call "故障分类表.vi"("低位"=w324, "高位"=w325, "枚举"=w326) -> ("状态"=w315:string[], "类型"=w318:string[])  [unwired: 7 out]
                          n473 = Insert Into Array(array=w319, new element=w318) -> (w317:string[])  [unwired: 1 in]
                          n474 = Insert Into Array(array=w316, new element=w315) -> (w314:string[])  [unwired: 1 in]
                        }
                      }
                      frame "CPU,软件" {
                        w335 = string[] [] ("类型")
                        n475 = for {
                          N: 2 -> [_]
                          tunnel: w336 -> [w351]
                          shift-right: [w341] -> w334
                          shift-left: w335 -> [w343]
                          shift-right: [w338] -> w333
                          shift-left: w335 -> [w340]
                          i -> [w347]
                          n476 = case shown="0, 默认" w347 {
                            tunnel: [T10."CPU" ("枚举") T10."软件" ("枚举")] -> w350
                            frame 0, Default {
                            }
                            frame 1 {
                            }
                          }
                          n477 = Multiply(x=w347, y=2) -> (x*y=w345:i32)
                          n478 = Increment(x=w345) -> (x+1=w344:i32)
                          n479 = Index Array(array=w351, index #1=w345, index #2=w344) -> (element #1=w349:u8, element #2=w348:u8)
                          n480 = call "故障分类表.vi"("低位"=w348, "高位"=w349, "枚举"=w350) -> ("状态"=w339:string[], "类型"=w342:string[])  [unwired: 7 out]
                          n481 = Insert Into Array(array=w343, new element=w342) -> (w341:string[])  [unwired: 1 in]
                          n482 = Insert Into Array(array=w340, new element=w339) -> (w338:string[])  [unwired: 1 in]
                        }
                      }
                      frame "RS485,RS232检测" {
                        w356 = string[] [] ("类型")
                        n483 = for {
                          N: 2 -> [_]
                          tunnel: w357 -> [w372]
                          shift-right: [w362] -> w355
                          shift-left: w356 -> [w364]
                          shift-right: [w359] -> w354
                          shift-left: w356 -> [w361]
                          i -> [w368]
                          n484 = case shown="1" w368 {
                            tunnel: [T10."RS485检测" ("枚举") T10."RS232检测" ("枚举")] -> w371
                            frame 0, Default {
                            }
                            frame 1 {
                            }
                          }
                          n485 = Multiply(x=w368, y=2) -> (x*y=w366:i32)
                          n486 = Increment(x=w366) -> (x+1=w365:i32)
                          n487 = Index Array(array=w372, index #1=w366, index #2=w365) -> (element #1=w370:u8, element #2=w369:u8)
                          n488 = call "故障分类表.vi"("低位"=w369, "高位"=w370, "枚举"=w371) -> ("状态"=w360:string[], "类型"=w363:string[])  [unwired: 7 out]
                          n489 = Insert Into Array(array=w364, new element=w363) -> (w362:string[])  [unwired: 1 in]
                          n490 = Insert Into Array(array=w361, new element=w360) -> (w359:string[])  [unwired: 1 in]
                        }
                      }
                      frame "DI,DO,AI,AO检测" {
                        w377 = string[] [] ("类型")
                        n491 = for {
                          N: 4 -> [_]
                          tunnel: w378 -> [w393]
                          shift-right: [w383] -> w376
                          shift-left: w377 -> [w385]
                          shift-right: [w380] -> w375
                          shift-left: w377 -> [w382]
                          i -> [w389]
                          n492 = case shown="3" w389 {
                            tunnel: [T10."DI" ("枚举") T10."DO" ("枚举") T10."AI" ("枚举") T10."AO" ("枚举")] -> w392
                            frame 0, Default {
                            }
                            frame 1 {
                            }
                            frame 2 {
                            }
                            frame 3 {
                            }
                          }
                          n493 = Multiply(x=w389, y=2) -> (x*y=w387:i32)
                          n494 = Increment(x=w387) -> (x+1=w386:i32)
                          n495 = Index Array(array=w393, index #1=w387, index #2=w386) -> (element #1=w391:u8, element #2=w390:u8)
                          n496 = call "故障分类表.vi"("低位"=w390, "高位"=w391, "枚举"=w392) -> ("状态"=w381:string[], "类型"=w384:string[])  [unwired: 7 out]
                          n497 = Insert Into Array(array=w385, new element=w384) -> (w383:string[])  [unwired: 1 in]
                          n498 = Insert Into Array(array=w382, new element=w381) -> (w380:string[])  [unwired: 1 in]
                        }
                      }
                      frame "预充电故障,电池不匹配,充电异常故障" {
                        w401 = string[] [] ("类型")
                        n499 = for {
                          N: 3 -> [_]
                          tunnel: w402 -> [w417]
                          shift-right: [w407] -> w400
                          shift-left: w401 -> [w409]
                          shift-right: [w404] -> w399
                          shift-left: w401 -> [w406]
                          i -> [w413]
                          n500 = case shown="0, 默认" w413 {
                            tunnel: [T10."预充电故障" ("枚举") T10."电池不匹配" ("枚举") T10."充电异常" ("枚举")] -> w416
                            frame 0, Default {
                            }
                            frame 1 {
                            }
                            frame 2 {
                            }
                          }
                          n501 = Multiply(x=w413, y=2) -> (x*y=w411:i32)
                          n502 = Increment(x=w411) -> (x+1=w410:i32)
                          n503 = Index Array(array=w417, index #1=w411, index #2=w410) -> (element #1=w415:u8, element #2=w414:u8)
                          n504 = call "故障分类表.vi"("低位"=w414, "高位"=w415, "枚举"=w416) -> ("状态"=w405:string[], "类型"=w408:string[])  [unwired: 7 out]
                          n505 = Insert Into Array(array=w409, new element=w408) -> (w407:string[])  [unwired: 1 in]
                          n506 = Insert Into Array(array=w406, new element=w405) -> (w404:string[])  [unwired: 1 in]
                        }
                      }
                    }
                    n507 = local write "读取其它状态"(w259) -> ()
                  }
                }
              }
            }
          }
        }
        frame Enabled {
        }
      }
      n508 = while {
        stop <- w423 stop-if-true
        n509 = local read "停止"() -> (w423:bool)
        n510 = local read "选项卡控件"() -> (w422:enum32{"电池系统信息", "BMS信息", "充电信息", "故障信息"})
        n511 = global read "中英文全局.vi" "中英文选择"() -> (w421:enum32{"中文", "English"})
        n512 = case shown="\"BMS信息\"" w422 {
          tunnel: w421 -> [_ w536 w624 w789]
          frame "电池系统信息", Default {
            n513 = disable-structure shown="启用" {
              disable-tunnel: [w482 w499] -> w459
              disable-tunnel: [w481 w498] -> w458
              disable-tunnel: [w480 w497] -> w457
              disable-tunnel: [w479 w496] -> w456
              disable-tunnel: [w478 w495] -> w455
              disable-tunnel: [w477 w492] -> w454
              disable-tunnel: [w476 w491] -> w453
              disable-tunnel: [w475 w490] -> w452
              disable-tunnel: [w474 w489] -> w451
              disable-tunnel: [w473 w488] -> w450
              disable-tunnel: [w472 w505] -> w449
              disable-tunnel: [w471 w504] -> w448
              disable-tunnel: [w470 w503] -> w447
              disable-tunnel: [w469 w502] -> w446
              disable-tunnel: [w468 w501] -> w445
              disable-tunnel: [w467 w500] -> w444
              disable-tunnel: [w466 w487] -> w443
              disable-tunnel: [w465 w486] -> w442
              frame Disabled {
                n514 = control-ref of="详细信息"() -> (w464:refnum<vi>)
                n515 = property class="Clust (严格)"(reference=w464) -> ("Value"=w463:T2)  [unwired: 1 in, 2 out]
                n516 = Unbundle(w463) -> ("平均电流"=w482:dbl, "最大充电电流"=w481:dbl, "最大放电电流"=w480:dbl, "实际容量"=w479:dbl, "充电总安时"=w478:dbl, "放电总安时"=w477:dbl, "正绝缘电阻"=w476:dbl, "负绝缘电阻"=w475:dbl, "功率"=w474:dbl, "从板个数"=w473:dbl, "辅助A继电器"=w484:dbl, "辅助B继电器"=w483:dbl, "DO1"=w472:string, "DO2"=w471:string, "DI1"=w470:string, "DI2"=w469:string, "DI3"=w468:string, "DI4"=w467:string, "AI1"=w466:dbl, "AI2"=w465:dbl, "外总压"=w485:dbl)
                n517 = local write "辅助继电器B(heat)"(w483) -> ()
                n518 = local write "外总压(V)"(w485) -> ()
                n519 = local write "辅助继电器A(fan)"(w484) -> ()
              }
              frame Enabled {
                n520 = global read "电池信息全局变量.vi" "放电总安时"() -> (w492:dbl)
                n521 = global read "电池信息全局变量.vi" "从板个数"() -> (w488:dbl)
                n522 = global read "电池信息全局变量.vi" "最大充电电流"() -> (w498:dbl)
                n523 = global read "电池信息全局变量.vi" "最大放电电流"() -> (w497:dbl)
                n524 = global read "电池信息全局变量.vi" "充电总安时"() -> (w495:dbl)
                n525 = global read "电池信息全局变量.vi" "正绝缘"() -> (w491:dbl)
                n526 = global read "电池信息全局变量.vi" "负绝缘"() -> (w490:dbl)
                n527 = global read "电池信息全局变量.vi" "平均电流"() -> (w499:dbl)
                n528 = global read "电池信息全局变量.vi" "实际容量"() -> (w496:dbl)
                n529 = global read "电池信息全局变量.vi" "AI2"() -> (w486:dbl)
                n530 = global read "电池信息全局变量.vi" "功率"() -> (w489:dbl)
                n531 = global read "电池信息全局变量.vi" "AI1"() -> (w487:dbl)
                n532 = global read "电池信息全局变量.vi" "DO"() -> (w494:string[])
                n533 = global read "电池信息全局变量.vi" "DI"() -> (w493:string[])
                n534 = Index Array(array=w494) -> (element #3=w505:string, element #4=w504:string)  [unwired: 4 in, 2 out]
                n535 = Index Array(array=w493) -> (element #1=w503:string, element #2=w502:string, element #3=w501:string, element #4=w500:string)  [unwired: 4 in]
              }
            }
            n536 = global read "电池信息全局变量.vi" "电池信息解析"() -> (w427:dbl[])
            n537 = Wait Until Next ms Multiple(millisecond multiple=u32 500 ("毫秒倍数")) -> ()  [unwired: 1 out]
            n538 = Index Array(array=w427) -> (element #1=w441:dbl, element #2=w436:dbl, element #3=w434:dbl, element #4=w429:dbl, element #5=w428:dbl)  [unwired: 5 in]
            n539 = local write "风机转速"(w428) -> ()
            n540 = call "二进制解析-8.6.vi"("索引"=8, "数值"=w434) -> ("低位子数组"=w433:i32[])  [unwired: 3 out]
            n541 = local write "预充电时间"(w429) -> ()
            n542 = call "二进制解析-8.6.vi"("索引"=8, "数值"=w436) -> ("低位子数组"=w432:i32[])  [unwired: 3 out]
            n543 = call "二进制解析-8.6.vi"("索引"=8, "数值"=w441) -> ("低位子数组"=w440:i32[])  [unwired: 3 out]
            n544 = for {
              N: 4 -> [_]
              tunnel: w433 -> [w509]
              i -> [w507]
              w511 = 2 ("y")
              n545 = Multiply(x=w507, y=w511) -> (x*y=w510:i32)
              n546 = Array Subset(array=w509, index=w510, length=w511) -> (w508:i32[])
              n547 = call "数值二进制转十进制-8.6.vi"("子数组"=w508) -> ("十进制数值"=w506:i32)  [unwired: 4 out]
              n548 = case shown="3" w507 {
                tunnel: w506 -> [w512 w513 w514 w515]
                frame 0, Default {
                  n549 = local write "压力传感器状态"(w512) -> ()
                }
                frame 1 {
                  n550 = local write "湿度传感器状态"(w513) -> ()
                }
                frame 2 {
                  n551 = local write "手动维护开关"(w514) -> ()
                }
                frame 3 {
                  n552 = local write "碰撞开关状态"(w515) -> ()
                }
              }
            }
            n553 = for {
              N: 4 -> [_]
              tunnel: w432 -> [w519]
              i -> [w517]
              w521 = 2 ("y")
              n554 = Multiply(x=w517, y=w521) -> (x*y=w520:i32)
              n555 = Array Subset(array=w519, index=w520, length=w521) -> (w518:i32[])
              n556 = call "数值二进制转十进制-8.6.vi"("子数组"=w518) -> ("十进制数值"=w516:i32)  [unwired: 4 out]
              n557 = case shown="3" w517 {
                tunnel: w516 -> [w522 w523 w524 w525]
                frame 0, Default {
                  n558 = local write "高压互锁状态"(w522) -> ()
                }
                frame 1 {
                  n559 = local write "维护开关状态"(w523) -> ()
                }
                frame 2 {
                  n560 = local write "烟雾报警器状态"(w524) -> ()
                }
                frame 3 {
                  n561 = local write "电池箱锁止机构状态"(w525) -> ()
                }
              }
            }
            n562 = for {
              N: 4 -> [_]
              tunnel: w440 -> [w529]
              i -> [w527]
              w531 = 2 ("y")
              n563 = Multiply(x=w527, y=w531) -> (x*y=w530:i32)
              n564 = Array Subset(array=w529, index=w530, length=w531) -> (w528:i32[])
              n565 = call "数值二进制转十进制-8.6.vi"("子数组"=w528) -> ("十进制数值"=w526:i32)  [unwired: 4 out]
              n566 = case shown="2" w527 {
                tunnel: w526 -> [w532 w533 w534 w535]
                frame 0, Default {
                  n567 = local write "液位传感器状态"(w532) -> ()
                }
                frame 1 {
                  n568 = local write "风机状态"(w533) -> ()
                }
                frame 2 {
                  n569 = local write "加热器状态"(w534) -> ()
                }
                frame 3 {
                  n570 = local write "严重故障干接点"(w535) -> ()
                }
              }
            }
            n571 = local read "主界面其他信息"() -> (w461:T5)
            n572 = Bundle(cluster=w461, "平均电流(A)"=w459, "最大充电电流(A)"=w458, "最大放电电流(A)"=w457, "实际容量(Ah)"=w456, "充电总安时(Ah)"=w455, "放电总安时(Ah)"=w454, "正绝缘电阻(kΩ)"=w453, "负绝缘电阻(kΩ)"=w452, "功率(kW)"=w451, "从板个数"=w450, "DO1"=w449, "DO2"=w448, "DI1"=w447, "DI2"=w446, "DI3"=w445, "DI4"=w444, "AI1(V)"=w443, "AI2(V)"=w442) -> (w460:T5)
            n573 = local write "主界面其他信息"(w460) -> ()
            n574 = global read "电池信息全局变量.vi" "辅助继电器A"() -> (w426:dbl)
            n575 = global read "电池信息全局变量.vi" "辅助继电器B"() -> (w425:dbl)
            n576 = global read "电池信息全局变量.vi" "外总压"() -> (w424:dbl)
            n577 = local write "辅助继电器A(fan)"(w426) -> ()
            n578 = local write "辅助继电器B(heat)"(w425) -> ()
            n579 = local write "外总压(V)"(w424) -> ()
          }
          frame "故障信息" {
            n580 = case shown="\"English\"" w536 {
              tunnel: [string[] ["正接触器粘连", "正接触器不能吸合", "带载切断总正继电器故障", "带载切断总负继电器故障", "负接触器粘连", "负接触器不能吸合", "预充电接触器粘连", "预充电接触器不能吸合", "DC/DC继电器粘连", "DC/DC继电器不能吸合", "高压互锁失效", "高压互锁异常", "充电接触器粘连", "充电接触器不能吸合", "充电继电器故障", "极柱温度高于上限值", "预充电", "保留", "保留", "保留", "风机堵路", "风机开路", "加热不能开启", "加热不能关闭", "加热器温度高于上限值", "进风口温度过高", "进风口温度过低", "进风口,出风口温差故障", "出风口温度过高", "出风口温度过低", "保留", "保留"] ("名称") string[] ["pos_adjoin", "pos_not_pickup", "curr_open_pos_relay", "curr_open_pos_relay", "neg_adjoin", "neg_not_pickup", "pre_adjoin", "pro_not_pickup", "dcdc_adjoin", "dcdc_not_pickup", "HVIL_fail", "HVIL_abnormal", "chg_adjoin", "chg_not_pcikup", "cur_open_chg_relay", "spot_high", "pre_chg_error", "rsv", "rsv", "rsv", "fan_off", "fan_on", "heat_not_on", "heat_not_off", "heat_t_high", "inlet_t_high", "inlet_t_low", "air_det_t", "outlet_t_high", "outlet_t_low", "rsv", "rsv"] ("名称")] -> w550
              frame "中文", Default {
              }
              frame "English" {
              }
            }
            n581 = case shown="\"English\"" w536 {
              tunnel: [string[] ["电压检测模块故障", "温度检测模块故障", "电流检测模块故障", "绝缘检测模块故障", "内总电压检测模块故障", "外总电压检测模块故障", "系统外扩时钟模块故障", "CPU内部EE故障", "EE存储器故障", "45db041存储器故障", "CPU内部FLASH存储器故障", "CPU故障", "CAN4通信模块故障", "CAN0通信模块故障", "CAN1通信模块故障", "保留", "保留", "保留", "保留", "保留", "充电均衡模块故障", "放电均衡模块故障", "保留", "软件故障", "保留", "保留", "保留", "保留", "DI模块故障", "DO模块故障", "保留", "保留"] ("名称") string[] ["detection_cellv", "detection_temper", "detection_curr", "detection_iso", "detection_sumv_in", "detection_sumv_out", "detection_exterm_clock", "detection_ee_cpu", "detection_ee_ext", "detection_flash_ext", "detection_flash_cpu", "cpu_error", "detection_can4", "detection_can0", "detection_can1", "rsv", "rsv", "rsv", "rsv", "rsv", "detection_chg_bal", "detection_dch_bal", "rsv", "soft_error", "rsv", "rsv", "rsv", "rsv", "DI_error", "DO_error", "rsv", "rsv"] ("名称")] -> w549
              frame "中文", Default {
              }
              frame "English" {
              }
            }
            n582 = case shown="\"English\"" w536 {
              tunnel: [string[] ["下电故障", "供电电源过压", "供电电源欠压", "保留", "保留", "保留", "保留", "保留", "保留", "碰撞传感器报警", "保留", "烟雾报警器故障", "保留", "保留", "保留", "保留", "绝缘故障偏正极", "绝缘故障偏负极", "绝缘故障中间侧", "绝缘故障(未分位置)"] ("名称") string[] ["shutdown", "supply_v_high", "supply_y_low", "rsv", "rsv", "rsv", "rsv", "rsv", "rsv", "Collision sensor alarm", "rsv", "smoke_alarm", "rsv", "rsv", "rsv", "rsv", "iso_pos", "iso_neg", "iso_mid", "iso_error"] ("名称")] -> w548
              frame "中文", Default {
              }
              frame "English" {
              }
            }
            n583 = case shown="\"English\"" w536 {
              tunnel: [string[] ["总电压过压", "总电压欠压", "单体电压过压", "单体电压欠压", "单箱压差过大", "整组压差过大", "单箱温差过大", "整组温差过大", "温度过高", "温度过低", "充电电流过高", "放电电流过高", "回馈过流", "保留", "SOC过高", "SOC过低", "保留", "保留", "保留", "箱间平均电压不一致", "电池组号不一致", "保留", "保留", "保留", "箱间SOC不一致", "保留", "保留", "保留", "整体电池容量低", "保留", "保留", "保留"] ("名称") string[] ["sumv_high", "sumv_low", "cellv_high", "cellv_low", "det_v_single", "det_v_all", "det_t_single", "det_t_all", "t_high", "t_low", "chg_curr_high", "dch_curr_high", "Feedback_curr_high", "rsv", "SOC_high", "SOC_low", "rsv", "rsv", "rsv", "average_v_diff", "bat_group_diff", "rsv", "rsv", "rsv", "SOC_diff", "rsv", "rsv", "rsv", "bat_cap_low", "rsv", "rsv", "rsv"] ("名称")] -> w551
              frame "中文", Default {
              }
              frame "English" {
              }
            }
            n584 = Wait Until Next ms Multiple(millisecond multiple=u32 500 ("毫秒倍数")) -> ()  [unwired: 1 out]
            n585 = global read "电池信息全局变量.vi" "电池系统故障"() -> (w543:string[])
            n586 = global read "电池信息全局变量.vi" "其他故障"() -> (w541:string[])
            n587 = global read "电池信息全局变量.vi" "电池故障"() -> (w544:string[])
            n588 = global read "电池信息全局变量.vi" "硬件故障"() -> (w542:string[])
            n589 = call "故障分解2.vi"("名称"=w551, "故障输入口"=w544) -> ("故障等级"=w552:dbl, "输出数组"=w540:string[][])  [unwired: 1 in, 1 out]
            n590 = call "故障分解2.vi"("名称"=w550, "故障输入口"=w543) -> ("故障等级"=w547:dbl, "输出数组"=w539:string[][])  [unwired: 1 in, 1 out]
            n591 = call "故障分解2.vi"("名称"=w548, "故障输入口"=w541) -> ("故障等级"=w545:dbl, "输出数组"=→"其他故障":string[][])  [unwired: 1 in, 1 out]
            n592 = call "故障分解2.vi"("名称"=w549, "故障输入口"=w542) -> ("故障等级"=w546:dbl, "输出数组"=→"硬件故障 2":string[][])  [unwired: 1 in, 1 out]
            n593 = case shown="0, 默认" w552 {
              frame 0, Default {
                n594 = property on="电池故障显示" class="Bool (严格)"("Visible"=TRUE ("可见"), "Value"=FALSE ("电池故障显示")) -> ()  [unwired: 2 in, 2 out]
                n595 = property on="二级故障 2" class="Bool (严格)"("Visible"=FALSE ("可见"), "Value"=FALSE ("二级故障 2")) -> ()  [unwired: 2 in, 2 out]
              }
              frame 1 {
                n596 = property on="电池故障显示" class="Bool (严格)"("Visible"=TRUE ("可见"), "Value"=TRUE ("电池故障显示")) -> ()  [unwired: 2 in, 2 out]
                n597 = property on="二级故障 2" class="Bool (严格)"("Visible"=FALSE ("可见"), "Value"=FALSE ("二级故障 2")) -> ()  [unwired: 2 in, 2 out]
              }
              frame 2 {
                n598 = property on="二级故障 2" class="Bool (严格)"("Visible"=TRUE ("可见"), "Value"=FALSE ("二级故障 2")) -> ()  [unwired: 2 in, 2 out]
                n599 = property on="电池故障显示" class="Bool (严格)"("Visible"=FALSE ("可见"), "Value"=FALSE ("电池故障显示")) -> ()  [unwired: 2 in, 2 out]
              }
              frame 3 {
                n600 = property on="二级故障 2" class="Bool (严格)"("Visible"=TRUE ("可见"), "Value"=TRUE ("二级故障 2")) -> ()  [unwired: 2 in, 2 out]
                n601 = property on="电池故障显示" class="Bool (严格)"("Visible"=FALSE ("可见"), "Value"=FALSE ("电池故障显示")) -> ()  [unwired: 2 in, 2 out]
              }
            }
            n602 = case shown="0, 默认" w547 {
              frame 0, Default {
                w594 = FALSE ("可见")
                n603 = property on="电池系统故障显示" class="Bool (严格)"("Visible"=TRUE ("可见"), "Value"=FALSE ("电池系统故障显示")) -> ()  [unwired: 2 in, 2 out]
                n604 = property on="二级故障 3" class="Bool (严格)"("Visible"=w594, "Value"=w594) -> ()  [unwired: 2 in, 2 out]
              }
              frame 1 {
                w597 = FALSE ("可见")
                n605 = property on="电池系统故障显示" class="Bool (严格)"("Visible"=TRUE ("可见"), "Value"=TRUE ("电池系统故障显示")) -> ()  [unwired: 2 in, 2 out]
                n606 = property on="二级故障 3" class="Bool (严格)"("Visible"=w597, "Value"=w597) -> ()  [unwired: 2 in, 2 out]
              }
              frame 2 {
                n607 = property on="电池系统故障显示" class="Bool (严格)"("Visible"=FALSE ("可见"), "Value"=FALSE ("电池系统故障显示")) -> ()  [unwired: 2 in, 2 out]
                n608 = property on="二级故障 3" class="Bool (严格)"("Visible"=TRUE ("可见"), "Value"=FALSE ("二级故障 3")) -> ()  [unwired: 2 in, 2 out]
              }
              frame 3 {
                n609 = property on="电池系统故障显示" class="Bool (严格)"("Visible"=FALSE ("可见"), "Value"=FALSE ("电池系统故障显示")) -> ()  [unwired: 2 in, 2 out]
                n610 = property on="二级故障 3" class="Bool (严格)"("Visible"=TRUE ("可见"), "Value"=TRUE ("二级故障 3")) -> ()  [unwired: 2 in, 2 out]
              }
            }
            n611 = case shown="3" w546 {
              frame 0, Default {
                n612 = property on="BMS故障显示" class="Bool (严格)"("Visible"=TRUE ("可见"), "Value"=FALSE ("BMS故障显示")) -> ()  [unwired: 2 in, 2 out]
                n613 = property on="二级故障 4" class="Bool (严格)"("Visible"=FALSE ("可见"), "Value"=FALSE ("二级故障 4")) -> ()  [unwired: 2 in, 2 out]
              }
              frame 1 {
                n614 = property on="BMS故障显示" class="Bool (严格)"("Visible"=TRUE ("可见"), "Value"=TRUE ("BMS故障显示")) -> ()  [unwired: 2 in, 2 out]
                n615 = property on="二级故障 4" class="Bool (严格)"("Visible"=FALSE ("可见"), "Value"=FALSE ("二级故障 4")) -> ()  [unwired: 2 in, 2 out]
              }
              frame 2 {
                n616 = property on="BMS故障显示" class="Bool (严格)"("Visible"=FALSE ("可见"), "Value"=FALSE ("BMS故障显示")) -> ()  [unwired: 2 in, 2 out]
                n617 = property on="二级故障 4" class="Bool (严格)"("Visible"=TRUE ("可见"), "Value"=FALSE ("二级故障 4")) -> ()  [unwired: 2 in, 2 out]
              }
              frame 3 {
                n618 = property on="BMS故障显示" class="Bool (严格)"("Visible"=FALSE ("可见"), "Value"=FALSE ("BMS故障显示")) -> ()  [unwired: 2 in, 2 out]
                n619 = property on="二级故障 4" class="Bool (严格)"("Visible"=TRUE ("可见"), "Value"=TRUE ("二级故障 4")) -> ()  [unwired: 2 in, 2 out]
              }
            }
            n620 = local write "电池故障"(w540) -> ()
            n621 = case shown="3" w545 {
              frame 0, Default {
                n622 = property on="其他故障显示" class="Bool (严格)"("Visible"=TRUE ("可见"), "Value"=FALSE ("其他故障显示")) -> ()  [unwired: 2 in, 2 out]
                n623 = property on="二级故障 5" class="Bool (严格)"("Visible"=FALSE ("可见"), "Value"=FALSE ("二级故障 5")) -> ()  [unwired: 2 in, 2 out]
              }
              frame 1 {
                n624 = property on="其他故障显示" class="Bool (严格)"("Visible"=TRUE ("可见"), "Value"=TRUE ("其他故障显示")) -> ()  [unwired: 2 in, 2 out]
                n625 = property on="二级故障 5" class="Bool (严格)"("Visible"=FALSE ("可见"), "Value"=FALSE ("二级故障 5")) -> ()  [unwired: 2 in, 2 out]
              }
              frame 2 {
                n626 = property on="其他故障显示" class="Bool (严格)"("Visible"=FALSE ("可见"), "Value"=FALSE ("其他故障显示")) -> ()  [unwired: 2 in, 2 out]
                n627 = property on="二级故障 5" class="Bool (严格)"("Visible"=TRUE ("可见"), "Value"=FALSE ("二级故障 5")) -> ()  [unwired: 2 in, 2 out]
              }
              frame 3 {
                n628 = property on="其他故障显示" class="Bool (严格)"("Visible"=FALSE ("可见"), "Value"=FALSE ("其他故障显示")) -> ()  [unwired: 2 in, 2 out]
                n629 = property on="二级故障 5" class="Bool (严格)"("Visible"=TRUE ("可见"), "Value"=TRUE ("二级故障 5")) -> ()  [unwired: 2 in, 2 out]
              }
            }
            n630 = local write "硬件故障 2"(w539) -> ()
          }
          frame "BMS信息" {
            n631 = global read "EV05全局变量1.vi" "BMS时间"() -> (w628:string)
            n632 = global read "电池信息全局变量.vi" "10"() -> (w630:string[])
            n633 = global read "电池信息全局变量.vi" "F"() -> (w629:dbl[])
            n634 = call <vilib>:"Space Constant.vi"() -> ("String"=w645:string)
            n635 = Index Array(array=w630) -> (element #1=w652:string, element #2=w650:string, element #3=w648:string)  [unwired: 3 in]
            n636 = Wait Until Next ms Multiple(millisecond multiple=u32 500 ("毫秒倍数")) -> ()  [unwired: 1 out]
            n637 = Index Array(array=w629) -> (element #1=w643:dbl, element #2=w642:dbl, element #3=w641:dbl, element #4=w640:dbl, element #5=w638:dbl, element #6=w635:dbl)  [unwired: 6 in]
            n638 = Match Pattern(string=w628, regular expression=w645) -> (before substring=w632:string, after substring=w644:string)  [unwired: 3 out]
            n639 = call <vilib>:"Space Constant.vi"() -> ("String"=w647:string)
            n640 = global read "电池信息全局变量.vi" "07"() -> (w631:dbl)
            n641 = Decimal String To Number(string=w652) -> (number=w651:i32)  [unwired: 3 out]
            n642 = Match Pattern(string=w648, regular expression=w647) -> (before substring=w633:string, after substring=w646:string)  [unwired: 3 out]
            n643 = local write "BMS当前系统时间2"(w632) -> ()
            n644 = local write "当前系统时间"(w644) -> ()
            n645 = Decimal String To Number(string=w650) -> (number=w649:i32)  [unwired: 3 out]
            n646 = Format Into String(format string="%#f" ("格式字符串"), w635) -> (resulting string=w634:string)  [unwired: 2 in, 1 out]
            n647 = Format Into String(format string="%#f" ("格式字符串"), w638) -> (resulting string=w637:string)  [unwired: 2 in, 1 out]
            n648 = local write "BMS当前系统时间2 2"(w633) -> ()
            n649 = local write "上次停机时间"(w646) -> ()
            n650 = call "二进制解析-8.6.vi"("索引"=8, "数值"=w631) -> ("低位子数组"=w671:i32[])  [unwired: 3 out]
            n651 = local write "内网总线负载率"(w637) -> ()
            n652 = local write "供电电源电压(V)"(w634) -> ()
            n653 = for {
              N: 4 -> [_]
              tunnel: w671 -> [w782]
              i -> [w780]
              w784 = 2 ("y")
              n654 = Multiply(x=w780, y=w784) -> (x*y=w783:i32)
              n655 = Array Subset(array=w782, index=w783, length=w784) -> (w781:i32[])
              n656 = call "数值二进制转十进制-8.6.vi"("子数组"=w781) -> ("十进制数值"=w779:i32)  [unwired: 4 out]
              n657 = case shown="3" w780 {
                tunnel: w779 -> [w785 w786 w787 w788]
                frame 0, Default {
                  n658 = local write "内部CAN总线状态"(w785) -> ()
                }
                frame 1 {
                  n659 = local write "整车CAN总线状态"(w786) -> ()
                }
                frame 2 {
                  n660 = local write "充电CAN总线状态"(w787) -> ()
                }
                frame 3 {
                  n661 = local write "标准CAN总线状态"(w788) -> ()
                }
              }
            }
            n662 = call "二进制解析-8.6.vi"("索引"=6, "数值"=w649) -> ("高位子数组"=w627:i32[])  [unwired: 3 out]
            n663 = call "二进制解析-8.6.vi"("索引"=8, "数值"=w642) -> ("低位子数组"=w662:i32[])  [unwired: 3 out]
            n664 = call "二进制解析-8.6.vi"("索引"=8, "数值"=w640) -> ("低位子数组"=w655:i32[])  [unwired: 3 out]
            n665 = call "二进制解析-8.6.vi"("索引"=8, "数值"=w651) -> ("低位子数组"=w666:i32[])  [unwired: 3 out]
            n666 = call "二进制解析-8.6.vi"("索引"=8, "数值"=w643) -> ("低位子数组"=w661:i32[])  [unwired: 3 out]
            n667 = call "二进制解析-8.6.vi"("索引"=8, "数值"=w641) -> ("低位子数组"=w656:i32[])  [unwired: 3 out]
            n668 = call "数值二进制转十进制-8.6.vi"("子数组"=w627) -> ("十进制数值"=w626:i32)  [unwired: 4 out]
            n669 = for {
              N: 2 -> [_]
              tunnel: w655 -> [w686]
              i -> [w684]
              w688 = 2 ("y")
              n670 = Multiply(x=w684, y=w688) -> (x*y=w687:i32)
              n671 = Array Subset(array=w686, index=w687, length=w688) -> (w685:i32[])
              n672 = call "数值二进制转十进制-8.6.vi"("子数组"=w685) -> ("十进制数值"=w683:i32)  [unwired: 4 out]
              n673 = case shown="1" w684 {
                tunnel: w683 -> [_ w689 _ _]
                frame 0, Default {
                }
                frame 1 {
                  n674 = local write "供电电源状态"(w689) -> ()
                }
                frame 2 {
                }
                frame 3 {
                }
              }
            }
            n675 = for {
              N: 4 -> [_]
              tunnel: w662 -> [w703]
              i -> [w701]
              w705 = 2 ("y")
              n676 = Multiply(x=w701, y=w705) -> (x*y=w704:i32)
              n677 = Array Subset(array=w703, index=w704, length=w705) -> (w702:i32[])
              n678 = call "数值二进制转十进制-8.6.vi"("子数组"=w702) -> ("十进制数值"=w700:i32)  [unwired: 4 out]
              n679 = case shown="3" w701 {
                tunnel: w700 -> [w706 w707 w708 w709]
                frame 0, Default {
                  n680 = local write "绝缘检测模块状态"(w706) -> ()
                }
                frame 1 {
                  n681 = local write "电流模块模块状态"(w707) -> ()
                }
                frame 2 {
                  n682 = local write "电池充电均衡模块状态"(w708) -> ()
                }
                frame 3 {
                  n683 = local write "电池放电均衡模块状态"(w709) -> ()
                }
              }
            }
            n684 = for {
              N: 4 -> [_]
              tunnel: w666 -> [w724]
              tunnel: w624 -> [w720]
              i -> [w722]
              w726 = 2 ("y")
              n685 = Multiply(x=w722, y=w726) -> (x*y=w725:i32)
              n686 = Array Subset(array=w724, index=w725, length=w726) -> (w723:i32[])
              n687 = call "数值二进制转十进制-8.6.vi"("子数组"=w723) -> ("十进制数值"=w721:i32)  [unwired: 4 out]
              n688 = case shown="3" w722 {
                tunnel: w721 -> [w729 w742 w755 w768]
                tunnel: w720 -> [w727 w741 w754 w767]
                frame 0, Default {
                  n689 = case shown="\"中文\", 默认" w727 {
                    tunnel: [w731 w736] -> w728
                    tunnel: w729 -> [w730 w735]
                    frame "中文", Default {
                      n690 = case shown="3" w730 {
                        tunnel: ["未唤醒" "唤醒" "无效"] -> w731
                        frame 0, Default {
                        }
                        frame 1 {
                        }
                        frame 3 {
                        }
                      }
                    }
                    frame "English" {
                      n691 = case shown="3" w735 {
                        tunnel: ["Not WakeUp" "WakeUp" "Invalid"] -> w736
                        frame 0, Default {
                        }
                        frame 1 {
                        }
                        frame 3 {
                        }
                      }
                    }
                  }
                  n692 = local write "Key_on"(w728) -> ()
                }
                frame 1 {
                  n693 = case shown="\"中文\", 默认" w741 {
                    tunnel: [w744 w749] -> w740
                    tunnel: w742 -> [w743 w748]
                    frame "中文", Default {
                      n694 = case shown="3" w743 {
                        tunnel: ["未唤醒" "唤醒" "无效"] -> w744
                        frame 0, Default {
                        }
                        frame 1 {
                        }
                        frame 3 {
                        }
                      }
                    }
                    frame "English" {
                      n695 = case shown="3" w748 {
                        tunnel: ["Not WakeUp" "WakeUp" "Invalid"] -> w749
                        frame 0, Default {
                        }
                        frame 1 {
                        }
                        frame 3 {
                        }
                      }
                    }
                  }
                  n696 = local write "慢充"(w740) -> ()
                }
                frame 2 {
                  n697 = case shown="\"中文\", 默认" w754 {
                    tunnel: [w757 w762] -> w753
                    tunnel: w755 -> [w756 w761]
                    frame "中文", Default {
                      n698 = case shown="3" w756 {
                        tunnel: ["未唤醒" "唤醒" "无效"] -> w757
                        frame 0, Default {
                        }
                        frame 1 {
                        }
                        frame 3 {
                        }
                      }
                    }
                    frame "English" {
                      n699 = case shown="3" w761 {
                        tunnel: ["Not WakeUp" "WakeUp" "Invalid"] -> w762
                        frame 0, Default {
                        }
                        frame 1 {
                        }
                        frame 3 {
                        }
                      }
                    }
                  }
                  n700 = local write "快充"(w753) -> ()
                }
                frame 3 {
                  n701 = case shown="\"中文\", 默认" w767 {
                    tunnel: [w770 w775] -> w766
                    tunnel: w768 -> [w769 w774]
                    frame "中文", Default {
                      n702 = case shown="3" w769 {
                        tunnel: ["未唤醒" "唤醒" "无效"] -> w770
                        frame 0, Default {
                        }
                        frame 1 {
                        }
                        frame 3 {
                        }
                      }
                    }
                    frame "English" {
                      n703 = case shown="3" w774 {
                        tunnel: ["Not WakeUp" "WakeUp" "Invalid"] -> w775
                        frame 0, Default {
                        }
                        frame 1 {
                        }
                        frame 3 {
                        }
                      }
                    }
                  }
                  n704 = local write "自唤醒"(w766) -> ()
                }
              }
            }
            n705 = for {
              N: 4 -> [_]
              tunnel: w661 -> [w713]
              i -> [w711]
              w715 = 2 ("y")
              n706 = Multiply(x=w711, y=w715) -> (x*y=w714:i32)
              n707 = Array Subset(array=w713, index=w714, length=w715) -> (w712:i32[])
              n708 = call "数值二进制转十进制-8.6.vi"("子数组"=w712) -> ("十进制数值"=w710:i32)  [unwired: 4 out]
              n709 = case shown="3" w711 {
                tunnel: w710 -> [w716 w717 w718 w719]
                frame 0, Default {
                  n710 = local write "温度模块检测状态"(w716) -> ()
                }
                frame 1 {
                  n711 = local write "内部总电压检测模块状态"(w717) -> ()
                }
                frame 2 {
                  n712 = local write "外部总电压检测模块状态"(w718) -> ()
                }
                frame 3 {
                  n713 = local write "电压模块检测状态"(w719) -> ()
                }
              }
            }
            n714 = for {
              N: 4 -> [_]
              tunnel: w656 -> [w693]
              i -> [w691]
              w695 = 2 ("y")
              n715 = Multiply(x=w691, y=w695) -> (x*y=w694:i32)
              n716 = Array Subset(array=w693, index=w694, length=w695) -> (w692:i32[])
              n717 = call "数值二进制转十进制-8.6.vi"("子数组"=w692) -> ("十进制数值"=w690:i32)  [unwired: 4 out]
              n718 = case shown="0, 默认" w691 {
                tunnel: w690 -> [w696 w697 w698 w699]
                frame 0, Default {
                  n719 = local write "系统时钟状态"(w696) -> ()
                }
                frame 1 {
                  n720 = local write "Flash存储器状态"(w697) -> ()
                }
                frame 2 {
                  n721 = local write "外部EE存储器状态"(w698) -> ()
                }
                frame 3 {
                  n722 = local write "内部EE存储器状态"(w699) -> ()
                }
              }
            }
            n723 = case shown="\"中文\", 默认" w624 {
              tunnel: [w674 w679] -> w625
              tunnel: w626 -> [w673 w678]
              frame "中文", Default {
                n724 = case shown="3" w673 {
                  tunnel: ["未唤醒" "唤醒" "无效"] -> w674
                  frame 0, Default {
                  }
                  frame 1 {
                  }
                  frame 3 {
                  }
                }
              }
              frame "English" {
                n725 = case shown="3" w678 {
                  tunnel: ["Not WakeUp" "WakeUp" "Invalid"] -> w679
                  frame 0, Default {
                  }
                  frame 1 {
                  }
                  frame 3 {
                  }
                }
              }
            }
            n726 = local write "CAN唤醒"(w625) -> ()
          }
          frame "充电信息" {
            w803 = "%#f" ("格式字符串")
            n727 = global read "电池信息全局变量.vi" "CP"() -> (w815:u8)
            n728 = global read "电池信息全局变量.vi" "CC2"() -> (→"检测点2 CC2(V)":dbl)
            n729 = global read "电池信息全局变量.vi" "CC"() -> (→"检测点4 CC(V)":dbl)
            n730 = global read "电池信息全局变量.vi" "列1"() -> (w798:dbl[])
            n731 = case shown="0..100" w815 {
              selector: w815 -> [_ w1584]
              tunnel: [u8 100 ("PWM检测点3 CP(%)") w1584] -> w814
              frame 101.., Default {
              }
              frame 0..100 {
              }
            }
            "PWM检测点3 CP(%)" <- w814
            n732 = Wait Until Next ms Multiple(millisecond multiple=u32 500 ("毫秒倍数")) -> ()  [unwired: 1 out]
            n733 = Index Array(array=w798) -> (element #1=w797:dbl, element #2=w796:dbl, element #3=w790:dbl, element #4=w791:dbl, element #5=w792:dbl, element #6=w795:dbl, element #7=w794:dbl, element #8=w793:dbl)  [unwired: 8 in]
            n734 = stacked-sequence {
              tunnel: w797 -> [w843 _]
              tunnel: w796 -> [w835 _]
              tunnel: w795 -> [w834 _]
              tunnel: w794 -> [w833 _]
              tunnel: w793 -> [w832 _]
              tunnel: w792 -> [_ w1190]
              tunnel: w791 -> [_ w1189]
              tunnel: w790 -> [_ w1187]
              tunnel: w789 -> [w819 w1177]
              frame #0 {
                w827 = "" ("trimmed string")
                n735 = call "二进制解析-8.6.vi"("索引"=8, "数值"=w832) -> ("低位子数组"=w829:i32[])  [unwired: 3 out]
                n736 = call "二进制解析-8.6.vi"("索引"=8, "数值"=w833) -> ("低位子数组"=w828:i32[])  [unwired: 3 out]
                n737 = call "二进制解析-8.6.vi"("索引"=8, "数值"=w834) -> ("低位子数组"=w840:i32[])  [unwired: 3 out]
                n738 = call "二进制解析-8.6.vi"("索引"=8, "数值"=w835) -> ("低位子数组"=w844:i32[])  [unwired: 3 out]
                n739 = call "二进制解析-8.6.vi"("索引"=8, "数值"=w843) -> ("低位子数组"=w842:i32[])  [unwired: 3 out]
                n740 = for {
                  N: 4 -> [_]
                  tunnel: w829 -> [w854]
                  tunnel: [w850] -> _ mode=indexing
                  shift-right: [w849] -> w825
                  shift-left: w827 -> [w848]
                  tunnel: w819 -> [w847]
                  i -> [w852]
                  w850 = 2 ("y")
                  n741 = Multiply(x=w852, y=w850) -> (x*y=w855:i32)
                  n742 = Array Subset(array=w854, index=w855, length=w850) -> (w853:i32[])
                  n743 = call "数值二进制转十进制-8.6.vi"("子数组"=w853) -> ("十进制数值"=w851:i32)  [unwired: 4 out]
                  n744 = case shown="\"English\"" w847 {
                    tunnel: w852 -> [w859 w894]
                    tunnel: w851 -> [w858 w893]
                    tunnel: [w857 w892] -> w849
                    tunnel: w848 -> [w856 w891]
                    frame "中文", Default {
                      n745 = case shown="3" w859 {
                        tunnel: w858 -> [w862 w870 w878 w886]
                        tunnel: [w861 w869 w877 w885] -> w857
                        tunnel: w856 -> [w860 w868 w876 w884]
                        frame 0, Default {
                          n746 = case shown="1" w862 {
                            tunnel: [w863 w864] -> w861
                            tunnel: w860 -> [w863 w866]
                            frame 0, Default {
                            }
                            frame 1 {
                              (unwired) "\n"
                              n747 = call <vilib>:"Space Constant.vi"() -> ()  [unwired: 1 out]
                              n748 = call <vilib>:"Space Constant.vi"() -> ("String"=w865:string)
                              n749 = Concatenate Strings(w866, "充电机急停故障", w865) -> (w864:string)
                            }
                          }
                        }
                        frame 1 {
                          n750 = case shown="1" w870 {
                            tunnel: [w871 w872] -> w869
                            tunnel: w868 -> [w871 w874]
                            frame 0, Default {
                            }
                            frame 1 {
                              n751 = call <vilib>:"Space Constant.vi"() -> ("String"=w873:string)
                              n752 = Concatenate Strings(w874, "电压异常", w873) -> (w872:string)
                            }
                          }
                        }
                        frame 2 {
                          n753 = case shown="1" w878 {
                            tunnel: [w879 w880] -> w877
                            tunnel: w876 -> [w879 w882]
                            frame 0, Default {
                            }
                            frame 1 {
                              n754 = Concatenate Strings(w882, "电流不匹配", "\n") -> (w880:string)
                            }
                          }
                        }
                        frame 3 {
                          n755 = case shown="1" w886 {
                            tunnel: [w887 w888] -> w885
                            tunnel: w884 -> [w887 w889]
                            frame 0, Default {
                            }
                            frame 1 {
                              n756 = Concatenate Strings(w889, "其他故障") -> (w888:string)
                            }
                          }
                        }
                      }
                    }
                    frame "English" {
                      n757 = case shown="3" w894 {
                        tunnel: w893 -> [w897 w905 w913 w921]
                        tunnel: [w896 w904 w912 w920] -> w892
                        tunnel: w891 -> [w895 w903 w911 w919]
                        frame 0, Default {
                          n758 = case shown="1" w897 {
                            tunnel: [w898 w899] -> w896
                            tunnel: w895 -> [w898 w901]
                            frame 0, Default {
                            }
                            frame 1 {
                              (unwired) "\n"
                              n759 = call <vilib>:"Space Constant.vi"() -> ()  [unwired: 1 out]
                              n760 = call <vilib>:"Space Constant.vi"() -> ("String"=w900:string)
                              n761 = Concatenate Strings(w901, "Charger fault stop", w900) -> (w899:string)
                            }
                          }
                        }
                        frame 1 {
                          n762 = case shown="1" w905 {
                            tunnel: [w906 w907] -> w904
                            tunnel: w903 -> [w906 w909]
                            frame 0, Default {
                            }
                            frame 1 {
                              n763 = call <vilib>:"Space Constant.vi"() -> ("String"=w908:string)
                              n764 = Concatenate Strings(w909, "Abnormal voltage", w908) -> (w907:string)
                            }
                          }
                        }
                        frame 2 {
                          n765 = case shown="1" w913 {
                            tunnel: [w914 w915] -> w912
                            tunnel: w911 -> [w914 w917]
                            frame 0, Default {
                            }
                            frame 1 {
                              n766 = Concatenate Strings(w917, "Current mismatch\\", "\n") -> (w915:string)
                            }
                          }
                        }
                        frame 3 {
                          n767 = case shown="1" w921 {
                            tunnel: [w922 w923] -> w920
                            tunnel: w919 -> [w922 w924]
                            frame 0, Default {
                            }
                            frame 1 {
                              n768 = Concatenate Strings(w924, "Other faults") -> (w923:string)
                            }
                          }
                        }
                      }
                    }
                  }
                }
                n769 = for {
                  N: 4 -> [_]
                  tunnel: w828 -> [w933]
                  tunnel: [w929] -> _ mode=indexing
                  shift-right: [w928] -> w826
                  shift-left: w827 -> [w927]
                  tunnel: w819 -> [w926]
                  i -> [w931]
                  w929 = 2 ("y")
                  n770 = Multiply(x=w931, y=w929) -> (x*y=w934:i32)
                  n771 = Array Subset(array=w933, index=w934, length=w929) -> (w932:i32[])
                  n772 = call "数值二进制转十进制-8.6.vi"("子数组"=w932) -> ("十进制数值"=w930:i32)  [unwired: 4 out]
                  n773 = case shown="\"English\"" w926 {
                    tunnel: w931 -> [w938 w973]
                    tunnel: w930 -> [w937 w972]
                    tunnel: [w936 w971] -> w928
                    tunnel: w927 -> [w935 w970]
                    frame "中文", Default {
                      n774 = case shown="3" w938 {
                        tunnel: w937 -> [w941 w949 w957 w965]
                        tunnel: [w940 w948 w956 w964] -> w936
                        tunnel: w935 -> [w939 w947 w955 w963]
                        frame 0, Default {
                          n775 = case shown="1" w941 {
                            tunnel: [w942 w943] -> w940
                            tunnel: w939 -> [w942 w945]
                            frame 0, Default {
                            }
                            frame 1 {
                              n776 = Concatenate Strings(w945, "充电机过温", "\n") -> (w943:string)
                            }
                          }
                        }
                        frame 1 {
                          n777 = case shown="1" w949 {
                            tunnel: [w950 w951] -> w948
                            tunnel: w947 -> [w950 w953]
                            frame 0, Default {
                            }
                            frame 1 {
                              n778 = Concatenate Strings(w953, "充电连接器故障", "\n") -> (w951:string)
                            }
                          }
                        }
                        frame 2 {
                          n779 = case shown="1" w957 {
                            tunnel: [w958 w959] -> w956
                            tunnel: w955 -> [w958 w961]
                            frame 0, Default {
                            }
                            frame 1 {
                              n780 = Concatenate Strings(w961, "充电机内部过温", "\n") -> (w959:string)
                            }
                          }
                        }
                        frame 3 {
                          n781 = case shown="1" w965 {
                            tunnel: [w966 w967] -> w964
                            tunnel: w963 -> [w966 w968]
                            frame 0, Default {
                            }
                            frame 1 {
                              n782 = Concatenate Strings(w968, "所需电量不能传送") -> (w967:string)
                            }
                          }
                        }
                      }
                    }
                    frame "English" {
                      n783 = case shown="1" w973 {
                        tunnel: w972 -> [w976 w984 w992 w1000]
                        tunnel: [w975 w983 w991 w999] -> w971
                        tunnel: w970 -> [w974 w982 w990 w998]
                        frame 0, Default {
                          n784 = case shown="1" w976 {
                            tunnel: [w977 w978] -> w975
                            tunnel: w974 -> [w977 w980]
                            frame 0, Default {
                            }
                            frame 1 {
                              n785 = Concatenate Strings(w980, "Charger over temperature", "\n") -> (w978:string)
                            }
                          }
                        }
                        frame 1 {
                          n786 = case shown="1" w984 {
                            tunnel: [w985 w986] -> w983
                            tunnel: w982 -> [w985 w988]
                            frame 0, Default {
                            }
                            frame 1 {
                              n787 = Concatenate Strings(w988, "The charging connector fault", "\n") -> (w986:string)
                            }
                          }
                        }
                        frame 2 {
                          n788 = case shown="1" w992 {
                            tunnel: [w993 w994] -> w991
                            tunnel: w990 -> [w993 w996]
                            frame 0, Default {
                            }
                            frame 1 {
                              n789 = Concatenate Strings(w996, "A charger internal temperature", "\n") -> (w994:string)
                            }
                          }
                        }
                        frame 3 {
                          n790 = case shown="1" w1000 {
                            tunnel: [w1001 w1002] -> w999
                            tunnel: w998 -> [w1001 w1003]
                            frame 0, Default {
                            }
                            frame 1 {
                              n791 = Concatenate Strings(w1003, "The required power cannot be transferred") -> (w1002:string)
                            }
                          }
                        }
                      }
                    }
                  }
                }
                n792 = for {
                  N: 4 -> [_]
                  tunnel: w842 -> [w1124]
                  tunnel: w819 -> [w1120]
                  i -> [w1122]
                  w1126 = 2 ("y")
                  n793 = Multiply(x=w1122, y=w1126) -> (x*y=w1125:i32)
                  n794 = Array Subset(array=w1124, index=w1125, length=w1126) -> (w1123:i32[])
                  n795 = call "数值二进制转十进制-8.6.vi"("子数组"=w1123) -> ("十进制数值"=w1121:i32)  [unwired: 4 out]
                  n796 = case shown="2" w1122 {
                    tunnel: w1121 -> [w1129 w1142 w1155 w1168]
                    tunnel: w1120 -> [w1127 w1140 w1153 w1166]
                    frame 0, Default {
                      n797 = case shown="\"English\"" w1127 {
                        tunnel: w1129 -> [w1131 w1136]
                        tunnel: [w1130 w1135] -> w1128
                        frame "中文", Default {
                          n798 = case shown="1" w1131 {
                            tunnel: ["允许充电" "禁止充电" "无效"] -> w1130
                            frame 1 {
                            }
                            frame 0, Default {
                            }
                            frame 3 {
                            }
                          }
                        }
                        frame "English" {
                          n799 = case shown="0, 默认" w1136 {
                            tunnel: ["Pmt_Chg" "forbid_chg" "Invalid"] -> w1135
                            frame 1 {
                            }
                            frame 0, Default {
                            }
                            frame 3 {
                            }
                          }
                        }
                      }
                      n800 = local write "充电允许控制状态"(w1128) -> ()
                    }
                    frame 1 {
                      n801 = case shown="\"English\"" w1140 {
                        tunnel: w1142 -> [w1144 w1149]
                        tunnel: [w1143 w1148] -> w1141
                        frame "中文", Default {
                          n802 = case shown="0, 默认" w1144 {
                            tunnel: ["消失" "存在" "无效"] -> w1143
                            frame 0, Default {
                            }
                            frame 1 {
                            }
                            frame 3 {
                            }
                          }
                        }
                        frame "English" {
                          n803 = case shown="1" w1149 {
                            tunnel: ["disappear" "There" "Invalid"] -> w1148
                            frame 0, Default {
                            }
                            frame 1 {
                            }
                            frame 3 {
                            }
                          }
                        }
                      }
                      n804 = local write "慢充电信号状态"(w1141) -> ()
                    }
                    frame 2 {
                      n805 = case shown="\"English\"" w1153 {
                        tunnel: w1155 -> [w1157 w1162]
                        tunnel: [w1156 w1161] -> w1154
                        frame "中文", Default {
                          n806 = case shown="0, 默认" w1157 {
                            tunnel: ["无效" "16A" "32A"] -> w1156
                            frame 0, Default {
                            }
                            frame 1 {
                            }
                            frame 2 {
                            }
                          }
                        }
                        frame "English" {
                          n807 = case shown="0, 默认" w1162 {
                            tunnel: ["Invalid" "16A" "32A"] -> w1161
                            frame 0, Default {
                            }
                            frame 1 {
                            }
                            frame 2 {
                            }
                          }
                        }
                      }
                      n808 = local write "交流充电接口容量"(w1154) -> ()
                    }
                    frame 3 {
                      n809 = case shown="\"English\"" w1166 {
                        tunnel: w1168 -> [w1170 w1174]
                        tunnel: [w1169 w1173] -> w1167
                        frame "中文", Default {
                          n810 = case shown="0, 默认" w1170 {
                            tunnel: ["不连接" "连接"] -> w1169
                            frame 0, Default {
                            }
                            frame 1 {
                            }
                          }
                        }
                        frame "English" {
                          n811 = case shown="1" w1174 {
                            tunnel: ["Not_Connect" "Connect"] -> w1173
                            frame 0, Default {
                            }
                            frame 1 {
                            }
                          }
                        }
                      }
                      n812 = local write "充电接口连接状态"(w1167) -> ()
                    }
                  }
                }
                n813 = for {
                  N: 3 -> [_]
                  tunnel: w844 -> [w1071]
                  tunnel: w819 -> [w1070]
                  i -> [w1072]
                  n814 = case shown="0, 默认" w1072 {
                    tunnel: w1071 -> [w1077 w1084 w1109]
                    tunnel: w1070 -> [_ w1078 w1103]
                    frame 0, Default {
                      n815 = Array Subset(array=w1077, index=0 ("索引"), length=2 ("长度")) -> (w1074:i32[])
                      n816 = call "数值二进制转十进制-8.6.vi"("子数组"=w1074) -> ("十进制数值"=w1073:i32)  [unwired: 4 out]
                      n817 = local write "充电状态"(w1073) -> ()
                      n818 = local write "下拉列表"(w1073) -> ()
                    }
                    frame 1 {
                      n819 = Array Subset(array=w1084, index=2 ("索引"), length=4 ("长度")) -> (w1081:i32[])
                      n820 = call "数值二进制转十进制-8.6.vi"("子数组"=w1081) -> ("十进制数值"=w1080:i32)  [unwired: 4 out]
                      n821 = case shown="\"English\"" w1078 {
                        tunnel: w1080 -> [w1086 w1095]
                        tunnel: [w1085 w1094] -> w1079
                        frame "中文", Default {
                          n822 = case shown="6" w1086 {
                            tunnel: ["无效" "预加热" "预充" "恒流" "恒压" "准备结束" "结束"] -> w1085
                            frame 0, Default {
                            }
                            frame 1 {
                            }
                            frame 2 {
                            }
                            frame 3 {
                            }
                            frame 4 {
                            }
                            frame 5 {
                            }
                            frame 6 {
                            }
                          }
                        }
                        frame "English" {
                          n823 = case shown="5" w1095 {
                            tunnel: ["Invalid" "Preheating" "Priming" "Constant_Curr" "Constant_V" "ready to end" "End"] -> w1094
                            frame 0, Default {
                            }
                            frame 1 {
                            }
                            frame 2 {
                            }
                            frame 3 {
                            }
                            frame 4 {
                            }
                            frame 5 {
                            }
                            frame 6 {
                            }
                          }
                        }
                      }
                      n824 = local write "充电阶段"(w1079) -> ()
                    }
                    frame 2 {
                      n825 = Array Subset(array=w1109, index=6 ("索引"), length=2 ("长度")) -> (w1106:i32[])
                      n826 = call "数值二进制转十进制-8.6.vi"("子数组"=w1106) -> ("十进制数值"=w1105:i32)  [unwired: 4 out]
                      n827 = case shown="\"English\"" w1103 {
                        tunnel: w1105 -> [w1111 w1116]
                        tunnel: [w1110 w1115] -> w1104
                        frame "中文", Default {
                          n828 = case shown="0, 默认" w1111 {
                            tunnel: ["正常" "异常" "无效"] -> w1110
                            frame 0, Default {
                            }
                            frame 1 {
                            }
                            frame 3 {
                            }
                          }
                        }
                        frame "English" {
                          n829 = case shown="3" w1116 {
                            tunnel: ["Normal" "Abnormal" "Invalid"] -> w1115
                            frame 0, Default {
                            }
                            frame 1 {
                            }
                            frame 3 {
                            }
                          }
                        }
                      }
                      n830 = local write "充电机状态"(w1104) -> ()
                    }
                  }
                }
                n831 = for {
                  N: 4 -> [_]
                  tunnel: w840 -> [w1012]
                  tunnel: [w1008] -> _ mode=indexing
                  shift-right: [w1007] -> w830
                  shift-left: w827 -> [w1006]
                  tunnel: w819 -> [w1005]
                  i -> [w1010]
                  w1008 = 2 ("y")
                  n832 = Multiply(x=w1010, y=w1008) -> (x*y=w1013:i32)
                  n833 = Array Subset(array=w1012, index=w1013, length=w1008) -> (w1011:i32[])
                  n834 = call "数值二进制转十进制-8.6.vi"("子数组"=w1011) -> ("十进制数值"=w1009:i32)  [unwired: 4 out]
                  n835 = case shown="\"English\"" w1005 {
                    tunnel: w1010 -> [w1017 w1045]
                    tunnel: w1009 -> [w1016 w1044]
                    tunnel: [w1015 w1043] -> w1007
                    tunnel: w1006 -> [w1014 w1042]
                    frame "中文", Default {
                      n836 = case shown="1" w1017 {
                        tunnel: w1016 -> [_ w1021 w1029 w1037]
                        tunnel: [w1018 w1020 w1028 w1036] -> w1015
                        tunnel: w1014 -> [w1018 w1019 w1027 w1035]
                        frame 0, Default {
                        }
                        frame 1 {
                          n837 = case shown="1" w1021 {
                            tunnel: [w1022 w1023] -> w1020
                            tunnel: w1019 -> [w1022 w1025]
                            frame 0, Default {
                            }
                            frame 1 {
                              n838 = Concatenate Strings(w1025, "达到充电机设定条件", "\n") -> (w1023:string)
                            }
                          }
                        }
                        frame 2 {
                          n839 = case shown="1" w1029 {
                            tunnel: [w1030 w1031] -> w1028
                            tunnel: w1027 -> [w1030 w1033]
                            frame 0, Default {
                            }
                            frame 1 {
                              n840 = Concatenate Strings(w1033, "人工中止", "\n") -> (w1031:string)
                            }
                          }
                        }
                        frame 3 {
                          n841 = case shown="1" w1037 {
                            tunnel: [w1038 w1039] -> w1036
                            tunnel: w1035 -> [w1038 w1040]
                            frame 0, Default {
                            }
                            frame 1 {
                              n842 = Concatenate Strings(w1040, "故障中止") -> (w1039:string)
                            }
                          }
                        }
                      }
                    }
                    frame "English" {
                      n843 = case shown="0, 默认" w1045 {
                        tunnel: w1044 -> [_ w1049 w1057 w1065]
                        tunnel: [w1046 w1048 w1056 w1064] -> w1043
                        tunnel: w1042 -> [w1046 w1047 w1055 w1063]
                        frame 0, Default {
                        }
                        frame 1 {
                          n844 = case shown="1" w1049 {
                            tunnel: [w1050 w1051] -> w1048
                            tunnel: w1047 -> [w1050 w1053]
                            frame 0, Default {
                            }
                            frame 1 {
                              n845 = Concatenate Strings(w1053, "To set the conditions", "\n") -> (w1051:string)
                            }
                          }
                        }
                        frame 2 {
                          n846 = case shown="1" w1057 {
                            tunnel: [w1058 w1059] -> w1056
                            tunnel: w1055 -> [w1058 w1061]
                            frame 0, Default {
                            }
                            frame 1 {
                              n847 = Concatenate Strings(w1061, "Artificial abort", "\n") -> (w1059:string)
                            }
                          }
                        }
                        frame 3 {
                          n848 = case shown="1" w1065 {
                            tunnel: [w1066 w1067] -> w1064
                            tunnel: w1063 -> [w1066 w1068]
                            frame 0, Default {
                            }
                            frame 1 {
                              n849 = Concatenate Strings(w1068, "Fault termination") -> (w1067:string)
                            }
                          }
                        }
                      }
                    }
                  }
                }
                n850 = call <vilib>:"Trim Whitespace.vi"("string"=w830) -> ("trimmed string"=w821:string)  [unwired: 1 in]
                n851 = Concatenate Strings(w826, w825) -> (w824:string)
                n852 = local write "充电机中止充电原因"(w821) -> ()
                n853 = call <vilib>:"Trim Whitespace.vi"("string"=w824) -> ("trimmed string"=w820:string)  [unwired: 1 in]
                n854 = local write "充电机 故障代码"(w820) -> ()
              }
              frame #1 {
                w1185 = "" ("trimmed string")
                n855 = call "二进制解析-8.6.vi"("索引"=8, "数值"=w1187) -> ("低位子数组"=w1186:i32[])  [unwired: 3 out]
                n856 = call "二进制解析-8.6.vi"("索引"=8, "数值"=w1190) -> ("低位子数组"=w1191:i32[])  [unwired: 3 out]
                n857 = call "二进制解析-8.6.vi"("索引"=8, "数值"=w1189) -> ("低位子数组"=w1193:i32[])  [unwired: 3 out]
                n858 = for {
                  N: 8 -> [_]
                  tunnel: w1191 -> [w1204]
                  shift-right: [w1200] -> w1184
                  shift-left: w1185 -> [w1199]
                  tunnel: w1177 -> [w1196]
                  i -> [w1198]
                  n859 = Reverse 1D Array(array=w1204) -> (reversed array=w1197:i32[])
                  n860 = Array Subset(array=w1197, index=w1198, length=1 ("y")) -> (w1203:i32[])
                  n861 = call "数值二进制转十进制-8.6.vi"("子数组"=w1203) -> ("十进制数值"=w1202:i32)  [unwired: 4 out]
                  n862 = case shown="\"English\"" w1196 {
                    tunnel: w1202 -> [w1208 w1252]
                    tunnel: [w1207 w1251] -> w1200
                    tunnel: w1199 -> [w1206 w1250]
                    tunnel: w1198 -> [w1205 w1249]
                    frame "中文", Default {
                      n863 = case shown="7" w1205 {
                        tunnel: w1208 -> [_ w1212 w1220 w1228 w1236 w1244]
                        tunnel: [w1209 w1211 w1219 w1227 w1235 w1243] -> w1207
                        tunnel: w1206 -> [w1209 w1210 w1218 w1226 w1234 w1242]
                        frame 0, Default {
                        }
                        frame 3 {
                          n864 = case shown="1" w1212 {
                            tunnel: [w1213 w1214] -> w1211
                            tunnel: w1210 -> [w1213 w1216]
                            frame 0, Default {
                            }
                            frame 1 {
                              n865 = Concatenate Strings(w1216, "其他故障", "\n") -> (w1214:string)
                            }
                          }
                        }
                        frame 4 {
                          n866 = case shown="1" w1220 {
                            tunnel: [w1221 w1222] -> w1219
                            tunnel: w1218 -> [w1221 w1224]
                            frame 0, Default {
                            }
                            frame 1 {
                              n867 = Concatenate Strings(w1224, "烟雾报警", "\n") -> (w1222:string)
                            }
                          }
                        }
                        frame 5 {
                          n868 = case shown="1" w1228 {
                            tunnel: [w1229 w1230] -> w1227
                            tunnel: w1226 -> [w1229 w1232]
                            frame 0, Default {
                            }
                            frame 1 {
                              n869 = Concatenate Strings(w1232, "辅助电源故障", "\n") -> (w1230:string)
                            }
                          }
                        }
                        frame 6 {
                          n870 = case shown="1" w1236 {
                            tunnel: [w1237 w1238] -> w1235
                            tunnel: w1234 -> [w1237 w1240]
                            frame 0, Default {
                            }
                            frame 1 {
                              n871 = Concatenate Strings(w1240, "充电通信超时", "\n") -> (w1238:string)
                            }
                          }
                        }
                        frame 7 {
                          n872 = case shown="1" w1244 {
                            tunnel: [w1245 w1246] -> w1243
                            tunnel: w1242 -> [w1245 w1247]
                            frame 0, Default {
                            }
                            frame 1 {
                              n873 = Concatenate Strings(w1247, "充电连接器故障") -> (w1246:string)
                            }
                          }
                        }
                      }
                    }
                    frame "English" {
                      n874 = case shown="7" w1249 {
                        tunnel: w1252 -> [_ w1256 w1264 w1272 w1280 w1288]
                        tunnel: [w1253 w1255 w1263 w1271 w1279 w1287] -> w1251
                        tunnel: w1250 -> [w1253 w1254 w1262 w1270 w1278 w1286]
                        frame 0, Default {
                        }
                        frame 3 {
                          n875 = case shown="1" w1256 {
                            tunnel: [w1257 w1258] -> w1255
                            tunnel: w1254 -> [w1257 w1260]
                            frame 0, Default {
                            }
                            frame 1 {
                              n876 = Concatenate Strings(w1260, "Other faults", "\n") -> (w1258:string)
                            }
                          }
                        }
                        frame 4 {
                          n877 = case shown="1" w1264 {
                            tunnel: [w1265 w1266] -> w1263
                            tunnel: w1262 -> [w1265 w1268]
                            frame 0, Default {
                            }
                            frame 1 {
                              n878 = Concatenate Strings(w1268, "Smoke alarm", "\n") -> (w1266:string)
                            }
                          }
                        }
                        frame 5 {
                          n879 = case shown="1" w1272 {
                            tunnel: [w1273 w1274] -> w1271
                            tunnel: w1270 -> [w1273 w1276]
                            frame 0, Default {
                            }
                            frame 1 {
                              n880 = Concatenate Strings(w1276, "Auxiliary power supply failure", "\n") -> (w1274:string)
                            }
                          }
                        }
                        frame 6 {
                          n881 = case shown="1" w1280 {
                            tunnel: [w1281 w1282] -> w1279
                            tunnel: w1278 -> [w1281 w1284]
                            frame 0, Default {
                            }
                            frame 1 {
                              n882 = Concatenate Strings(w1284, "Charging communication timeout", "\n") -> (w1282:string)
                            }
                          }
                        }
                        frame 7 {
                          n883 = case shown="1" w1288 {
                            tunnel: [w1289 w1290] -> w1287
                            tunnel: w1286 -> [w1289 w1291]
                            frame 0, Default {
                            }
                            frame 1 {
                              n884 = Concatenate Strings(w1291, "The charging connector fault") -> (w1290:string)
                            }
                          }
                        }
                      }
                    }
                  }
                }
                n885 = for {
                  N: 8 -> [_]
                  tunnel: w1193 -> [w1446]
                  shift-right: [w1442] -> w1192
                  shift-left: w1185 -> [w1441]
                  tunnel: w1177 -> [w1438]
                  i -> [w1440]
                  n886 = Reverse 1D Array(array=w1446) -> (reversed array=w1439:i32[])
                  n887 = Array Subset(array=w1439, index=w1440, length=1 ("y")) -> (w1445:i32[])
                  n888 = call "数值二进制转十进制-8.6.vi"("子数组"=w1445) -> ("十进制数值"=w1444:i32)  [unwired: 4 out]
                  n889 = case shown="\"English\"" w1438 {
                    tunnel: w1444 -> [w1450 w1518]
                    tunnel: [w1449 w1517] -> w1442
                    tunnel: w1441 -> [w1448 w1516]
                    tunnel: w1440 -> [w1447 w1515]
                    frame "中文", Default {
                      n890 = case shown="0, 默认" w1447 {
                        tunnel: w1450 -> [w1453 w1461 w1469 w1477 w1485 w1493 w1501 w1509]
                        tunnel: [w1452 w1460 w1468 w1476 w1484 w1492 w1500 w1508] -> w1449
                        tunnel: w1448 -> [w1451 w1459 w1467 w1475 w1483 w1491 w1499 w1507]
                        frame 0, Default {
                          n891 = case shown="1" w1453 {
                            tunnel: [w1454 w1455] -> w1452
                            tunnel: w1451 -> [w1454 w1457]
                            frame 0, Default {
                            }
                            frame 1 {
                              n892 = Concatenate Strings(w1457, "输出连接器故障", "\n") -> (w1455:string)
                            }
                          }
                        }
                        frame 1 {
                          n893 = case shown="1" w1461 {
                            tunnel: [w1462 w1463] -> w1460
                            tunnel: w1459 -> [w1462 w1465]
                            frame 0, Default {
                            }
                            frame 1 {
                              n894 = Concatenate Strings(w1465, "充电继电器故障", "\n") -> (w1463:string)
                            }
                          }
                        }
                        frame 2 {
                          n895 = case shown="1" w1469 {
                            tunnel: [w1470 w1471] -> w1468
                            tunnel: w1467 -> [w1470 w1473]
                            frame 0, Default {
                            }
                            frame 1 {
                              n896 = Concatenate Strings(w1473, "电池己充满", "\n") -> (w1471:string)
                            }
                          }
                        }
                        frame 3 {
                          n897 = case shown="1" w1477 {
                            tunnel: [w1478 w1479] -> w1476
                            tunnel: w1475 -> [w1478 w1481]
                            frame 0, Default {
                            }
                            frame 1 {
                              n898 = Concatenate Strings(w1481, "电池不匹配", "\n") -> (w1479:string)
                            }
                          }
                        }
                        frame 4 {
                          n899 = case shown="1" w1485 {
                            tunnel: [w1486 w1487] -> w1484
                            tunnel: w1483 -> [w1486 w1489]
                            frame 0, Default {
                            }
                            frame 1 {
                              n900 = Concatenate Strings(w1489, "充电电流超限", "\n") -> (w1487:string)
                            }
                          }
                        }
                        frame 5 {
                          n901 = case shown="1" w1493 {
                            tunnel: [w1494 w1495] -> w1492
                            tunnel: w1491 -> [w1494 w1497]
                            frame 0, Default {
                            }
                            frame 1 {
                              n902 = Concatenate Strings(w1497, "电池温度过低", "\n") -> (w1495:string)
                            }
                          }
                        }
                        frame 6 {
                          n903 = case shown="1" w1501 {
                            tunnel: [w1502 w1503] -> w1500
                            tunnel: w1499 -> [w1502 w1505]
                            frame 0, Default {
                            }
                            frame 1 {
                              n904 = Concatenate Strings(w1505, "电池温度过高", "\n") -> (w1503:string)
                            }
                          }
                        }
                        frame 7 {
                          n905 = case shown="1" w1509 {
                            tunnel: [w1510 w1512] -> w1508
                            tunnel: w1507 -> [w1510 w1513]
                            frame 0, Default {
                            }
                            frame 1 {
                              n906 = Concatenate Strings(w1513, "总电压过低", "\n") -> (w1512:string)
                            }
                          }
                        }
                      }
                    }
                    frame "English" {
                      n907 = case shown="0, 默认" w1515 {
                        tunnel: w1518 -> [w1521 w1529 w1537 w1545 w1553 w1561 w1569 w1577]
                        tunnel: [w1520 w1528 w1536 w1544 w1552 w1560 w1568 w1576] -> w1517
                        tunnel: w1516 -> [w1519 w1527 w1535 w1543 w1551 w1559 w1567 w1575]
                        frame 0, Default {
                          n908 = case shown="1" w1521 {
                            tunnel: [w1522 w1523] -> w1520
                            tunnel: w1519 -> [w1522 w1525]
                            frame 0, Default {
                            }
                            frame 1 {
                              n909 = Concatenate Strings(w1525, "The fault output connector", "\n") -> (w1523:string)
                            }
                          }
                        }
                        frame 1 {
                          n910 = case shown="1" w1529 {
                            tunnel: [w1530 w1531] -> w1528
                            tunnel: w1527 -> [w1530 w1533]
                            frame 0, Default {
                            }
                            frame 1 {
                              n911 = Concatenate Strings(w1533, "Charging relay fault", "\n") -> (w1531:string)
                            }
                          }
                        }
                        frame 2 {
                          n912 = case shown="1" w1537 {
                            tunnel: [w1538 w1539] -> w1536
                            tunnel: w1535 -> [w1538 w1541]
                            frame 0, Default {
                            }
                            frame 1 {
                              n913 = Concatenate Strings(w1541, "The battery is full of", "\n") -> (w1539:string)
                            }
                          }
                        }
                        frame 3 {
                          n914 = case shown="1" w1545 {
                            tunnel: [w1546 w1547] -> w1544
                            tunnel: w1543 -> [w1546 w1549]
                            frame 0, Default {
                            }
                            frame 1 {
                              n915 = Concatenate Strings(w1549, "The battery does not match", "\n") -> (w1547:string)
                            }
                          }
                        }
                        frame 4 {
                          n916 = case shown="1" w1553 {
                            tunnel: [w1554 w1555] -> w1552
                            tunnel: w1551 -> [w1554 w1557]
                            frame 0, Default {
                            }
                            frame 1 {
                              n917 = Concatenate Strings(w1557, "The charging current overload", "\n") -> (w1555:string)
                            }
                          }
                        }
                        frame 5 {
                          n918 = case shown="1" w1561 {
                            tunnel: [w1562 w1563] -> w1560
                            tunnel: w1559 -> [w1562 w1565]
                            frame 0, Default {
                            }
                            frame 1 {
                              n919 = Concatenate Strings(w1565, "The battery temperature is too low", "\n") -> (w1563:string)
                            }
                          }
                        }
                        frame 6 {
                          n920 = case shown="1" w1569 {
                            tunnel: [w1570 w1571] -> w1568
                            tunnel: w1567 -> [w1570 w1573]
                            frame 0, Default {
                            }
                            frame 1 {
                              n921 = Concatenate Strings(w1573, "The high temperature of the battery", "\n") -> (w1571:string)
                            }
                          }
                        }
                        frame 7 {
                          n922 = case shown="1" w1577 {
                            tunnel: [w1578 w1580] -> w1576
                            tunnel: w1575 -> [w1578 w1581]
                            frame 0, Default {
                            }
                            frame 1 {
                              n923 = Concatenate Strings(w1581, "The total voltage is too low", "\n") -> (w1580:string)
                            }
                          }
                        }
                      }
                    }
                  }
                }
                n924 = for {
                  N: 8 -> [_]
                  tunnel: w1186 -> [w1301]
                  shift-right: [w1297] -> w1183
                  shift-left: w1185 -> [w1296]
                  tunnel: w1177 -> [w1293]
                  i -> [w1295]
                  n925 = Reverse 1D Array(array=w1301) -> (reversed array=w1294:i32[])
                  n926 = Array Subset(array=w1294, index=w1295, length=1 ("y")) -> (w1300:i32[])
                  n927 = call "数值二进制转十进制-8.6.vi"("子数组"=w1300) -> ("十进制数值"=w1299:i32)  [unwired: 4 out]
                  n928 = case shown="\"English\"" w1293 {
                    tunnel: w1299 -> [w1305 w1373]
                    tunnel: [w1304 w1372] -> w1297
                    tunnel: w1296 -> [w1303 w1371]
                    tunnel: w1295 -> [w1302 w1370]
                    frame "中文", Default {
                      n929 = case shown="7" w1302 {
                        tunnel: w1305 -> [w1308 w1316 w1324 w1332 w1340 w1348 w1356 w1364]
                        tunnel: [w1307 w1315 w1323 w1331 w1339 w1347 w1355 w1363] -> w1304
                        tunnel: w1303 -> [w1306 w1314 w1322 w1330 w1338 w1346 w1354 w1362]
                        frame 0, Default {
                          n930 = case shown="1" w1308 {
                            tunnel: [w1309 w1310] -> w1307
                            tunnel: w1306 -> [w1309 w1312]
                            frame 0, Default {
                            }
                            frame 1 {
                              n931 = Concatenate Strings(w1312, "总电压超过上限", "\n") -> (w1310:string)
                            }
                          }
                        }
                        frame 1 {
                          n932 = case shown="1" w1316 {
                            tunnel: [w1317 w1318] -> w1315
                            tunnel: w1314 -> [w1317 w1320]
                            frame 0, Default {
                            }
                            frame 1 {
                              n933 = Concatenate Strings(w1320, "单体电压过低", "\n") -> (w1318:string)
                            }
                          }
                        }
                        frame 2 {
                          n934 = case shown="1" w1324 {
                            tunnel: [w1325 w1326] -> w1323
                            tunnel: w1322 -> [w1325 w1328]
                            frame 0, Default {
                            }
                            frame 1 {
                              n935 = Concatenate Strings(w1328, "单体电压超过上限", "\n") -> (w1326:string)
                            }
                          }
                        }
                        frame 3 {
                          n936 = case shown="1" w1332 {
                            tunnel: [w1333 w1334] -> w1331
                            tunnel: w1330 -> [w1333 w1336]
                            frame 0, Default {
                            }
                            frame 1 {
                              n937 = Concatenate Strings(w1336, "系统存在绝缘故障", "\n") -> (w1334:string)
                            }
                          }
                        }
                        frame 4 {
                          n938 = case shown="1" w1340 {
                            tunnel: [w1341 w1342] -> w1339
                            tunnel: w1338 -> [w1341 w1344]
                            frame 0, Default {
                            }
                            frame 1 {
                              n939 = Concatenate Strings(w1344, "BMS有硬件故障", "\n") -> (w1342:string)
                            }
                          }
                        }
                        frame 5 {
                          n940 = case shown="1" w1348 {
                            tunnel: [w1349 w1350] -> w1347
                            tunnel: w1346 -> [w1349 w1352]
                            frame 0, Default {
                            }
                            frame 1 {
                              n941 = Concatenate Strings(w1352, "达到所需SOC目标值", "\n") -> (w1350:string)
                            }
                          }
                        }
                        frame 6 {
                          n942 = case shown="1" w1356 {
                            tunnel: [w1357 w1358] -> w1355
                            tunnel: w1354 -> [w1357 w1360]
                            frame 0, Default {
                            }
                            frame 1 {
                              n943 = Concatenate Strings(w1360, "达到总电压设定值", "\n") -> (w1358:string)
                            }
                          }
                        }
                        frame 7 {
                          n944 = case shown="1" w1364 {
                            tunnel: [w1365 w1367] -> w1363
                            tunnel: w1362 -> [w1365 w1368]
                            frame 0, Default {
                            }
                            frame 1 {
                              n945 = Concatenate Strings(w1368, "达到所需单体电压设定值", "\n") -> (w1367:string)
                            }
                          }
                        }
                      }
                    }
                    frame "English" {
                      n946 = case shown="1" w1370 {
                        tunnel: w1373 -> [w1376 w1384 w1392 w1400 w1408 w1416 w1424 w1432]
                        tunnel: [w1375 w1383 w1391 w1399 w1407 w1415 w1423 w1431] -> w1372
                        tunnel: w1371 -> [w1374 w1382 w1390 w1398 w1406 w1414 w1422 w1430]
                        frame 0, Default {
                          n947 = case shown="1" w1376 {
                            tunnel: [w1377 w1378] -> w1375
                            tunnel: w1374 -> [w1377 w1380]
                            frame 0, Default {
                            }
                            frame 1 {
                              n948 = Concatenate Strings(w1380, "The total voltage exceeds the upper limit", "\n") -> (w1378:string)
                            }
                          }
                        }
                        frame 1 {
                          n949 = case shown="1" w1384 {
                            tunnel: [w1385 w1386] -> w1383
                            tunnel: w1382 -> [w1385 w1388]
                            frame 0, Default {
                            }
                            frame 1 {
                              n950 = Concatenate Strings(w1388, "Single voltage is too low", "\n") -> (w1386:string)
                            }
                          }
                        }
                        frame 2 {
                          n951 = case shown="1" w1392 {
                            tunnel: [w1393 w1394] -> w1391
                            tunnel: w1390 -> [w1393 w1396]
                            frame 0, Default {
                            }
                            frame 1 {
                              n952 = Concatenate Strings(w1396, "Single voltage exceeds the upper limit", "\n") -> (w1394:string)
                            }
                          }
                        }
                        frame 3 {
                          n953 = case shown="1" w1400 {
                            tunnel: [w1401 w1402] -> w1399
                            tunnel: w1398 -> [w1401 w1404]
                            frame 0, Default {
                            }
                            frame 1 {
                              n954 = Concatenate Strings(w1404, "System insulation fault", "\n") -> (w1402:string)
                            }
                          }
                        }
                        frame 4 {
                          n955 = case shown="1" w1408 {
                            tunnel: [w1409 w1410] -> w1407
                            tunnel: w1406 -> [w1409 w1412]
                            frame 0, Default {
                            }
                            frame 1 {
                              n956 = Concatenate Strings(w1412, "The BMS has a hardware failure", "\n") -> (w1410:string)
                            }
                          }
                        }
                        frame 5 {
                          n957 = case shown="1" w1416 {
                            tunnel: [w1417 w1418] -> w1415
                            tunnel: w1414 -> [w1417 w1420]
                            frame 0, Default {
                            }
                            frame 1 {
                              n958 = Concatenate Strings(w1420, "To achieve the required SOC target values", "\n") -> (w1418:string)
                            }
                          }
                        }
                        frame 6 {
                          n959 = case shown="1" w1424 {
                            tunnel: [w1425 w1426] -> w1423
                            tunnel: w1422 -> [w1425 w1428]
                            frame 0, Default {
                            }
                            frame 1 {
                              n960 = Concatenate Strings(w1428, "The total voltage setting value", "\n") -> (w1426:string)
                            }
                          }
                        }
                        frame 7 {
                          n961 = case shown="1" w1432 {
                            tunnel: [w1433 w1435] -> w1431
                            tunnel: w1430 -> [w1433 w1436]
                            frame 0, Default {
                            }
                            frame 1 {
                              n962 = Concatenate Strings(w1436, "To achieve the desired monomer voltage \nsetting value", "\n") -> (w1435:string)
                            }
                          }
                        }
                      }
                    }
                  }
                }
                n963 = Concatenate Strings(w1183, w1192, w1184) -> (w1182:string)
                n964 = call <vilib>:"Trim Whitespace.vi"("string"=w1182) -> ("trimmed string"=w1178:string)  [unwired: 1 in]
                n965 = local write "BMS中止\n充电原因"(w1178) -> ()
              }
            }
            n966 = global read "电池信息全局变量.vi" "充电机累计输出能量"() -> (w807:dbl)
            n967 = global read "电池信息全局变量.vi" "最小允许充电电流"() -> (w801:dbl)
            n968 = global read "电池信息全局变量.vi" "最大允许充电电流"() -> (w802:dbl)
            n969 = global read "电池信息全局变量.vi" "充电机输出电流"() -> (w805:dbl)
            n970 = global read "电池信息全局变量.vi" "充电机输出电压"() -> (w804:dbl)
            n971 = Format Into String(format string=w803, w804) -> (resulting string=w799:string)  [unwired: 2 in, 1 out]
            n972 = Format Into String(format string=w803, w805) -> (resulting string=w800:string)  [unwired: 2 in, 1 out]
            n973 = Format Into String(format string=w803, w807) -> (resulting string=w806:string)  [unwired: 2 in, 1 out]
            n974 = local write "最大允许充电电流(A)"(w802) -> ()
            n975 = local write "最小允许充电电流(A)"(w801) -> ()
            n976 = local write "充电机输出电压(V)"(w799) -> ()
            n977 = local write "充电机累计输出能量(kW)"(w806) -> ()
            n978 = local write "充电机输出电流(A)"(w800) -> ()
            n979 = global read "电池信息全局变量.vi" "最高允许充电单体电压"() -> (w811:dbl)
            n980 = global read "电池信息全局变量.vi" "最高允许充电总电压"() -> (w812:dbl)
            n981 = global read "电池信息全局变量.vi" "最高允许充电温度"() -> (w813:dbl)
            n982 = global read "电池信息全局变量.vi" "累计充电时间"() -> (w810:dbl)
            n983 = global read "电池信息全局变量.vi" "剩余充电时间"() -> (w809:dbl)
            n984 = global read "电池信息全局变量.vi" "充电电流步长"() -> (w808:dbl)
            n985 = local write "充电电流步长"(w808) -> ()
            n986 = local write "累计充电时间(min)"(w810) -> ()
            n987 = local write "剩余充电时间(min)"(w809) -> ()
            n988 = local write "最高允许充电单体电压(A)"(w811) -> ()
            n989 = local write "最高允许充电总电压(A)"(w812) -> ()
            n990 = local write "最高允许充电温度(℃)"(w813) -> ()
          }
        }
      }
      n991 = property on="电池故障显示" class="Bool (严格)"("Visible"=w209, "Value"=FALSE ("电池故障显示")) -> ()  [unwired: 2 in, 2 out]
      n992 = property on="电池系统故障显示" class="Bool (严格)"("Visible"=w209, "Value"=w209) -> ()  [unwired: 2 in, 2 out]
      n993 = property on="BMS故障显示" class="Bool (严格)"("Visible"=w209, "Value"=w209) -> ()  [unwired: 2 in, 2 out]
      n994 = property on="其他故障显示" class="Bool (严格)"("Visible"=w209, "Value"=w209) -> ()  [unwired: 2 in, 2 out]
      n995 = property on="二级故障 2" class="Bool (严格)"("Visible"=w210, "Value"=FALSE ("二级故障 2")) -> ()  [unwired: 2 in, 2 out]
      n996 = property on="二级故障 3" class="Bool (严格)"("Visible"=w210, "Value"=w210) -> ()  [unwired: 2 in, 2 out]
      n997 = property on="二级故障 4" class="Bool (严格)"("Visible"=w210, "Value"=w210) -> ()  [unwired: 2 in, 2 out]
      n998 = property on="二级故障 5" class="Bool (严格)"("Visible"=w210, "Value"=w210) -> ()  [unwired: 2 in, 2 out]
      "单选选项2" <- FALSE ("单选选项2")
    }
  }
